vi "TILDAS Prep Line Valves Sequence - 6June22.vi"() -> ()   [LabVIEW 2020]
uses:
  <vilib>/Analysis/baseanly.llb/Mean (DBL).vi
  <vilib>/MakerHub/LINX/Public/Peripherals/Digital/Digital Write 1 Chan.vi
  <vilib>/MakerHub/LINX/Public/Peripherals/Digital/Digital Write N Chans.vi
  <vilib>/MakerHub/LINX/Private/Local IO/LinxDigitalWrite.vi
  <vilib>/MakerHub/LINX/Public/Utilities/Check Channel.vi
  <vilib>/MakerHub/LINX/Public/Utilities/Open Serial.vi
  <vilib>/MakerHub/LINX/Private/Utilties/Generate Error.vi
  <vilib>/MakerHub/LINX/LMH-LINX.lvlib
  <vilib>/Analysis/NI_AALBase.lvlib
panel:
  in  "Stop Loop Fill":bool
  out "Prep. Loop":bool
  in  "Circulation Loop":bool
  in  "Circulation Loop":u8=17
  out "Slosh acc. %":dbl
  out "P frac. slosh":dbl
  out "Rem. slosh frac.":dbl
  out "Exact slosh":dbl
  out "Slosh P (mbar)":dbl
  out "Slosh to do":dbl
  out "No. Slosh":dbl
  out "Final P Accuracy (%)":dbl
  in  "Stop Sample Pressure":bool
  out "Final P (mbar)":dbl
  out "Final Target P (mbar)":dbl
  out "Seq. Finished":bool
  out "Inject GB":bool
  in  "Test":bool
  in  "Stop Pump Over":bool
  out "umol CO2":dbl format="%0.3f"
  out "Dil. Target P (mbar)":dbl format="%0.3f"
  out "Thawing":bool
  out "Diluting":bool
  out "Cryo-pull":bool
  out "Dilution P (mbar)":dbl
  in  "Stop Dilution":bool
  out "Dil. i":i32
  in  "Valve 2":u8=2
  in  "V2":bool
  in  "Valve 3":u8=3
  in  "V3":bool
  in  "Valve 1":u8=4
  in  "V1":bool
  in  "Valve 5":u8=5
  in  "V5":bool
  in  "Valve 6":u8=6
  in  "V6":bool
  in  "Valve 4":u8=7
  in  "V4":bool
  in  "Valve 16":u8=8
  in  "V16":bool
  in  "Valve 8":u8=10
  in  "V8":bool
  in  "Dewar":u8=11
  in  "D":bool
  in  "Valve 19":u8=12
  in  "V19":bool
  in  "Valve 7":u8=13
  in  "V7":bool
  in  "Valve 18":u8=14
  in  "V18":bool
  in  "Valve 17":u8=16
  in  "V21":bool
  in  "Valve 21":u8=15
  in  "V17":bool
  in  "Valve 20":u8=17
  in  "V20":bool
  in  "stop (F)":bool caption="Gauge Signal"
  out "Wika (Avg)":dynamicdata(graph)
  out "?":dbl(knob) scale=0.001..1000.0
  out "?":dynamicdata(graph)
  out "Agilent":dbl(knob) scale=0.001..10.0
  out "Agilent (Torr)":dbl
  out "Pressure (mbar)":dbl format="%0.3f"
  out "V":dbl format="%#_4g"
  out "Thaw Yield (torr)":dbl
  out "Open Flask":bool
  out "Break Tube":bool
  in  "Temp (K)":dbl
  out "Analysis Start Time":timestamp format="%<%H:%M:%S\n%x>T"
  out "Current Time":timestamp format="%<%H:%M:%S>T"
  in  "End Program":bool caption="Press & Hold"
  in  "GO!!!!":bool
  in  "Cracker 3":bool
  in  "Cracker 2":bool
  in  "Cracker 1":bool
  in  "Standby Mode":bool
  out "Cracker":bool
  in  "Cracker Enabled":bool
  in  "Flask Enabled":bool
  in  "Carbonate Enabled":bool
  out "Atm Flask":bool
  out "Carbonate Sam":bool
  in  "Start Sequence":bool
  # "List of proper DO channel values: \nV1 - 4\nV2 - 2                     Slosh stats\nV3 - 3\nV4 - 7\nV5 - 5\nV6 - 6\nV7 - 13\nV8 - 10\nDewar - 11\nV16 - 8\nV17 - 15\nV18 - 14\nV19 - 12\nV20 - 17\nV21 - 16\nCirculation Loop - 9"
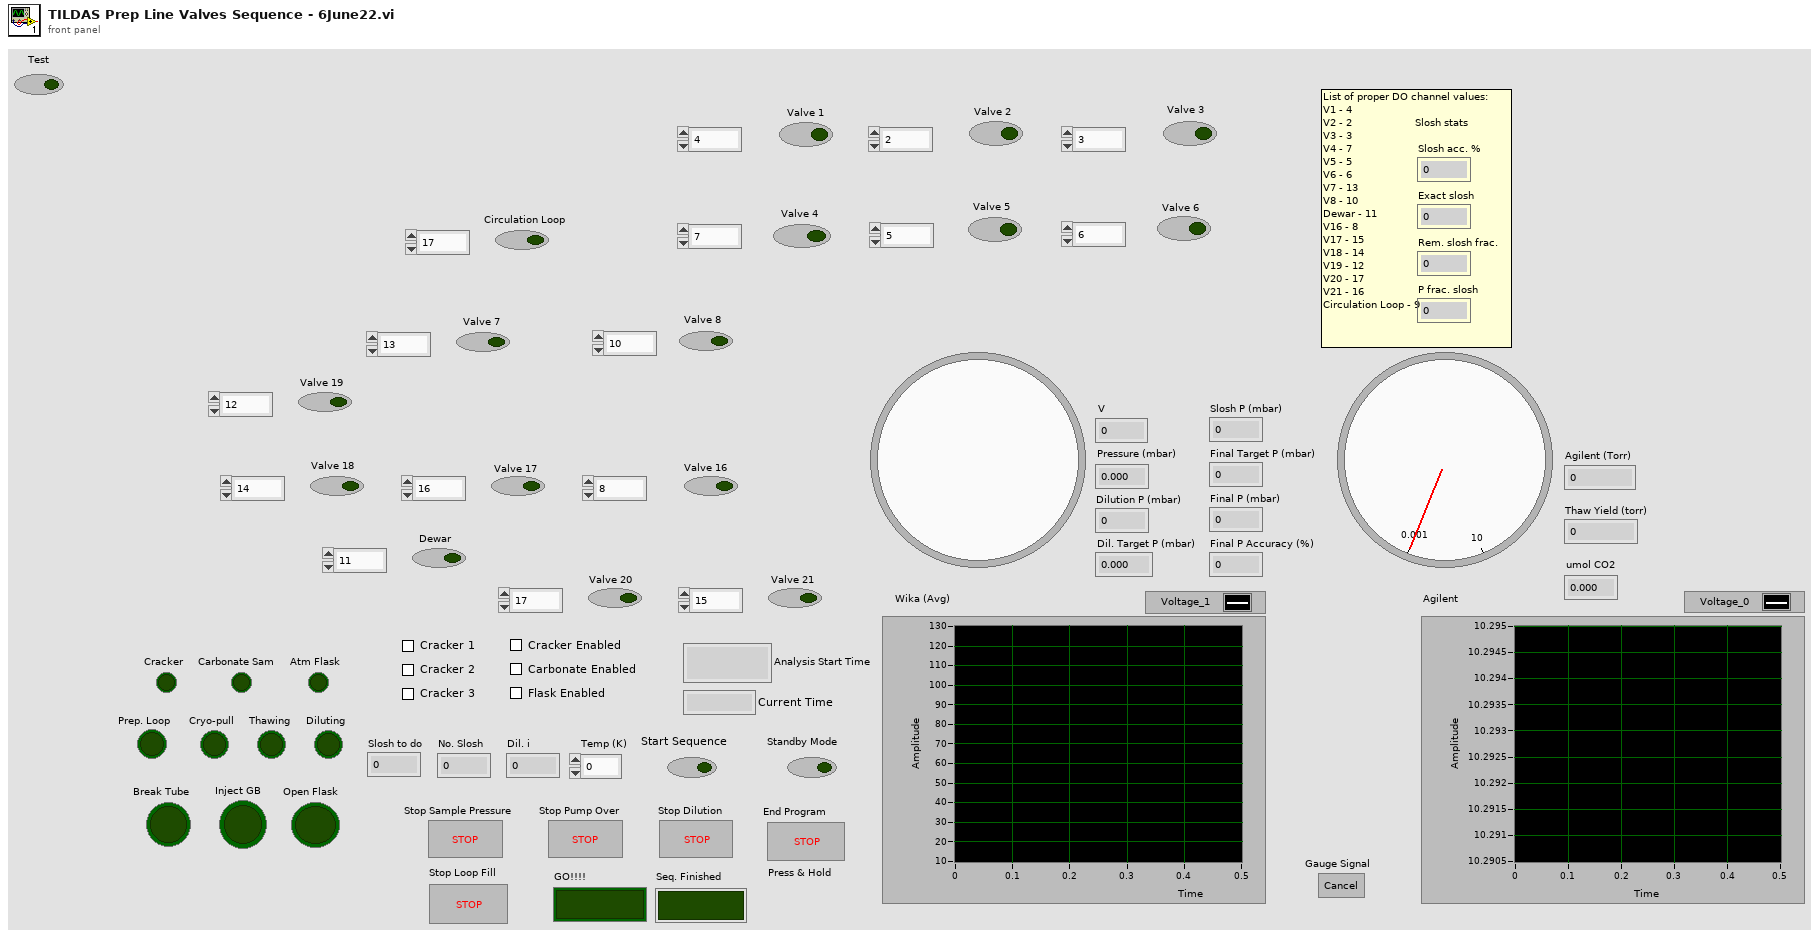
[diagram p1: front panel]
types:
  T1 = typedef "LMH-LINX.lvlib/LINX Ref.ctl" = cluster{"IO":T2, "Interface":T3, "LINX Device Config":T4}
  T2 = typedef "LMH-LINX.lvlib/Platform.ctl" = enum16{"Remote", "Local"}
  T3 = typedef "LMH-LINX.lvlib/Interface.ctl" = enum16{"Serial", "TCP"}
  T4 = typedef "LMH-LINX.lvlib/Device.lvlib/LINX Device Config.ctl" = cluster{"Interface":T3, "COM Port":refnum<visa-resource-name>, "TCP Configuration":T5, "Device Family":u8, "Device ID":u8, "Device Name":string, "TCP Ref":refnum<k5>, "Channels":T6}
  T5 = typedef "LMH-LINX.lvlib/Device.lvlib/TCP Config.ctl" = cluster{"IP Address":string, "Port":u16}
  T6 = typedef "LMH-LINX.lvlib/Channels.ctl" = cluster{"DI":u8[], "DO":u8[], "AI":u8[], "AO":u8[], "PWM":u8[], "QE":u8[], "UART":u8[], "I2C 2":u8[], "SPI":u8[], "CAN":u8[], "Servo":u8[], "AI Ref (V)":dbl, "AI Resolution (Bits)":u8, "AO Ref (V)":dbl, "AO Resolution (Bits)":u8}
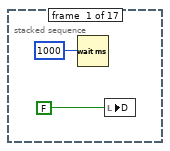
[diagram p6: hidden frame]
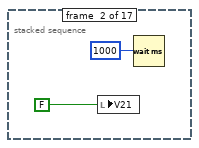
[diagram p7: hidden frame]
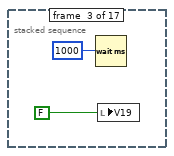
[diagram p8: hidden frame]
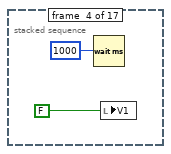
[diagram p9: hidden frame]
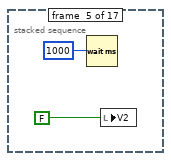
[diagram p10: hidden frame]
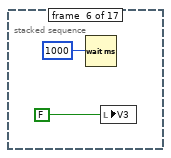
[diagram p11: hidden frame]
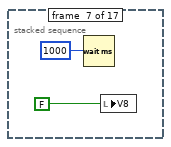
[diagram p12: hidden frame]
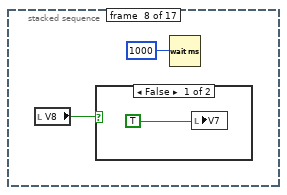
[diagram p13: hidden frame]
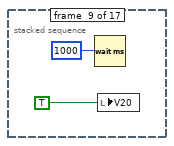
[diagram p15: hidden frame]
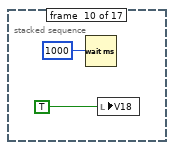
[diagram p16: hidden frame]
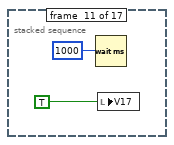
[diagram p17: hidden frame]
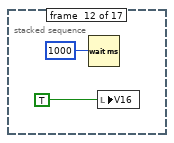
[diagram p18: hidden frame]
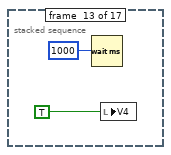
[diagram p19: hidden frame]
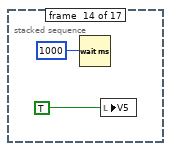
[diagram p20: hidden frame]
diagram:
  # "Standby mode: \nV21 - C\nV19 - C\nV1 - C\nV2 - C\nV3 - C\nV8 - C\nV7 - O\nV20 - O\nV18 - O\nV17 - O\nV16 - O\nV4 - O\nV5 - O\nV6 - O\nTurn off all \nindicators/controls"
  n1 = control-ref of="Standby Mode"() -> (w18:refnum<vi>)
  n2 = register-events(w18) -> (reference out=w17:refnum<event-registration>, error out=w7:errorcluster)  [unwired: 2 in]
  n3 = while {
    tunnel: w17 -> [w29]
    tunnel: [w28] -> w16
    tunnel: w7 -> [w25]
    tunnel: [w25] -> w8
    stop <- w26 stop-if-true
    n4 = event shown="[0] \"Standby Mode\": Value Change" {
      selector: w29 -> [_]
      dyn-events: [_] -> w28
      timeout: _ -> [_]
      event "Standby Mode": Value Change {
        n5 = event-data() -> ()  [unwired: 1 in, 6 out]
        n6 = stacked-sequence {
          frame #0 {
            n7 = Wait (ms)(milliseconds to wait=1000) -> ()  [unwired: 1 out]
            n8 = local write "D"(FALSE) -> ()
          }
          frame #1 {
            n9 = local write "V21"(FALSE) -> ()
            n10 = Wait (ms)(milliseconds to wait=1000) -> ()  [unwired: 1 out]
          }
          frame #2 {
            n11 = Wait (ms)(milliseconds to wait=1000) -> ()  [unwired: 1 out]
            n12 = local write "V19"(FALSE) -> ()
          }
          frame #3 {
            n13 = Wait (ms)(milliseconds to wait=1000) -> ()  [unwired: 1 out]
            n14 = local write "V1"(FALSE) -> ()
          }
          frame #4 {
            n15 = Wait (ms)(milliseconds to wait=1000) -> ()  [unwired: 1 out]
            n16 = local write "V2"(FALSE) -> ()
          }
          frame #5 {
            n17 = Wait (ms)(milliseconds to wait=1000) -> ()  [unwired: 1 out]
            n18 = local write "V3"(FALSE) -> ()
          }
          frame #6 {
            n19 = Wait (ms)(milliseconds to wait=1000) -> ()  [unwired: 1 out]
            n20 = local write "V8"(FALSE) -> ()
          }
          frame #7 {
            n21 = local read "V8"() -> (w45:bool)
            n22 = case shown="False" w45 {
              frame False {
                n23 = local write "V7"(TRUE) -> ()
              }
              frame True {
              }
            }
            n24 = Wait (ms)(milliseconds to wait=1000) -> ()  [unwired: 1 out]
          }
          frame #8 {
            n25 = Wait (ms)(milliseconds to wait=1000) -> ()  [unwired: 1 out]
            n26 = local write "V20"(TRUE) -> ()
          }
          frame #9 {
            n27 = Wait (ms)(milliseconds to wait=1000) -> ()  [unwired: 1 out]
            n28 = local write "V18"(TRUE) -> ()
          }
          frame #10 {
            n29 = Wait (ms)(milliseconds to wait=1000) -> ()  [unwired: 1 out]
            n30 = local write "V17"(TRUE) -> ()
          }
          frame #11 {
            n31 = Wait (ms)(milliseconds to wait=1000) -> ()  [unwired: 1 out]
            n32 = local write "V16"(TRUE) -> ()
          }
          frame #12 {
            n33 = Wait (ms)(milliseconds to wait=1000) -> ()  [unwired: 1 out]
            n34 = local write "V4"(TRUE) -> ()
          }
          frame #13 {
            n35 = Wait (ms)(milliseconds to wait=1000) -> ()  [unwired: 1 out]
            n36 = local write "V5"(TRUE) -> ()
          }
          frame #14 {
            n37 = Wait (ms)(milliseconds to wait=1000) -> ()  [unwired: 1 out]
            n38 = local write "V6"(TRUE) -> ()
          }
          frame #15 {
            w61 = FALSE
            n39 = local write "Break Tube"(w61) -> ()
            n40 = local write "Start Sequence"(w61) -> ()
            n41 = local write "Carbonate Enabled"(w61) -> ()
            n42 = local write "Flask Enabled"(w61) -> ()
            n43 = local write "Standby Mode"(w61) -> ()
            n44 = local write "Open Flask"(w61) -> ()
            n45 = local write "Cracker Enabled"(w61) -> ()
            n46 = local write "Carbonate Sam"(w61) -> ()
            n47 = local write "Cracker 1"(w61) -> ()
            n48 = local write "Atm Flask"(w61) -> ()
            n49 = local write "Cracker 2"(w61) -> ()
            n50 = local write "Cracker 3"(w61) -> ()
            n51 = local write "Cracker"(w61) -> ()
            n52 = local write "GO!!!!"(w61) -> ()
          }
          frame #16 {
            n53 = local write "Dil. Target P (mbar)"(0.0 ("Target P (mbar)")) -> ()
            n54 = local write "umol CO2"(0.0 ("umol CO2")) -> ()
            n55 = local write "Thaw Yield (torr)"(0.0 ("Thaw Yield (torr)")) -> ()
            n56 = local write "Dilution P (mbar)"(0.0 ("Dilution P (mbar)")) -> ()
            n57 = local write "Dil. i"(0 ("Dil. i")) -> ()
          }
        }
      }
    }
    n58 = Wait (ms)(milliseconds to wait=u32 111) -> ()  [unwired: 1 out]
    n59 = local read "End Program"() -> (w26:bool)
  }
  n60 = control-ref of="Start Sequence"() -> (w12:refnum<vi>)
  n61 = register-events(w12) -> (reference out=w13:refnum<event-registration>, error out=w9:errorcluster)  [unwired: 2 in]
  n62 = Unregister For Events(event registration refnum=w16, error in=w8) -> (error out=w15:errorcluster)
  n63 = call <vilib>:"Simple Error Handler.vi"("error in (no error)"=w15) -> ()  [unwired: 4 in, 5 out]
  n64 = call-poly <vilib>:"Open.vi"("Serial Port"=refnum<visa-resource-name> "COM3") -> ("Error Out"=w23:errorcluster, "LINX Resource"=w22:T1)  [unwired: 8 in, 1 out]
  n65 = while {
    tunnel: w13 -> [w70]
    tunnel: [w69] -> w11
    tunnel: w9 -> [w68]
    tunnel: [w67] -> w10
    stop <- w71 stop-if-true
    n66 = event shown="[0] \"Start Sequence\": Value Change" {
      selector: w70 -> [_]
      dyn-events: [_] -> w69
      timeout: _ -> [_]
      tunnel: w68 -> [w73]
      tunnel: [w73] -> w67
      event "Start Sequence": Value Change {
        # "Just lights - used to verify start of sequence"
        # "Atm flask sequence"
        # "Carbonate sequence"
        # "Crackers sequence"
        n67 = event-data() -> ()  [unwired: 1 in, 6 out]
        n68 = local read "Carbonate Enabled"() -> (w87:bool)
        n69 = local read "Flask Enabled"() -> (w86:bool)
        n70 = local read "Cracker Enabled"() -> (w84:bool)
        n71 = local read "Carbonate Enabled"() -> (w79:bool)
        n72 = local read "Cracker Enabled"() -> (w80:bool)
        n73 = local read "Start Sequence"() -> (w82:bool)
        n74 = local read "Flask Enabled"() -> (w78:bool)
        n75 = Or(x=w87, y=w86) -> (x .or. y?=w85:bool)
        n76 = Or(x=w84, y=w85) -> (x .or. y?=w83:bool)
        n77 = And(x=w82, y=w83) -> (x .and. y?=w81:bool)
        n78 = case shown="True" w80 {
          frame False {
          }
          frame True {
            n79 = local write "Carbonate Sam"(FALSE) -> ()
            n80 = local write "Atm Flask"(FALSE) -> ()
            n81 = local write "Cracker"(TRUE) -> ()
          }
        }
        n82 = case shown="True" w79 {
          frame False {
          }
          frame True {
            n83 = local write "Carbonate Sam"(TRUE) -> ()
            n84 = local write "Atm Flask"(FALSE) -> ()
            n85 = local write "Cracker"(FALSE) -> ()
          }
        }
        n86 = case shown="True" w78 {
          frame False {
          }
          frame True {
            n87 = local write "Carbonate Sam"(FALSE) -> ()
            n88 = local write "Atm Flask"(TRUE) -> ()
            n89 = local write "Cracker"(FALSE) -> ()
          }
        }
        n90 = case shown="True" w81 {
          selector: w81 -> [w1641 w1643]
          tunnel: [w1641 w1643] -> w74
          frame False {
            n91 = call "Display Message to User13"() -> ()  [unwired: 10 in, 2 out]
          }
          frame True {
            n92 = flat-sequence {
              frame #0 {
                n93 = Get Date/Time In Seconds() -> (seconds since 1Jan1904=→"Analysis Start Time":timestamp)
              }
              frame #1 {
                n94 = local write "GO!!!!"(TRUE) -> ()
              }
            }
            n95 = Wait (ms)(milliseconds to wait=u32 1000) -> ()  [unwired: 1 out]
          }
        }
        n96 = case shown="True" w74 {
          selector: w74 -> [w99 _]
          tunnel: [w99 w103] -> w76
          frame False {
          }
          frame True {
            n97 = local read "Carbonate Sam"() -> (w100:bool)
            n98 = local read "Start Sequence"() -> (w101:bool)
            n99 = And(x=w101, y=w100) -> (x .and. y?=w102:bool)
            n100 = case shown="True" w102 {
              tunnel: [w106 w107] -> w103
              frame False {
                n101 = local read "Carbonate Enabled"() -> (w104:bool)
                n102 = local read "GO!!!!"() -> (w105:bool)
                n103 = And(x=w105, y=w104) -> (x .and. y?=w106:bool)
              }
              frame True {
                n104 = local read "Carbonate Enabled"() -> (w108:bool)
                n105 = local read "GO!!!!"() -> (w109:bool)
                n106 = And(x=w109, y=w108) -> (x .and. y?=w107:bool)
              }
            }
          }
        }
        n107 = case shown="True" w74 {
          selector: w74 -> [w110 _]
          tunnel: [w110 w114] -> w75
          frame False {
          }
          frame True {
            n108 = local read "Start Sequence"() -> (w112:bool)
            n109 = local read "Cracker"() -> (w111:bool)
            n110 = And(x=w112, y=w111) -> (x .and. y?=w113:bool)
            n111 = case shown="True" w113 {
              tunnel: [w117 w118] -> w114
              frame False {
                n112 = local read "Carbonate Enabled"() -> (w115:bool)
                n113 = local read "GO!!!!"() -> (w116:bool)
                n114 = And(x=w116, y=w115) -> (x .and. y?=w117:bool)
              }
              frame True {
                n115 = local read "Cracker Enabled"() -> (w119:bool)
                n116 = local read "GO!!!!"() -> (w120:bool)
                n117 = And(x=w120, y=w119) -> (x .and. y?=w118:bool)
              }
            }
          }
        }
        n118 = case shown="True" w74 {
          selector: w74 -> [w88 _]
          tunnel: [w88 w92] -> w77
          frame False {
          }
          frame True {
            n119 = local read "Start Sequence"() -> (w90:bool)
            n120 = local read "Atm Flask"() -> (w89:bool)
            n121 = And(x=w90, y=w89) -> (x .and. y?=w91:bool)
            n122 = case shown="True" w91 {
              tunnel: [w95 w96] -> w92
              frame False {
                n123 = local read "Flask Enabled"() -> (w93:bool)
                n124 = local read "GO!!!!"() -> (w94:bool)
                n125 = And(x=w94, y=w93) -> (x .and. y?=w95:bool)
              }
              frame True {
                n126 = local read "Flask Enabled"() -> (w97:bool)
                n127 = local read "GO!!!!"() -> (w98:bool)
                n128 = And(x=w98, y=w97) -> (x .and. y?=w96:bool)
              }
            }
          }
        }
        n129 = case shown="True" w75 {
          frame False {
          }
          frame True {
            # "Pretty much if something is wrong from the start it won't pass this 2 second check and save the trouble of dealing with it"
            # "If Current Time is within a 2 second window of \nAnalysis Start Time, run this. If not, do nothing."
            n130 = local read "Analysis Start Time"() -> (w725:timestamp)
            n131 = local read "Current Time"() -> (w724:timestamp)
            n132 = To Double Precision Float(number=w725) -> (double precision float=w723:dbl)
            n133 = To Double Precision Float(number=w724) -> (double precision float=w726:dbl)
            n134 = Add(x=w723, y=2.0) -> (x+y=w728:dbl)
            n135 = Greater?(x=w726, y=w723) -> (0:w729:bool)
            n136 = Less?(x=w726, y=w728) -> (x < y?=w730:bool)
            n137 = And(x=w729, y=w730) -> (x .and. y?=w722:bool)
            n138 = case shown="True" w722 {
              frame False {
              }
              frame True {
                # "Cracker 1: V1-V4\nCracker 2: V2-V5\nCracker 3: V3-V6"
                # "Assuming stby start"
                # "Read cracker selected"
                # "Cracker 1: V1-V4\nCracker 2: V2-V5\nCracker 3: V3-V6"
                # "Assuming stby start"
                # "Read cracker selected"
                n139 = local read "Cracker 1"() -> (w731:bool)
                n140 = case shown="False" w731 {
                  frame False {
                    # "Cracker 1: V1-V4\nCracker 2: V2-V5\nCracker 3: V3-V6"
                    n141 = local read "Cracker 2"() -> (w732:bool)
                    n142 = case shown="False" w732 {
                      frame False {
                        # "Cracker 1: V1-V4\nCracker 2: V2-V5\nCracker 3: V3-V6"
                        n143 = local read "Cracker 3"() -> (w733:bool)
                        n144 = case shown="True" w733 {
                          frame False {
                            n145 = call "Display Message to User12"() -> ()  [unwired: 10 in, 2 out]
                          }
                          frame True {
                            n146 = stacked-sequence {
                              tunnel: [_ _ _ _ w759 _ _ _ _ _ _ _ _ _ _ _ _ _ _ _ _ _ _ _ _ _ _ _ _ _ _ _ _ _ _ _ _ _ _ _ _ _ _ _ _ _ _ _ _ _ _ _ _ _ _ _ _ _ _ _ _] -> _
                              tunnel: [_ _ _ _ _ _ _ _ _ _ _ _ _ _ _ _ w789 _ _ _ _ _ _ _ _ _ _ _ _ _ _ _ _ _ _ _ _ _ _ _ _ _ _ _ _ _ _ _ _ _ _ _ _ _ _ _ _ _ _ _ _] -> _
                              tunnel: [_ _ _ _ _ w760 _ _ _ _ _ _ _ _ _ _ _ _ _ _ _ _ _ _ _ _ _ _ _ _ _ _ _ _ _ _ _ _ _ _ _ _ _ _ _ _ _ _ _ _ _ _ _ _ _ _ _ _ _ _ _] -> _
                              tunnel: [_ _ _ _ _ _ _ _ _ _ _ _ _ _ _ _ _ _ _ _ _ _ _ _ _ _ _ _ _ _ _ _ _ _ _ _ _ _ _ _ _ _ _ _ _ _ _ _ _ _ _ _ _ _ _ _ w1024 _ _ _ _] -> _
                              tunnel: [_ _ _ _ _ _ _ _ _ _ _ _ _ _ _ _ _ _ _ _ _ _ _ _ _ _ _ _ _ _ _ _ _ _ _ _ _ _ _ _ _ _ _ _ _ _ _ _ _ _ _ _ _ _ _ _ _ _ w1027 _ _] -> _
                              frame #0 {
                                n147 = local write "Final Target P (mbar)"(0.0) -> ()
                                n148 = local write "Final P Accuracy (%)"(0.0) -> ()
                                n149 = local write "Thaw Yield (torr)"(0.0) -> ()
                                n150 = local write "Final P (mbar)"(0.0) -> ()
                                n151 = local write "Slosh to do"(0.0) -> ()
                                n152 = local write "umol CO2"(0.0) -> ()
                                n153 = local write "No. Slosh"(0.0) -> ()
                                n154 = local write "Dil. i"(0.0) -> ()
                                n155 = local write "Dil. Target P (mbar)"(0.0) -> ()
                                n156 = local write "Dilution P (mbar)"(0.0) -> ()
                                n157 = local write "Rem. slosh frac."(0.0) -> ()
                                n158 = local write "Slosh P (mbar)"(0.0) -> ()
                                n159 = local write "Slosh acc. %"(0.0) -> ()
                                n160 = local write "P frac. slosh"(0.0) -> ()
                                n161 = local write "Exact slosh"(0.0) -> ()
                                n162 = local write "Temp (K)"(294.0) -> ()
                              }
                              frame #1 {
                                # "V18,17,16,20 should all be open to start"
                                # "Open V7"
                                n163 = local write "V7"(TRUE) -> ()
                                n164 = local write "Seq. Finished"(FALSE) -> ()
                                n165 = Wait (ms)(milliseconds to wait=1000) -> ()  [unwired: 1 out]
                              }
                              frame #2 {
                                # "V18,17,16,20 should all be open to start"
                                # "Open V16"
                                n166 = local write "V16"(TRUE) -> ()
                                n167 = Wait (ms)(milliseconds to wait=1000) -> ()  [unwired: 1 out]
                              }
                              frame #3 {
                                # "Close off unselected crackers"
                                n168 = flat-sequence {
                                frame #0 {
                                n169 = local write "V4"(FALSE) -> ()
                                }
                                frame #1 {
                                n170 = Wait (ms)(milliseconds to wait=1000) -> ()  [unwired: 1 out]
                                }
                                frame #2 {
                                n171 = local write "V5"(FALSE) -> ()
                                }
                                }
                                n172 = Wait (ms)(milliseconds to wait=1000) -> ()  [unwired: 1 out]
                              }
                              frame #4 {
                                # "Close flask valves"
                                n173 = call "Prompt User for Input33"() -> ("OK"=w759:bool)  [unwired: 18 in, 1 out]
                              }
                              frame #5 {
                                # "Close crackers and GB manual valves"
                                n174 = call "Prompt User for Input34"() -> ("OK"=w760:bool)  [unwired: 18 in, 1 out]
                              }
                              frame #6 {
                                # "Open Loop"
                                n175 = local write "Circulation Loop"(TRUE) -> ()
                                n176 = local write "Prep. Loop"(TRUE) -> ()
                                n177 = Wait (ms)(milliseconds to wait=1000) -> ()  [unwired: 1 out]
                              }
                              frame #7 {
                                # "22/4/22 - background ~280 mtorr bg"
                                # "Pump Loop for 60sec"
                                n178 = call "Time Delay22"() -> ()  [unwired: 11 in, 1 out]
                              }
                              frame #8 {
                                # "Open V8"
                                n179 = local write "V8"(TRUE) -> ()
                                n180 = Wait (ms)(milliseconds to wait=1000) -> ()  [unwired: 1 out]
                              }
                              frame #9 {
                                # "Close V20"
                                n181 = local write "V20"(FALSE) -> ()
                                n182 = Wait (ms)(milliseconds to wait=1000) -> ()  [unwired: 1 out]
                              }
                              frame #10 {
                                # "Open V21"
                                n183 = local write "V21"(TRUE) -> ()
                                n184 = Wait (ms)(milliseconds to wait=1000) -> ()  [unwired: 1 out]
                              }
                              frame #11 {
                                # "When P > 1300 in Loop close V21"
                                n185 = while {
                                shift-right: [w771] -> _
                                shift-left: _ -> [_]
                                stop <- w772 stop-if-true
                                n186 = local read "Pressure (mbar)"() -> (w775:dbl)
                                n187 = Wait (ms)(milliseconds to wait=100) -> ()  [unwired: 1 out]
                                n188 = Greater?(x=w775, y=1300.0) -> (0:w774:bool)
                                n189 = case shown="True" w774 {
                                selector: w774 -> [w777 w780]
                                tunnel: [w777 w780] -> w771
                                frame False {
                                }
                                frame True {
                                n190 = local write "Stop Loop Fill"(TRUE) -> ()
                                n191 = local write "V21"(FALSE) -> ()
                                }
                                }
                                n192 = local read "Stop Loop Fill"() -> (w772:bool)
                                }
                                n193 = Wait (ms)(milliseconds to wait=1000) -> ()  [unwired: 1 out]
                              }
                              frame #12 {
                                n194 = call "Prompt User for Input35"() -> ()  [unwired: 18 in, 2 out]
                                n195 = local write "Stop Loop Fill"(FALSE) -> ()
                              }
                              frame #13 {
                                # "Shut Loop"
                                n196 = local write "Circulation Loop"(FALSE) -> ()
                                n197 = local write "Prep. Loop"(FALSE) -> ()
                                n198 = Wait (ms)(milliseconds to wait=1000) -> ()  [unwired: 1 out]
                              }
                              frame #14 {
                                # "Close V8"
                                n199 = local write "V8"(FALSE) -> ()
                                n200 = Wait (ms)(milliseconds to wait=1000) -> ()  [unwired: 1 out]
                              }
                              frame #15 {
                                # "Open V20"
                                n201 = local write "V20"(TRUE) -> ()
                                n202 = Wait (ms)(milliseconds to wait=1000) -> ()  [unwired: 1 out]
                              }
                              frame #16 {
                                # "Open crackers manual valve, close GB manual valve"
                                n203 = call "Prompt User for Input36"() -> ("OK"=w789:bool)  [unwired: 18 in, 1 out]
                              }
                              frame #17 {
                                # "Open V6 - pump out cracker to be used"
                                n204 = local write "V6"(TRUE) -> ()
                                n205 = Wait (ms)(milliseconds to wait=1000) -> ()  [unwired: 1 out]
                              }
                              frame #18 {
                                # "When P < 0,076 torr continue w/ sequence"
                                n206 = while {
                                shift-right: [w793] -> _
                                shift-left: _ -> [_]
                                stop <- w794 stop-if-true
                                n207 = local read "Agilent (Torr)"() -> (w797:dbl)
                                n208 = Wait (ms)(milliseconds to wait=100) -> ()  [unwired: 1 out]
                                n209 = Less?(x=w797, y=0.076) -> (x < y?=w796:bool)
                                n210 = case shown="True" w796 {
                                selector: w796 -> [w799 w801]
                                tunnel: [w799 w801] -> w793
                                frame False {
                                }
                                frame True {
                                n211 = local write "Stop Pump Over"(TRUE) -> ()
                                }
                                }
                                n212 = local read "Stop Pump Over"() -> (w794:bool)
                                }
                                n213 = Wait (ms)(milliseconds to wait=1000) -> ()  [unwired: 1 out]
                              }
                              frame #19 {
                                # "10 extra sec to pump out bottom cracker volume"
                                n214 = local write "Stop Pump Over"(FALSE) -> ()
                                n215 = Wait (ms)(milliseconds to wait=10000) -> ()  [unwired: 1 out]
                              }
                              frame #20 {
                                # "Redundant just in case"
                                # "Close V4"
                                n216 = local write "V4"(FALSE) -> ()
                                n217 = Wait (ms)(milliseconds to wait=1000) -> ()  [unwired: 1 out]
                              }
                              frame #21 {
                                # "Redundant just in case"
                                # "Close V5"
                                n218 = local write "V5"(FALSE) -> ()
                                n219 = Wait (ms)(milliseconds to wait=1000) -> ()  [unwired: 1 out]
                              }
                              frame #22 {
                                # "Dewar up"
                                n220 = local write "D"(TRUE) -> ()
                                n221 = Wait (ms)(milliseconds to wait=1000) -> ()  [unwired: 1 out]
                              }
                              frame #23 {
                                # "15 sec for trap to cool"
                                n222 = Wait (ms)(milliseconds to wait=15000) -> ()  [unwired: 1 out]
                              }
                              frame #24 {
                                # "Close V18"
                                n223 = local write "V18"(FALSE) -> ()
                                n224 = Wait (ms)(milliseconds to wait=1000) -> ()  [unwired: 1 out]
                              }
                              frame #25 {
                                # "Break tube light on"
                                n225 = local write "Break Tube"(TRUE) -> ()
                                n226 = Wait (ms)(milliseconds to wait=1000) -> ()  [unwired: 1 out]
                              }
                              frame #26 {
                                # "10 min cryo-pull"
                                n227 = local write "Cryo-pull"(TRUE) -> ()
                                n228 = call "Cryo pull t7"() -> ()  [unwired: 11 in, 1 out]
                              }
                              frame #27 {
                                # "Open V18 - pump over"
                                n229 = local write "V18"(TRUE) -> ()
                                n230 = Wait (ms)(milliseconds to wait=5000) -> ()  [unwired: 1 out]
                              }
                              frame #28 {
                                # "When P < 0.075 torr close LN2 trap"
                                n231 = while {
                                shift-right: [w820] -> _
                                shift-left: _ -> [_]
                                stop <- w822 stop-if-true
                                n232 = local read "Agilent (Torr)"() -> (w825:dbl)
                                n233 = Wait (ms)(milliseconds to wait=100) -> ()  [unwired: 1 out]
                                n234 = Less?(x=w825, y=0.075) -> (x < y?=w823:bool)
                                n235 = case shown="True" w823 {
                                selector: w823 -> [w826 w827]
                                tunnel: [w826 w827] -> w820
                                frame False {
                                }
                                frame True {
                                w829 = FALSE
                                n236 = local write "V17"(w829) -> ()
                                n237 = local write "V18"(w829) -> ()
                                n238 = local write "Stop Pump Over"(TRUE) -> ()
                                }
                                }
                                n239 = local read "Stop Pump Over"() -> (w822:bool)
                                }
                                n240 = local write "Cryo-pull"(FALSE) -> ()
                                n241 = Wait (ms)(milliseconds to wait=1000) -> ()  [unwired: 1 out]
                              }
                              frame #29 {
                                # "Close V16"
                                n242 = local write "Stop Pump Over"(FALSE) -> ()
                                n243 = local write "V16"(FALSE) -> ()
                                n244 = Wait (ms)(milliseconds to wait=1000) -> ()  [unwired: 1 out]
                              }
                              frame #30 {
                                # "Close V6"
                                n245 = local write "V6"(FALSE) -> ()
                                n246 = Wait (ms)(milliseconds to wait=1000) -> ()  [unwired: 1 out]
                              }
                              frame #31 {
                                # "Dewar down"
                                n247 = local write "D"(FALSE) -> ()
                                n248 = Wait (ms)(milliseconds to wait=1000) -> ()  [unwired: 1 out]
                              }
                              frame #32 {
                                # "6 minute thaw"
                                n249 = call "Time Delay23"() -> ()  [unwired: 11 in, 1 out]
                                n250 = local write "Thawing"(TRUE) -> ()
                                n251 = call "Display Message to User15"() -> ()  [unwired: 10 in, 2 out]
                              }
                              frame #33 {
                                n252 = call "Display Message to User16"() -> ()  [unwired: 10 in, 2 out]
                              }
                              frame #34 {
                                # "Read thaw P on Agilent - calculate umol CO2 trapped"
                                n253 = local write "Thawing"(FALSE) -> ()
                                n254 = flat-sequence {
                                frame #0 {
                                n255 = local read "Agilent (Torr)"() -> (w841:dbl)
                                n256 = local write "Thaw Yield (torr)"(w841) -> ()
                                n257 = Wait (ms)(milliseconds to wait=200) -> ()  [unwired: 1 out]
                                }
                                frame #1 {
                                # "mol CO2"
                                # "''Cast base units''"
                                # "R"
                                # "V LN2, in m3"
                                # "torr to Pa"
                                n258 = local read "Thaw Yield (torr)"() -> (w849:dbl)
                                n259 = local read "Temp (K)"() -> (w842:dbl)
                                n260 = Cast Unit Bases(0:dbl[unit] 8.3144598) -> (2:w843:dbl)  [unwired: 1 in]
                                n261 = Multiply(x=w849, y=133.3223684211) -> (x*y=w848:dbl)
                                n262 = Multiply(x=w843, y=w842) -> (x*y=w847:dbl)
                                n263 = Multiply(x=w848, y=6.1e-05) -> (x*y=w853:dbl)
                                n264 = Divide(x=w853, y=w847) -> (x/y=w846:dbl)
                                n265 = Multiply(x=1000000.0, y=w846) -> (x*y=w844:dbl)
                                n266 = local write "umol CO2"(w844) -> ()
                                }
                                }
                                n267 = Wait (ms)(milliseconds to wait=500) -> ()  [unwired: 1 out]
                              }
                              frame #35 {
                                # "P for 400ppm"
                                # "22/4/22\nOffset \nfor extra\nN2 from \nloop"
                                # "Calculate and store Target P"
                                # "''Cast base units''"
                                # "R"
                                # "''Cast base units''"
                                # "R"
                                # "PV=nrt\nP - Pa\nV - m3\nn - mol\nR - \nT - K"
                                # "Pa to mbar"
                                # "P = nRT/V"
                                # "Pa"
                                # "mol N2 to dilute"
                                # "V LN2, flask, bellow in m3"
                                # "ppm"
                                # "n mol N2 = x mol CO2/0.000400"
                                # "0.000400 = x mol CO2/n mol N2"
                                # "mol CO2"
                                # "V LN2, in m3"
                                # "torr to Pa"
                                n268 = local read "Thaw Yield (torr)"() -> (w873:dbl)
                                n269 = local read "Temp (K)"() -> (w857:dbl)
                                n270 = Subtract(x=w873, y=0.2) -> (x-y=w872:dbl)
                                n271 = Cast Unit Bases(0:dbl[unit] 8.3144598) -> (2:w864:dbl)  [unwired: 1 in]
                                n272 = Multiply(x=w872, y=133.3223684211) -> (x*y=w855:dbl)
                                n273 = Multiply(x=w864, y=w857) -> (x*y=w856:dbl)
                                n274 = Multiply(x=w855, y=6.1e-05) -> (x*y=w854:dbl)
                                n275 = Divide(x=w854, y=w856) -> (x/y=w861:dbl)
                                n276 = Divide(x=w861, y=0.0004) -> (x/y=w875:dbl)
                                n277 = Cast Unit Bases(0:dbl[unit] 8.3144598) -> (2:w863:dbl)  [unwired: 1 in]
                                n278 = local read "Temp (K)"() -> (w860:dbl)
                                n279 = Multiply(x=w863, y=w875) -> (x*y=w859:dbl)
                                n280 = Multiply(x=w860, y=w859) -> (x*y=w858:dbl)
                                n281 = Divide(x=w858, y=0.000687) -> (x/y=w862:dbl)
                                n282 = Multiply(x=0.01, y=w862) -> (x*y=w876:dbl)
                                n283 = local write "Final Target P (mbar)"(w876) -> ()
                                n284 = Wait (ms)(milliseconds to wait=200) -> ()  [unwired: 1 out]
                              }
                              frame #36 {
                                # "Calculate Dilution Target Pressure in prep for final expansion"
                                # "Dil. TP fills full MV, V17 closes\n101ml pumped away (all but flask)\n586ml @ Dil. TP expands to 687ml\n--> 687ml @ Final P (P for 400ppm)"
                                # "P1V1 = P2V2\nDTP*586ml = TFP*687ml\nDTP = (FP*687)/586"
                                n285 = local read "Final Target P (mbar)"() -> (w879:dbl)
                                n286 = Multiply(x=w879, y=687.0) -> (x*y=w880:dbl)
                                n287 = Divide(x=w880, y=586.0) -> (x/y=w882:dbl)
                                n288 = local write "Dil. Target P (mbar)"(w882) -> ()
                                n289 = Wait (ms)(milliseconds to wait=200) -> ()  [unwired: 1 out]
                              }
                              frame #37 {
                                # "22/2/22\nAvg of n=2 1500 mbar auto test sloshes:\nn = 3E-6x^2 + 0,003x + 0,0254"
                                # "21/2/22\n1400 mbar auto test sloshes:\nn = 3E-6x^2 + 0,0033x + 0,0268\nn        x (P mbar)\n0        0\n1        232\n2        430\n3        569\n4        733\n5        847"
                                # "8/2/22\n1100 mbar manual sloshes:\nn = 1E-5x^2 + 0,0003x + 0,3052\nn        x (P mbar)\n0        0\n1        205\n2        345\n3        477\n4        587\n5        678\n6        755\n7        819\n8        872\n9        916\n10      951\n11      981"
                                n290 = flat-sequence {
                                frame #0 {
                                # "Currently using avg curve for (Avg(Avg(1500x2),1400))\nn = 3E-6x^2 + 0.0031x + 0.0261"
                                # "Given Dilution Target Pressure, calculate how many sloshes it would take to get \nthe pressure in the full MV to that pressure."
                                n291 = local read "Dil. Target P (mbar)"() -> (w895:dbl)
                                n292 = local read "Dil. Target P (mbar)"() -> (w893:dbl)
                                n293 = Square(x=w895) -> (x^2=w894:dbl)
                                n294 = Multiply(x=3e-06, y=w894) -> (x*y=w891:dbl)
                                n295 = Multiply(x=w893, y=0.0031) -> (x*y=w892:dbl)
                                n296 = Add(x=w891, y=w892) -> (x+y=w890:dbl)
                                n297 = Add(x=w890, y=0.0261) -> (x+y=w886:dbl)
                                n298 = local write "Exact slosh"(w886) -> ()
                                n299 = Wait (ms)(milliseconds to wait=100) -> ()  [unwired: 1 out]
                                }
                                frame #1 {
                                # "Now take that calculated number of \nsloshes and round down to nearest integer."
                                n300 = local read "Exact slosh"() -> (w897:dbl)
                                n301 = Round Toward -Infinity(1:w897) -> (0:w898:dbl)
                                n302 = local write "Slosh to do"(w898) -> ()
                                n303 = Wait (ms)(milliseconds to wait=100) -> ()  [unwired: 1 out]
                                }
                                frame #2 {
                                n304 = local read "Exact slosh"() -> (w901:dbl)
                                n305 = local read "Slosh to do"() -> (w900:dbl)
                                n306 = Subtract(x=w901, y=w900) -> (x-y=w902:dbl)
                                n307 = local write "Rem. slosh frac."(w902) -> ()
                                n308 = Wait (ms)(milliseconds to wait=100) -> ()  [unwired: 1 out]
                                }
                                frame #3 {
                                n309 = local read "Rem. slosh frac."() -> (w906:dbl)
                                n310 = Multiply(x=1450.0, y=w906) -> (x*y=w905:dbl)
                                n311 = local write "P frac. slosh"(w905) -> ()
                                n312 = Wait (ms)(milliseconds to wait=100) -> ()  [unwired: 1 out]
                                }
                                }
                                n313 = Wait (ms)(milliseconds to wait=200) -> ()  [unwired: 1 out]
                              }
                              frame #38 {
                                # "P should be something like 250mtor (V LN2 ~1/10 of V LN2 + flask)"
                                # "Open, Close V17 - pure CO2 expansion into flask\nEqual concentration of CO2 in LN2, flask, and H of V16/V17"
                                n314 = flat-sequence {
                                frame #0 {
                                n315 = local write "V17"(TRUE) -> ()
                                }
                                frame #1 {
                                n316 = Wait (ms)(milliseconds to wait=u32 40000) -> ()  [unwired: 1 out]
                                }
                                frame #2 {
                                n317 = local write "V17"(FALSE) -> ()
                                }
                                }
                                n318 = Wait (ms)(milliseconds to wait=1000) -> ()  [unwired: 1 out]
                              }
                              frame #39 {
                                # "Close V20"
                                n319 = local write "V20"(FALSE) -> ()
                                n320 = Wait (ms)(milliseconds to wait=1000) -> ()  [unwired: 1 out]
                              }
                              frame #40 {
                                # "Open V8 - begin dilution steps"
                                n321 = local write "Diluting"(TRUE) -> ()
                                n322 = local write "V8"(TRUE) -> ()
                                n323 = Wait (ms)(milliseconds to wait=1000) -> ()  [unwired: 1 out]
                              }
                              frame #41 {
                                # "Open V21"
                                n324 = local write "V21"(TRUE) -> ()
                                n325 = Wait (ms)(milliseconds to wait=1000) -> ()  [unwired: 1 out]
                              }
                              frame #42 {
                                # "Build P in bellow before introducing to LN2 trap w/ sample"
                                n326 = call "Pressurize in LN16"() -> ()  [unwired: 11 in, 1 out]
                              }
                              frame #43 {
                                # "Open V18"
                                n327 = local write "V18"(TRUE) -> ()
                                n328 = Wait (ms)(milliseconds to wait=1000) -> ()  [unwired: 1 out]
                              }
                              frame #44 {
                                n329 = local read "Slosh to do"() -> (w920:dbl)
                                n330 = for {
                                N: w920 -> [_]
                                n331 = flat-sequence {
                                frame #0 {
                                n332 = while {
                                shift-right: [w922] -> _
                                shift-left: _ -> [_]
                                stop <- w923 stop-if-true
                                # "Greater difference in P causes more \nturbulent mixing when expanded into flask"
                                # "When P in bellow + LN2 is > 1450mbar, Open V17"
                                n333 = local read "Pressure (mbar)"() -> (w925:dbl)
                                n334 = Wait (ms)(milliseconds to wait=100) -> ()  [unwired: 1 out]
                                n335 = Greater?(x=w925, y=1450.0) -> (0:w926:bool)
                                n336 = case shown="True" w926 {
                                selector: w926 -> [w927 w929]
                                tunnel: [w927 w929] -> w922
                                frame False {
                                }
                                frame True {
                                n337 = local write "Stop Sample Pressure"(TRUE) -> ()
                                n338 = local write "V17"(TRUE) -> ()
                                }
                                }
                                n339 = local read "Stop Sample Pressure"() -> (w923:bool)
                                }
                                }
                                frame #1 {
                                n340 = local read "No. Slosh"() -> (w931:dbl)
                                n341 = local write "Stop Sample Pressure"(FALSE) -> ()
                                n342 = Increment(x=w931) -> (x+1=w932:dbl)
                                n343 = Wait (ms)(milliseconds to wait=4000) -> ()  [unwired: 1 out]
                                n344 = local write "No. Slosh"(w932) -> ()
                                }
                                frame #2 {
                                n345 = local read "Pressure (mbar)"() -> (w935:dbl)
                                n346 = local write "Slosh P (mbar)"(w935) -> ()
                                n347 = Wait (ms)(milliseconds to wait=1000) -> ()  [unwired: 1 out]
                                }
                                frame #3 {
                                n348 = local write "V17"(FALSE) -> ()
                                n349 = Wait (ms)(milliseconds to wait=1000) -> ()  [unwired: 1 out]
                                }
                                }
                                }
                              }
                              frame #45 {
                                # "Check that the final fractional slosh P \nwill be greater P than what's in the \nflask already. If yes, do fractional slosh; \nif no, skip it and go straight to diluting to DTP."
                                n350 = local read "Slosh P (mbar)"() -> (w941:dbl)
                                n351 = local read "P frac. slosh"() -> (w940:dbl)
                                n352 = Greater Or Equal?(x=w940, y=w941) -> (x >= y?=w939:bool)
                                n353 = case shown="True" w939 {
                                frame False {
                                # "Open V17"
                                n354 = local write "V17"(TRUE) -> ()
                                n355 = local read "Dil. Target P (mbar)"() -> (w943:dbl)
                                n356 = local read "Slosh P (mbar)"() -> (w942:dbl)
                                n357 = Divide(x=w942, y=w943) -> (x/y=w946:dbl)
                                n358 = Multiply(x=w946, y=100.0) -> (x*y=w944:dbl)
                                n359 = local write "Slosh acc. %"(w944) -> ()
                                n360 = Wait (ms)(milliseconds to wait=1000) -> ()  [unwired: 1 out]
                                }
                                frame True {
                                # "Last slosh into flask, keep V17 open so dilution loop can start right after"
                                n361 = flat-sequence {
                                frame #0 {
                                n362 = local read "Rem. slosh frac."() -> (w951:dbl)
                                n363 = local read "No. Slosh"() -> (w952:dbl)
                                n364 = Wait (ms)(milliseconds to wait=100) -> ()  [unwired: 1 out]
                                n365 = Add(x=w952, y=w951) -> (x+y=w950:dbl)
                                n366 = local write "Slosh to do"(w950) -> ()
                                }
                                frame #1 {
                                n367 = while {
                                shift-right: [w955] -> _
                                shift-left: _ -> [_]
                                stop <- w957 stop-if-true
                                # "When P in bellow + LN2 is > fractional slosh P, Open V17"
                                n368 = local read "Pressure (mbar)"() -> (w958:dbl)
                                n369 = local read "P frac. slosh"() -> (w953:dbl)
                                n370 = Wait (ms)(milliseconds to wait=100) -> ()  [unwired: 1 out]
                                n371 = Greater Or Equal?(x=w958, y=w953) -> (x >= y?=w956:bool)
                                n372 = case shown="True" w956 {
                                selector: w956 -> [w959 w960]
                                tunnel: [w959 w960] -> w955
                                frame False {
                                }
                                frame True {
                                n373 = local write "Stop Sample Pressure"(TRUE) -> ()
                                n374 = local write "V17"(TRUE) -> ()
                                }
                                }
                                n375 = local read "Stop Sample Pressure"() -> (w957:bool)
                                }
                                }
                                frame #2 {
                                n376 = local read "Rem. slosh frac."() -> (w963:dbl)
                                n377 = local read "No. Slosh"() -> (w964:dbl)
                                n378 = local write "Stop Sample Pressure"(FALSE) -> ()
                                n379 = Add(x=w964, y=w963) -> (x+y=w965:dbl)
                                n380 = Wait (ms)(milliseconds to wait=5000) -> ()  [unwired: 1 out]
                                n381 = local write "No. Slosh"(w965) -> ()
                                }
                                frame #3 {
                                n382 = local read "Pressure (mbar)"() -> (w968:dbl)
                                n383 = local write "Slosh P (mbar)"(w968) -> ()
                                n384 = Wait (ms)(milliseconds to wait=500) -> ()  [unwired: 1 out]
                                }
                                frame #4 {
                                n385 = local read "Slosh P (mbar)"() -> (w971:dbl)
                                n386 = local read "Dil. Target P (mbar)"() -> (w972:dbl)
                                n387 = Divide(x=w971, y=w972) -> (x/y=w975:dbl)
                                n388 = Multiply(x=w975, y=100.0) -> (x*y=w973:dbl)
                                n389 = local write "Slosh acc. %"(w973) -> ()
                                n390 = Wait (ms)(milliseconds to wait=200) -> ()  [unwired: 1 out]
                                }
                                }
                                }
                                }
                              }
                              frame #46 {
                                # "Dil. TP fills full MV, V17 closes\n101ml pumped away (all but flask)\n586ml @ Dil. TP expands to 687ml\n--> 687ml @ Final P (P for 400ppm)"
                                # "Agilent P comes through the DAQ"
                                # "When P Wika = maths for 400ppm dilution, close V8"
                                n391 = local read "Dil. Target P (mbar)"() -> (w978:dbl)
                                n392 = local read "Pressure (mbar)"() -> (w977:dbl)
                                n393 = Greater?(x=w978, y=w977) -> (0:w976:bool)
                                n394 = case shown="True" w976 {
                                frame False {
                                n395 = local write "V17"(FALSE) -> ()
                                n396 = local write "V8"(FALSE) -> ()
                                n397 = call "Display Message to User17"() -> ()  [unwired: 10 in, 2 out]
                                }
                                frame True {
                                n398 = while {
                                shift-right: [w983] -> _
                                shift-left: _ -> [_]
                                i -> [w993]
                                stop <- w994 stop-if-true
                                n399 = local read "Dil. Target P (mbar)"() -> (w991:dbl)
                                n400 = local write "Dil. i"(w993) -> ()
                                n401 = local read "Pressure (mbar)"() -> (w990:dbl)
                                n402 = local read "Pressure (mbar)"() -> (w988:dbl)
                                n403 = Add(x=w988, y=2.0) -> (x+y=w987:dbl)
                                n404 = Subtract(x=w990, y=2.0) -> (x-y=w986:dbl)
                                n405 = Wait (ms)(milliseconds to wait=u32 100) -> ()  [unwired: 1 out]
                                n406 = In Range and Coerce(upper limit=w987, x=w991, lower limit=w986) -> (coerced(x)=w982:dbl, In Range?=w989:bool)
                                n407 = local write "Dilution P (mbar)"(w982) -> ()
                                n408 = case shown="True" w989 {
                                selector: w989 -> [w995 w999]
                                tunnel: [w995 w999] -> w983
                                frame False {
                                }
                                frame True {
                                n409 = local write "V8"(FALSE) -> ()
                                n410 = local write "Stop Dilution"(TRUE) -> ()
                                n411 = local write "V17"(FALSE) -> ()
                                }
                                }
                                n412 = local read "Stop Dilution"() -> (w994:bool)
                                }
                                }
                                }
                                n413 = Wait (ms)(milliseconds to wait=1000) -> ()  [unwired: 1 out]
                              }
                              frame #47 {
                                # "Close V21 - N2 inlet - want to keep this volume under superambient pressure always"
                                # "Flask will be over concentrated in CO2 (hopefully somewhere around 480ppm - cant really check that so it's blind)\n19/1/22, 8:00 - Initial manual test of this measured 472ppm on the Licor. Sample expansion and re-dilution that\nfollowed diluted the sample to 397ppm."
                                n414 = local write "Stop Dilution"(FALSE) -> ()
                                n415 = local write "Diluting"(FALSE) -> ()
                                n416 = local write "V21"(FALSE) -> ()
                                n417 = Wait (ms)(milliseconds to wait=1000) -> ()  [unwired: 1 out]
                              }
                              frame #48 {
                                # "Open V20 - pump out bellow + LN2 trap"
                                n418 = local write "V20"(TRUE) -> ()
                                n419 = Wait (ms)(milliseconds to wait=1000) -> ()  [unwired: 1 out]
                              }
                              frame #49 {
                                # "Should already be open anyways"
                                # "Open V18 - pump out bellow + LN2 trap"
                                n420 = local write "V18"(TRUE) -> ()
                                n421 = Wait (ms)(milliseconds to wait=1000) -> ()  [unwired: 1 out]
                              }
                              frame #50 {
                                # "Pump excess N2 out from LN2, bellow for 2min"
                                n422 = call "Time Delay24"() -> ()  [unwired: 11 in, 1 out]
                              }
                              frame #51 {
                                # "Close V20"
                                n423 = local write "V20"(FALSE) -> ()
                                n424 = Wait (ms)(milliseconds to wait=1000) -> ()  [unwired: 1 out]
                              }
                              frame #52 {
                                # "Open V17 - expand flask back into LN2 and bellow volume"
                                n425 = local write "V17"(TRUE) -> ()
                                n426 = Wait (ms)(milliseconds to wait=15000) -> ()  [unwired: 1 out]
                              }
                              frame #53 {
                                n427 = local read "Pressure (mbar)"() -> (w1013:dbl)
                                n428 = call "Convert from Dynamic Data8"("Dynamic Data Type"=w1013) -> ("Array"=w1012:dbl[])  [unwired: 3 in]
                                n429 = call-poly <vilib>:"Mean.vi"("X"=w1012) -> ("mean"=w1014:dbl)  [unwired: 1 out]
                                n430 = local write "Final P (mbar)"(w1014) -> ()
                                n431 = Wait (ms)(milliseconds to wait=200) -> ()  [unwired: 1 out]
                              }
                              frame #54 {
                                n432 = local read "Final Target P (mbar)"() -> (w1017:dbl)
                                n433 = local read "Final P (mbar)"() -> (w1016:dbl)
                                n434 = Divide(x=w1016, y=w1017) -> (x/y=w1018:dbl)
                                n435 = Multiply(x=w1018, y=100.0) -> (x*y=w1019:dbl)
                                n436 = local write "Final P Accuracy (%)"(w1019) -> ()
                                n437 = Wait (ms)(milliseconds to wait=200) -> ()  [unwired: 1 out]
                              }
                              frame #55 {
                                # "Open V16"
                                n438 = local write "V16"(TRUE) -> ()
                                n439 = Wait (ms)(milliseconds to wait=1000) -> ()  [unwired: 1 out]
                              }
                              frame #56 {
                                # "Activate circulation loop"
                                n440 = local write "Circulation Loop"(TRUE) -> ()
                                n441 = call "Prompt User for Input37"() -> ("OK"=w1024:bool)  [unwired: 18 in, 1 out]
                                n442 = Wait (ms)(milliseconds to wait=1000) -> ()  [unwired: 1 out]
                              }
                              frame #57 {
                                # "currently 2,5min"
                                # "Time delay for circulation/mixing"
                                n443 = call "Time Delay25"() -> ()  [unwired: 11 in, 1 out]
                              }
                              frame #58 {
                                n444 = call "Prompt User for Input38"() -> ("OK"=w1027:bool)  [unwired: 18 in, 1 out]
                              }
                              frame #59 {
                                # "Close V16"
                                # "Stop circulation"
                                n445 = local write "Circulation Loop"(FALSE) -> ()
                                n446 = local write "V16"(FALSE) -> ()
                                n447 = Wait (ms)(milliseconds to wait=1000) -> ()  [unwired: 1 out]
                              }
                              frame #60 {
                                n448 = local write "GO!!!!"(FALSE) -> ()
                                n449 = local write "Start Sequence"(FALSE) -> ()
                                n450 = local write "Carbonate Sam"(FALSE) -> ()
                                n451 = local write "Seq. Finished"(TRUE) -> ()
                              }
                            }
                          }
                        }
                      }
                      frame True {
                        n452 = stacked-sequence {
                          tunnel: [_ _ _ _ w1060 _ _ _ _ _ _ _ _ _ _ _ _ _ _ _ _ _ _ _ _ _ _ _ _ _ _ _ _ _ _ _ _ _ _ _ _ _ _ _ _ _ _ _ _ _ _ _ _ _ _ _ _ _ _ _ _] -> _
                          tunnel: [_ _ _ _ _ _ _ _ _ _ _ _ _ _ _ _ w1090 _ _ _ _ _ _ _ _ _ _ _ _ _ _ _ _ _ _ _ _ _ _ _ _ _ _ _ _ _ _ _ _ _ _ _ _ _ _ _ _ _ _ _ _] -> _
                          tunnel: [_ _ _ _ _ w1061 _ _ _ _ _ _ _ _ _ _ _ _ _ _ _ _ _ _ _ _ _ _ _ _ _ _ _ _ _ _ _ _ _ _ _ _ _ _ _ _ _ _ _ _ _ _ _ _ _ _ _ _ _ _ _] -> _
                          tunnel: [_ _ _ _ _ _ _ _ _ _ _ _ _ _ _ _ _ _ _ _ _ _ _ _ _ _ _ _ _ _ _ _ _ _ _ _ _ _ _ _ _ _ _ _ _ _ _ _ _ _ _ _ _ _ _ _ w1325 _ _ _ _] -> _
                          tunnel: [_ _ _ _ _ _ _ _ _ _ _ _ _ _ _ _ _ _ _ _ _ _ _ _ _ _ _ _ _ _ _ _ _ _ _ _ _ _ _ _ _ _ _ _ _ _ _ _ _ _ _ _ _ _ _ _ _ _ w1328 _ _] -> _
                          frame #0 {
                            n453 = local write "Final Target P (mbar)"(0.0) -> ()
                            n454 = local write "Final P Accuracy (%)"(0.0) -> ()
                            n455 = local write "Thaw Yield (torr)"(0.0) -> ()
                            n456 = local write "Final P (mbar)"(0.0) -> ()
                            n457 = local write "Slosh to do"(0.0) -> ()
                            n458 = local write "umol CO2"(0.0) -> ()
                            n459 = local write "No. Slosh"(0.0) -> ()
                            n460 = local write "Dil. i"(0.0) -> ()
                            n461 = local write "Dil. Target P (mbar)"(0.0) -> ()
                            n462 = local write "Dilution P (mbar)"(0.0) -> ()
                            n463 = local write "Rem. slosh frac."(0.0) -> ()
                            n464 = local write "Slosh P (mbar)"(0.0) -> ()
                            n465 = local write "Slosh acc. %"(0.0) -> ()
                            n466 = local write "P frac. slosh"(0.0) -> ()
                            n467 = local write "Exact slosh"(0.0) -> ()
                            n468 = local write "Temp (K)"(294.0) -> ()
                          }
                          frame #1 {
                            # "V18,17,16,20 should all be open to start"
                            # "Open V7"
                            n469 = local write "V7"(TRUE) -> ()
                            n470 = local write "Seq. Finished"(FALSE) -> ()
                            n471 = Wait (ms)(milliseconds to wait=1000) -> ()  [unwired: 1 out]
                          }
                          frame #2 {
                            # "V18,17,16,20 should all be open to start"
                            # "Open V16"
                            n472 = local write "V16"(TRUE) -> ()
                            n473 = Wait (ms)(milliseconds to wait=1000) -> ()  [unwired: 1 out]
                          }
                          frame #3 {
                            # "Close off unselected crackers"
                            n474 = flat-sequence {
                              frame #0 {
                                n475 = local write "V4"(FALSE) -> ()
                              }
                              frame #1 {
                                n476 = Wait (ms)(milliseconds to wait=1000) -> ()  [unwired: 1 out]
                              }
                              frame #2 {
                                n477 = local write "V6"(FALSE) -> ()
                              }
                            }
                            n478 = Wait (ms)(milliseconds to wait=1000) -> ()  [unwired: 1 out]
                          }
                          frame #4 {
                            # "Close flask valves"
                            n479 = call "Prompt User for Input21"() -> ("OK"=w1060:bool)  [unwired: 18 in, 1 out]
                          }
                          frame #5 {
                            # "Close crackers and GB manual valves"
                            n480 = call "Prompt User for Input22"() -> ("OK"=w1061:bool)  [unwired: 18 in, 1 out]
                          }
                          frame #6 {
                            # "Open Loop"
                            n481 = local write "Circulation Loop"(TRUE) -> ()
                            n482 = local write "Prep. Loop"(TRUE) -> ()
                            n483 = Wait (ms)(milliseconds to wait=1000) -> ()  [unwired: 1 out]
                          }
                          frame #7 {
                            # "22/4/22 - background ~280 mtorr bg"
                            # "Pump Loop for 60sec"
                            n484 = call "Time Delay14"() -> ()  [unwired: 11 in, 1 out]
                          }
                          frame #8 {
                            # "Open V8"
                            n485 = local write "V8"(TRUE) -> ()
                            n486 = Wait (ms)(milliseconds to wait=1000) -> ()  [unwired: 1 out]
                          }
                          frame #9 {
                            # "Close V20"
                            n487 = local write "V20"(FALSE) -> ()
                            n488 = Wait (ms)(milliseconds to wait=1000) -> ()  [unwired: 1 out]
                          }
                          frame #10 {
                            # "Open V21"
                            n489 = local write "V21"(TRUE) -> ()
                            n490 = Wait (ms)(milliseconds to wait=1000) -> ()  [unwired: 1 out]
                          }
                          frame #11 {
                            # "When P > 1300 in Loop close V21"
                            n491 = while {
                              shift-right: [w1072] -> _
                              shift-left: _ -> [_]
                              stop <- w1073 stop-if-true
                              n492 = local read "Pressure (mbar)"() -> (w1076:dbl)
                              n493 = Wait (ms)(milliseconds to wait=100) -> ()  [unwired: 1 out]
                              n494 = Greater?(x=w1076, y=1300.0) -> (0:w1075:bool)
                              n495 = case shown="True" w1075 {
                                selector: w1075 -> [w1078 w1081]
                                tunnel: [w1078 w1081] -> w1072
                                frame False {
                                }
                                frame True {
                                n496 = local write "Stop Loop Fill"(TRUE) -> ()
                                n497 = local write "V21"(FALSE) -> ()
                                }
                              }
                              n498 = local read "Stop Loop Fill"() -> (w1073:bool)
                            }
                            n499 = Wait (ms)(milliseconds to wait=1000) -> ()  [unwired: 1 out]
                          }
                          frame #12 {
                            n500 = call "Prompt User for Input23"() -> ()  [unwired: 18 in, 2 out]
                            n501 = local write "Stop Loop Fill"(FALSE) -> ()
                          }
                          frame #13 {
                            # "Shut Loop"
                            n502 = local write "Circulation Loop"(FALSE) -> ()
                            n503 = local write "Prep. Loop"(FALSE) -> ()
                            n504 = Wait (ms)(milliseconds to wait=1000) -> ()  [unwired: 1 out]
                          }
                          frame #14 {
                            # "Close V8"
                            n505 = local write "V8"(FALSE) -> ()
                            n506 = Wait (ms)(milliseconds to wait=1000) -> ()  [unwired: 1 out]
                          }
                          frame #15 {
                            # "Open V20"
                            n507 = local write "V20"(TRUE) -> ()
                            n508 = Wait (ms)(milliseconds to wait=1000) -> ()  [unwired: 1 out]
                          }
                          frame #16 {
                            # "Open crackers manual valve, close GB manual valve"
                            n509 = call "Prompt User for Input24"() -> ("OK"=w1090:bool)  [unwired: 18 in, 1 out]
                          }
                          frame #17 {
                            # "Open V5 - pump out cracker to be used"
                            n510 = local write "V5"(TRUE) -> ()
                            n511 = Wait (ms)(milliseconds to wait=1000) -> ()  [unwired: 1 out]
                          }
                          frame #18 {
                            # "When P < 0,076 torr continue w/ sequence"
                            n512 = while {
                              shift-right: [w1094] -> _
                              shift-left: _ -> [_]
                              stop <- w1095 stop-if-true
                              n513 = local read "Agilent (Torr)"() -> (w1098:dbl)
                              n514 = Wait (ms)(milliseconds to wait=100) -> ()  [unwired: 1 out]
                              n515 = Less?(x=w1098, y=0.076) -> (x < y?=w1097:bool)
                              n516 = case shown="True" w1097 {
                                selector: w1097 -> [w1100 w1102]
                                tunnel: [w1100 w1102] -> w1094
                                frame False {
                                }
                                frame True {
                                n517 = local write "Stop Pump Over"(TRUE) -> ()
                                }
                              }
                              n518 = local read "Stop Pump Over"() -> (w1095:bool)
                            }
                            n519 = Wait (ms)(milliseconds to wait=1000) -> ()  [unwired: 1 out]
                          }
                          frame #19 {
                            # "10 extra sec to pump out bottom cracker volume"
                            n520 = local write "Stop Pump Over"(FALSE) -> ()
                            n521 = Wait (ms)(milliseconds to wait=10000) -> ()  [unwired: 1 out]
                          }
                          frame #20 {
                            # "Redundant just in case"
                            # "Close V4"
                            n522 = local write "V4"(FALSE) -> ()
                            n523 = Wait (ms)(milliseconds to wait=1000) -> ()  [unwired: 1 out]
                          }
                          frame #21 {
                            # "Redundant just in case"
                            # "Close V6"
                            n524 = local write "V6"(FALSE) -> ()
                            n525 = Wait (ms)(milliseconds to wait=1000) -> ()  [unwired: 1 out]
                          }
                          frame #22 {
                            # "Dewar up"
                            n526 = local write "D"(TRUE) -> ()
                            n527 = Wait (ms)(milliseconds to wait=1000) -> ()  [unwired: 1 out]
                          }
                          frame #23 {
                            # "15 sec for trap to cool"
                            n528 = Wait (ms)(milliseconds to wait=15000) -> ()  [unwired: 1 out]
                          }
                          frame #24 {
                            # "Close V18"
                            n529 = local write "V18"(FALSE) -> ()
                            n530 = Wait (ms)(milliseconds to wait=1000) -> ()  [unwired: 1 out]
                          }
                          frame #25 {
                            # "Break tube light on"
                            n531 = local write "Break Tube"(TRUE) -> ()
                            n532 = Wait (ms)(milliseconds to wait=1000) -> ()  [unwired: 1 out]
                          }
                          frame #26 {
                            # "10 min cryo-pull"
                            n533 = local write "Cryo-pull"(TRUE) -> ()
                            n534 = call "Cryo pull t6"() -> ()  [unwired: 11 in, 1 out]
                          }
                          frame #27 {
                            # "Open V18 - pump over"
                            n535 = local write "V18"(TRUE) -> ()
                            n536 = Wait (ms)(milliseconds to wait=5000) -> ()  [unwired: 1 out]
                          }
                          frame #28 {
                            # "When P < 0.075 torr close LN2 trap"
                            n537 = while {
                              shift-right: [w1121] -> _
                              shift-left: _ -> [_]
                              stop <- w1123 stop-if-true
                              n538 = local read "Agilent (Torr)"() -> (w1126:dbl)
                              n539 = Wait (ms)(milliseconds to wait=100) -> ()  [unwired: 1 out]
                              n540 = Less?(x=w1126, y=0.075) -> (x < y?=w1124:bool)
                              n541 = case shown="True" w1124 {
                                selector: w1124 -> [w1127 w1128]
                                tunnel: [w1127 w1128] -> w1121
                                frame False {
                                }
                                frame True {
                                w1130 = FALSE
                                n542 = local write "V17"(w1130) -> ()
                                n543 = local write "V18"(w1130) -> ()
                                n544 = local write "Stop Pump Over"(TRUE) -> ()
                                }
                              }
                              n545 = local read "Stop Pump Over"() -> (w1123:bool)
                            }
                            n546 = local write "Cryo-pull"(FALSE) -> ()
                            n547 = Wait (ms)(milliseconds to wait=1000) -> ()  [unwired: 1 out]
                          }
                          frame #29 {
                            # "Close V16"
                            n548 = local write "Stop Pump Over"(FALSE) -> ()
                            n549 = local write "V16"(FALSE) -> ()
                            n550 = Wait (ms)(milliseconds to wait=1000) -> ()  [unwired: 1 out]
                          }
                          frame #30 {
                            # "Close V5"
                            n551 = local write "V5"(FALSE) -> ()
                            n552 = Wait (ms)(milliseconds to wait=1000) -> ()  [unwired: 1 out]
                          }
                          frame #31 {
                            # "Dewar down"
                            n553 = local write "D"(FALSE) -> ()
                            n554 = Wait (ms)(milliseconds to wait=1000) -> ()  [unwired: 1 out]
                          }
                          frame #32 {
                            # "6 minute thaw"
                            n555 = call "Time Delay15"() -> ()  [unwired: 11 in, 1 out]
                            n556 = local write "Thawing"(TRUE) -> ()
                            n557 = call "Display Message to User9"() -> ()  [unwired: 10 in, 2 out]
                          }
                          frame #33 {
                            n558 = call "Display Message to User10"() -> ()  [unwired: 10 in, 2 out]
                          }
                          frame #34 {
                            # "Read thaw P on Agilent - calculate umol CO2 trapped"
                            n559 = local write "Thawing"(FALSE) -> ()
                            n560 = flat-sequence {
                              frame #0 {
                                n561 = local read "Agilent (Torr)"() -> (w1142:dbl)
                                n562 = local write "Thaw Yield (torr)"(w1142) -> ()
                                n563 = Wait (ms)(milliseconds to wait=200) -> ()  [unwired: 1 out]
                              }
                              frame #1 {
                                # "mol CO2"
                                # "''Cast base units''"
                                # "R"
                                # "V LN2, in m3"
                                # "torr to Pa"
                                n564 = local read "Thaw Yield (torr)"() -> (w1150:dbl)
                                n565 = local read "Temp (K)"() -> (w1143:dbl)
                                n566 = Cast Unit Bases(0:dbl[unit] 8.3144598) -> (2:w1144:dbl)  [unwired: 1 in]
                                n567 = Multiply(x=w1150, y=133.3223684211) -> (x*y=w1149:dbl)
                                n568 = Multiply(x=w1144, y=w1143) -> (x*y=w1148:dbl)
                                n569 = Multiply(x=w1149, y=6.1e-05) -> (x*y=w1154:dbl)
                                n570 = Divide(x=w1154, y=w1148) -> (x/y=w1147:dbl)
                                n571 = Multiply(x=1000000.0, y=w1147) -> (x*y=w1145:dbl)
                                n572 = local write "umol CO2"(w1145) -> ()
                              }
                            }
                            n573 = Wait (ms)(milliseconds to wait=500) -> ()  [unwired: 1 out]
                          }
                          frame #35 {
                            # "P for 400ppm"
                            # "22/4/22\nOffset \nfor extra\nN2 from \nloop"
                            # "Calculate and store Target P"
                            # "''Cast base units''"
                            # "R"
                            # "''Cast base units''"
                            # "R"
                            # "PV=nrt\nP - Pa\nV - m3\nn - mol\nR - \nT - K"
                            # "Pa to mbar"
                            # "P = nRT/V"
                            # "Pa"
                            # "mol N2 to dilute"
                            # "V LN2, flask, bellow in m3"
                            # "ppm"
                            # "n mol N2 = x mol CO2/0.000400"
                            # "0.000400 = x mol CO2/n mol N2"
                            # "mol CO2"
                            # "V LN2, in m3"
                            # "torr to Pa"
                            n574 = local read "Thaw Yield (torr)"() -> (w1174:dbl)
                            n575 = local read "Temp (K)"() -> (w1158:dbl)
                            n576 = Subtract(x=w1174, y=0.2) -> (x-y=w1173:dbl)
                            n577 = Cast Unit Bases(0:dbl[unit] 8.3144598) -> (2:w1165:dbl)  [unwired: 1 in]
                            n578 = Multiply(x=w1173, y=133.3223684211) -> (x*y=w1156:dbl)
                            n579 = Multiply(x=w1165, y=w1158) -> (x*y=w1157:dbl)
                            n580 = Multiply(x=w1156, y=6.1e-05) -> (x*y=w1155:dbl)
                            n581 = Divide(x=w1155, y=w1157) -> (x/y=w1162:dbl)
                            n582 = Divide(x=w1162, y=0.0004) -> (x/y=w1176:dbl)
                            n583 = Cast Unit Bases(0:dbl[unit] 8.3144598) -> (2:w1164:dbl)  [unwired: 1 in]
                            n584 = local read "Temp (K)"() -> (w1161:dbl)
                            n585 = Multiply(x=w1164, y=w1176) -> (x*y=w1160:dbl)
                            n586 = Multiply(x=w1161, y=w1160) -> (x*y=w1159:dbl)
                            n587 = Divide(x=w1159, y=0.000687) -> (x/y=w1163:dbl)
                            n588 = Multiply(x=0.01, y=w1163) -> (x*y=w1177:dbl)
                            n589 = local write "Final Target P (mbar)"(w1177) -> ()
                            n590 = Wait (ms)(milliseconds to wait=200) -> ()  [unwired: 1 out]
                          }
                          frame #36 {
                            # "Calculate Dilution Target Pressure in prep for final expansion"
                            # "Dil. TP fills full MV, V17 closes\n101ml pumped away (all but flask)\n586ml @ Dil. TP expands to 687ml\n--> 687ml @ Final P (P for 400ppm)"
                            # "P1V1 = P2V2\nDTP*586ml = TFP*687ml\nDTP = (FP*687)/586"
                            n591 = local read "Final Target P (mbar)"() -> (w1180:dbl)
                            n592 = Multiply(x=w1180, y=687.0) -> (x*y=w1181:dbl)
                            n593 = Divide(x=w1181, y=586.0) -> (x/y=w1183:dbl)
                            n594 = local write "Dil. Target P (mbar)"(w1183) -> ()
                            n595 = Wait (ms)(milliseconds to wait=200) -> ()  [unwired: 1 out]
                          }
                          frame #37 {
                            # "22/2/22\nAvg of n=2 1500 mbar auto test sloshes:\nn = 3E-6x^2 + 0,003x + 0,0254"
                            # "21/2/22\n1400 mbar auto test sloshes:\nn = 3E-6x^2 + 0,0033x + 0,0268\nn        x (P mbar)\n0        0\n1        232\n2        430\n3        569\n4        733\n5        847"
                            # "8/2/22\n1100 mbar manual sloshes:\nn = 1E-5x^2 + 0,0003x + 0,3052\nn        x (P mbar)\n0        0\n1        205\n2        345\n3        477\n4        587\n5        678\n6        755\n7        819\n8        872\n9        916\n10      951\n11      981"
                            n596 = flat-sequence {
                              frame #0 {
                                # "Currently using avg curve for (Avg(Avg(1500x2),1400))\nn = 3E-6x^2 + 0.0031x + 0.0261"
                                # "Given Dilution Target Pressure, calculate how many sloshes it would take to get \nthe pressure in the full MV to that pressure."
                                n597 = local read "Dil. Target P (mbar)"() -> (w1196:dbl)
                                n598 = local read "Dil. Target P (mbar)"() -> (w1194:dbl)
                                n599 = Square(x=w1196) -> (x^2=w1195:dbl)
                                n600 = Multiply(x=3e-06, y=w1195) -> (x*y=w1192:dbl)
                                n601 = Multiply(x=w1194, y=0.0031) -> (x*y=w1193:dbl)
                                n602 = Add(x=w1192, y=w1193) -> (x+y=w1191:dbl)
                                n603 = Add(x=w1191, y=0.0261) -> (x+y=w1187:dbl)
                                n604 = local write "Exact slosh"(w1187) -> ()
                                n605 = Wait (ms)(milliseconds to wait=100) -> ()  [unwired: 1 out]
                              }
                              frame #1 {
                                # "Now take that calculated number of \nsloshes and round down to nearest integer."
                                n606 = local read "Exact slosh"() -> (w1198:dbl)
                                n607 = Round Toward -Infinity(1:w1198) -> (0:w1199:dbl)
                                n608 = local write "Slosh to do"(w1199) -> ()
                                n609 = Wait (ms)(milliseconds to wait=100) -> ()  [unwired: 1 out]
                              }
                              frame #2 {
                                n610 = local read "Exact slosh"() -> (w1202:dbl)
                                n611 = local read "Slosh to do"() -> (w1201:dbl)
                                n612 = Subtract(x=w1202, y=w1201) -> (x-y=w1203:dbl)
                                n613 = local write "Rem. slosh frac."(w1203) -> ()
                                n614 = Wait (ms)(milliseconds to wait=100) -> ()  [unwired: 1 out]
                              }
                              frame #3 {
                                n615 = local read "Rem. slosh frac."() -> (w1207:dbl)
                                n616 = Multiply(x=1450.0, y=w1207) -> (x*y=w1206:dbl)
                                n617 = local write "P frac. slosh"(w1206) -> ()
                                n618 = Wait (ms)(milliseconds to wait=100) -> ()  [unwired: 1 out]
                              }
                            }
                            n619 = Wait (ms)(milliseconds to wait=200) -> ()  [unwired: 1 out]
                          }
                          frame #38 {
                            # "P should be something like 250mtor (V LN2 ~1/10 of V LN2 + flask)"
                            # "Open, Close V17 - pure CO2 expansion into flask\nEqual concentration of CO2 in LN2, flask, and H of V16/V17"
                            n620 = flat-sequence {
                              frame #0 {
                                n621 = local write "V17"(TRUE) -> ()
                              }
                              frame #1 {
                                n622 = Wait (ms)(milliseconds to wait=u32 40000) -> ()  [unwired: 1 out]
                              }
                              frame #2 {
                                n623 = local write "V17"(FALSE) -> ()
                              }
                            }
                            n624 = Wait (ms)(milliseconds to wait=1000) -> ()  [unwired: 1 out]
                          }
                          frame #39 {
                            # "Close V20"
                            n625 = local write "V20"(FALSE) -> ()
                            n626 = Wait (ms)(milliseconds to wait=1000) -> ()  [unwired: 1 out]
                          }
                          frame #40 {
                            # "Open V8 - begin dilution steps"
                            n627 = local write "Diluting"(TRUE) -> ()
                            n628 = local write "V8"(TRUE) -> ()
                            n629 = Wait (ms)(milliseconds to wait=1000) -> ()  [unwired: 1 out]
                          }
                          frame #41 {
                            # "Open V21"
                            n630 = local write "V21"(TRUE) -> ()
                            n631 = Wait (ms)(milliseconds to wait=1000) -> ()  [unwired: 1 out]
                          }
                          frame #42 {
                            # "Build P in bellow before introducing to LN2 trap w/ sample"
                            n632 = call "Pressurize in LN15"() -> ()  [unwired: 11 in, 1 out]
                          }
                          frame #43 {
                            # "Open V18"
                            n633 = local write "V18"(TRUE) -> ()
                            n634 = Wait (ms)(milliseconds to wait=1000) -> ()  [unwired: 1 out]
                          }
                          frame #44 {
                            n635 = local read "Slosh to do"() -> (w1221:dbl)
                            n636 = for {
                              N: w1221 -> [_]
                              n637 = flat-sequence {
                                frame #0 {
                                n638 = while {
                                shift-right: [w1223] -> _
                                shift-left: _ -> [_]
                                stop <- w1224 stop-if-true
                                # "Greater difference in P causes more \nturbulent mixing when expanded into flask"
                                # "When P in bellow + LN2 is > 1450mbar, Open V17"
                                n639 = local read "Pressure (mbar)"() -> (w1226:dbl)
                                n640 = Wait (ms)(milliseconds to wait=100) -> ()  [unwired: 1 out]
                                n641 = Greater?(x=w1226, y=1450.0) -> (0:w1227:bool)
                                n642 = case shown="True" w1227 {
                                selector: w1227 -> [w1228 w1230]
                                tunnel: [w1228 w1230] -> w1223
                                frame False {
                                }
                                frame True {
                                n643 = local write "Stop Sample Pressure"(TRUE) -> ()
                                n644 = local write "V17"(TRUE) -> ()
                                }
                                }
                                n645 = local read "Stop Sample Pressure"() -> (w1224:bool)
                                }
                                }
                                frame #1 {
                                n646 = local read "No. Slosh"() -> (w1232:dbl)
                                n647 = local write "Stop Sample Pressure"(FALSE) -> ()
                                n648 = Increment(x=w1232) -> (x+1=w1233:dbl)
                                n649 = Wait (ms)(milliseconds to wait=4000) -> ()  [unwired: 1 out]
                                n650 = local write "No. Slosh"(w1233) -> ()
                                }
                                frame #2 {
                                n651 = local read "Pressure (mbar)"() -> (w1236:dbl)
                                n652 = local write "Slosh P (mbar)"(w1236) -> ()
                                n653 = Wait (ms)(milliseconds to wait=1000) -> ()  [unwired: 1 out]
                                }
                                frame #3 {
                                n654 = local write "V17"(FALSE) -> ()
                                n655 = Wait (ms)(milliseconds to wait=1000) -> ()  [unwired: 1 out]
                                }
                              }
                            }
                          }
                          frame #45 {
                            # "Check that the final fractional slosh P \nwill be greater P than what's in the \nflask already. If yes, do fractional slosh; \nif no, skip it and go straight to diluting to DTP."
                            n656 = local read "Slosh P (mbar)"() -> (w1242:dbl)
                            n657 = local read "P frac. slosh"() -> (w1241:dbl)
                            n658 = Greater Or Equal?(x=w1241, y=w1242) -> (x >= y?=w1240:bool)
                            n659 = case shown="True" w1240 {
                              frame False {
                                # "Open V17"
                                n660 = local write "V17"(TRUE) -> ()
                                n661 = local read "Dil. Target P (mbar)"() -> (w1244:dbl)
                                n662 = local read "Slosh P (mbar)"() -> (w1243:dbl)
                                n663 = Divide(x=w1243, y=w1244) -> (x/y=w1247:dbl)
                                n664 = Multiply(x=w1247, y=100.0) -> (x*y=w1245:dbl)
                                n665 = local write "Slosh acc. %"(w1245) -> ()
                                n666 = Wait (ms)(milliseconds to wait=1000) -> ()  [unwired: 1 out]
                              }
                              frame True {
                                # "Last slosh into flask, keep V17 open so dilution loop can start right after"
                                n667 = flat-sequence {
                                frame #0 {
                                n668 = local read "Rem. slosh frac."() -> (w1252:dbl)
                                n669 = local read "No. Slosh"() -> (w1253:dbl)
                                n670 = Wait (ms)(milliseconds to wait=100) -> ()  [unwired: 1 out]
                                n671 = Add(x=w1253, y=w1252) -> (x+y=w1251:dbl)
                                n672 = local write "Slosh to do"(w1251) -> ()
                                }
                                frame #1 {
                                n673 = while {
                                shift-right: [w1256] -> _
                                shift-left: _ -> [_]
                                stop <- w1258 stop-if-true
                                # "When P in bellow + LN2 is > fractional slosh P, Open V17"
                                n674 = local read "Pressure (mbar)"() -> (w1259:dbl)
                                n675 = local read "P frac. slosh"() -> (w1254:dbl)
                                n676 = Wait (ms)(milliseconds to wait=100) -> ()  [unwired: 1 out]
                                n677 = Greater Or Equal?(x=w1259, y=w1254) -> (x >= y?=w1257:bool)
                                n678 = case shown="True" w1257 {
                                selector: w1257 -> [w1260 w1261]
                                tunnel: [w1260 w1261] -> w1256
                                frame False {
                                }
                                frame True {
                                n679 = local write "Stop Sample Pressure"(TRUE) -> ()
                                n680 = local write "V17"(TRUE) -> ()
                                }
                                }
                                n681 = local read "Stop Sample Pressure"() -> (w1258:bool)
                                }
                                }
                                frame #2 {
                                n682 = local read "Rem. slosh frac."() -> (w1264:dbl)
                                n683 = local read "No. Slosh"() -> (w1265:dbl)
                                n684 = local write "Stop Sample Pressure"(FALSE) -> ()
                                n685 = Add(x=w1265, y=w1264) -> (x+y=w1266:dbl)
                                n686 = Wait (ms)(milliseconds to wait=5000) -> ()  [unwired: 1 out]
                                n687 = local write "No. Slosh"(w1266) -> ()
                                }
                                frame #3 {
                                n688 = local read "Pressure (mbar)"() -> (w1269:dbl)
                                n689 = local write "Slosh P (mbar)"(w1269) -> ()
                                n690 = Wait (ms)(milliseconds to wait=500) -> ()  [unwired: 1 out]
                                }
                                frame #4 {
                                n691 = local read "Slosh P (mbar)"() -> (w1272:dbl)
                                n692 = local read "Dil. Target P (mbar)"() -> (w1273:dbl)
                                n693 = Divide(x=w1272, y=w1273) -> (x/y=w1276:dbl)
                                n694 = Multiply(x=w1276, y=100.0) -> (x*y=w1274:dbl)
                                n695 = local write "Slosh acc. %"(w1274) -> ()
                                n696 = Wait (ms)(milliseconds to wait=200) -> ()  [unwired: 1 out]
                                }
                                }
                              }
                            }
                          }
                          frame #46 {
                            # "Dil. TP fills full MV, V17 closes\n101ml pumped away (all but flask)\n586ml @ Dil. TP expands to 687ml\n--> 687ml @ Final P (P for 400ppm)"
                            # "Agilent P comes through the DAQ"
                            # "When P Wika = maths for 400ppm dilution, close V8"
                            n697 = local read "Dil. Target P (mbar)"() -> (w1279:dbl)
                            n698 = local read "Pressure (mbar)"() -> (w1278:dbl)
                            n699 = Greater?(x=w1279, y=w1278) -> (0:w1277:bool)
                            n700 = case shown="True" w1277 {
                              frame False {
                                n701 = local write "V17"(FALSE) -> ()
                                n702 = local write "V8"(FALSE) -> ()
                                n703 = call "Display Message to User11"() -> ()  [unwired: 10 in, 2 out]
                              }
                              frame True {
                                n704 = while {
                                shift-right: [w1284] -> _
                                shift-left: _ -> [_]
                                i -> [w1294]
                                stop <- w1295 stop-if-true
                                n705 = local read "Dil. Target P (mbar)"() -> (w1292:dbl)
                                n706 = local write "Dil. i"(w1294) -> ()
                                n707 = local read "Pressure (mbar)"() -> (w1291:dbl)
                                n708 = local read "Pressure (mbar)"() -> (w1289:dbl)
                                n709 = Add(x=w1289, y=2.0) -> (x+y=w1288:dbl)
                                n710 = Subtract(x=w1291, y=2.0) -> (x-y=w1287:dbl)
                                n711 = Wait (ms)(milliseconds to wait=u32 100) -> ()  [unwired: 1 out]
                                n712 = In Range and Coerce(upper limit=w1288, x=w1292, lower limit=w1287) -> (coerced(x)=w1283:dbl, In Range?=w1290:bool)
                                n713 = local write "Dilution P (mbar)"(w1283) -> ()
                                n714 = case shown="True" w1290 {
                                selector: w1290 -> [w1296 w1300]
                                tunnel: [w1296 w1300] -> w1284
                                frame False {
                                }
                                frame True {
                                n715 = local write "V8"(FALSE) -> ()
                                n716 = local write "Stop Dilution"(TRUE) -> ()
                                n717 = local write "V17"(FALSE) -> ()
                                }
                                }
                                n718 = local read "Stop Dilution"() -> (w1295:bool)
                                }
                              }
                            }
                            n719 = Wait (ms)(milliseconds to wait=1000) -> ()  [unwired: 1 out]
                          }
                          frame #47 {
                            # "Close V21 - N2 inlet - want to keep this volume under superambient pressure always"
                            # "Flask will be over concentrated in CO2 (hopefully somewhere around 480ppm - cant really check that so it's blind)\n19/1/22, 8:00 - Initial manual test of this measured 472ppm on the Licor. Sample expansion and re-dilution that\nfollowed diluted the sample to 397ppm."
                            n720 = local write "Stop Dilution"(FALSE) -> ()
                            n721 = local write "Diluting"(FALSE) -> ()
                            n722 = local write "V21"(FALSE) -> ()
                            n723 = Wait (ms)(milliseconds to wait=1000) -> ()  [unwired: 1 out]
                          }
                          frame #48 {
                            # "Open V20 - pump out bellow + LN2 trap"
                            n724 = local write "V20"(TRUE) -> ()
                            n725 = Wait (ms)(milliseconds to wait=1000) -> ()  [unwired: 1 out]
                          }
                          frame #49 {
                            # "Should already be open anyways"
                            # "Open V18 - pump out bellow + LN2 trap"
                            n726 = local write "V18"(TRUE) -> ()
                            n727 = Wait (ms)(milliseconds to wait=1000) -> ()  [unwired: 1 out]
                          }
                          frame #50 {
                            # "Pump excess N2 out from LN2, bellow for 2min"
                            n728 = call "Time Delay16"() -> ()  [unwired: 11 in, 1 out]
                          }
                          frame #51 {
                            # "Close V20"
                            n729 = local write "V20"(FALSE) -> ()
                            n730 = Wait (ms)(milliseconds to wait=1000) -> ()  [unwired: 1 out]
                          }
                          frame #52 {
                            # "Open V17 - expand flask back into LN2 and bellow volume"
                            n731 = local write "V17"(TRUE) -> ()
                            n732 = Wait (ms)(milliseconds to wait=15000) -> ()  [unwired: 1 out]
                          }
                          frame #53 {
                            n733 = local read "Pressure (mbar)"() -> (w1314:dbl)
                            n734 = call "Convert from Dynamic Data6"("Dynamic Data Type"=w1314) -> ("Array"=w1313:dbl[])  [unwired: 3 in]
                            n735 = call-poly <vilib>:"Mean.vi"("X"=w1313) -> ("mean"=w1315:dbl)  [unwired: 1 out]
                            n736 = local write "Final P (mbar)"(w1315) -> ()
                            n737 = Wait (ms)(milliseconds to wait=200) -> ()  [unwired: 1 out]
                          }
                          frame #54 {
                            n738 = local read "Final Target P (mbar)"() -> (w1318:dbl)
                            n739 = local read "Final P (mbar)"() -> (w1317:dbl)
                            n740 = Divide(x=w1317, y=w1318) -> (x/y=w1319:dbl)
                            n741 = Multiply(x=w1319, y=100.0) -> (x*y=w1320:dbl)
                            n742 = local write "Final P Accuracy (%)"(w1320) -> ()
                            n743 = Wait (ms)(milliseconds to wait=200) -> ()  [unwired: 1 out]
                          }
                          frame #55 {
                            # "Open V16"
                            n744 = local write "V16"(TRUE) -> ()
                            n745 = Wait (ms)(milliseconds to wait=1000) -> ()  [unwired: 1 out]
                          }
                          frame #56 {
                            # "Activate circulation loop"
                            n746 = local write "Circulation Loop"(TRUE) -> ()
                            n747 = call "Prompt User for Input25"() -> ("OK"=w1325:bool)  [unwired: 18 in, 1 out]
                            n748 = Wait (ms)(milliseconds to wait=1000) -> ()  [unwired: 1 out]
                          }
                          frame #57 {
                            # "currently 2,5min"
                            # "Time delay for circulation/mixing"
                            n749 = call "Time Delay17"() -> ()  [unwired: 11 in, 1 out]
                          }
                          frame #58 {
                            n750 = call "Prompt User for Input26"() -> ("OK"=w1328:bool)  [unwired: 18 in, 1 out]
                          }
                          frame #59 {
                            # "Close V16"
                            # "Stop circulation"
                            n751 = local write "Circulation Loop"(FALSE) -> ()
                            n752 = local write "V16"(FALSE) -> ()
                            n753 = Wait (ms)(milliseconds to wait=1000) -> ()  [unwired: 1 out]
                          }
                          frame #60 {
                            n754 = local write "GO!!!!"(FALSE) -> ()
                            n755 = local write "Start Sequence"(FALSE) -> ()
                            n756 = local write "Carbonate Sam"(FALSE) -> ()
                            n757 = local write "Seq. Finished"(TRUE) -> ()
                          }
                        }
                      }
                    }
                  }
                  frame True {
                    n758 = stacked-sequence {
                      frame #0 {
                        n759 = local write "Final Target P (mbar)"(0.0) -> ()
                        n760 = local write "Final P Accuracy (%)"(0.0) -> ()
                        n761 = local write "Thaw Yield (torr)"(0.0) -> ()
                        n762 = local write "Final P (mbar)"(0.0) -> ()
                        n763 = local write "Slosh to do"(0.0) -> ()
                        n764 = local write "umol CO2"(0.0) -> ()
                        n765 = local write "No. Slosh"(0.0) -> ()
                        n766 = local write "Dil. i"(0.0) -> ()
                        n767 = local write "Dil. Target P (mbar)"(0.0) -> ()
                        n768 = local write "Dilution P (mbar)"(0.0) -> ()
                        n769 = local write "Rem. slosh frac."(0.0) -> ()
                        n770 = local write "Slosh P (mbar)"(0.0) -> ()
                        n771 = local write "Slosh acc. %"(0.0) -> ()
                        n772 = local write "P frac. slosh"(0.0) -> ()
                        n773 = local write "Exact slosh"(0.0) -> ()
                        n774 = local write "Temp (K)"(294.0) -> ()
                      }
                      frame #1 {
                        # "V18,17,16,20 should all be open to start"
                        # "Open V7"
                        n775 = local write "V7"(TRUE) -> ()
                        n776 = local write "Seq. Finished"(FALSE) -> ()
                        n777 = Wait (ms)(milliseconds to wait=1000) -> ()  [unwired: 1 out]
                      }
                      frame #2 {
                        # "V18,17,16,20 should all be open to start"
                        # "Open V16"
                        n778 = local write "V16"(TRUE) -> ()
                        n779 = Wait (ms)(milliseconds to wait=1000) -> ()  [unwired: 1 out]
                      }
                      frame #3 {
                        # "Close off unselected crackers"
                        n780 = flat-sequence {
                          frame #0 {
                            n781 = local write "V5"(FALSE) -> ()
                          }
                          frame #1 {
                            n782 = Wait (ms)(milliseconds to wait=1000) -> ()  [unwired: 1 out]
                          }
                          frame #2 {
                            n783 = local write "V6"(FALSE) -> ()
                          }
                        }
                        n784 = Wait (ms)(milliseconds to wait=1000) -> ()  [unwired: 1 out]
                      }
                      frame #4 {
                        # "Close flask valves"
                        n785 = call "Prompt User for Input15"() -> ()  [unwired: 18 in, 2 out]
                      }
                      frame #5 {
                        # "Close crackers and GB manual valves"
                        n786 = call "Prompt User for Input18"() -> ()  [unwired: 18 in, 2 out]
                      }
                      frame #6 {
                        # "Open Loop"
                        n787 = local write "Circulation Loop"(TRUE) -> ()
                        n788 = local write "Prep. Loop"(TRUE) -> ()
                        n789 = Wait (ms)(milliseconds to wait=1000) -> ()  [unwired: 1 out]
                      }
                      frame #7 {
                        # "22/4/22 - background ~280 mtorr bg"
                        # "Pump Loop for 60sec"
                        n790 = call "Time Delay10"() -> ()  [unwired: 11 in, 1 out]
                      }
                      frame #8 {
                        # "Open V8"
                        n791 = local write "V8"(TRUE) -> ()
                        n792 = Wait (ms)(milliseconds to wait=1000) -> ()  [unwired: 1 out]
                      }
                      frame #9 {
                        # "Close V20"
                        n793 = local write "V20"(FALSE) -> ()
                        n794 = Wait (ms)(milliseconds to wait=1000) -> ()  [unwired: 1 out]
                      }
                      frame #10 {
                        # "Open V21"
                        n795 = local write "V21"(TRUE) -> ()
                        n796 = Wait (ms)(milliseconds to wait=1000) -> ()  [unwired: 1 out]
                      }
                      frame #11 {
                        # "When P > 1300 in Loop close V21"
                        n797 = while {
                          shift-right: [w1371] -> _
                          shift-left: _ -> [_]
                          stop <- w1372 stop-if-true
                          n798 = local read "Pressure (mbar)"() -> (w1375:dbl)
                          n799 = Wait (ms)(milliseconds to wait=100) -> ()  [unwired: 1 out]
                          n800 = Greater?(x=w1375, y=1300.0) -> (0:w1374:bool)
                          n801 = case shown="True" w1374 {
                            selector: w1374 -> [w1377 w1380]
                            tunnel: [w1377 w1380] -> w1371
                            frame False {
                            }
                            frame True {
                              n802 = local write "Stop Loop Fill"(TRUE) -> ()
                              n803 = local write "V21"(FALSE) -> ()
                            }
                          }
                          n804 = local read "Stop Loop Fill"() -> (w1372:bool)
                        }
                        n805 = Wait (ms)(milliseconds to wait=1000) -> ()  [unwired: 1 out]
                      }
                      frame #12 {
                        n806 = call "Prompt User for Input16"() -> ()  [unwired: 18 in, 2 out]
                        n807 = local write "Stop Loop Fill"(FALSE) -> ()
                      }
                      frame #13 {
                        # "Shut Loop"
                        n808 = local write "Circulation Loop"(FALSE) -> ()
                        n809 = local write "Prep. Loop"(FALSE) -> ()
                        n810 = Wait (ms)(milliseconds to wait=1000) -> ()  [unwired: 1 out]
                      }
                      frame #14 {
                        # "Close V8"
                        n811 = local write "V8"(FALSE) -> ()
                        n812 = Wait (ms)(milliseconds to wait=1000) -> ()  [unwired: 1 out]
                      }
                      frame #15 {
                        # "Open V20"
                        n813 = local write "V20"(TRUE) -> ()
                        n814 = Wait (ms)(milliseconds to wait=1000) -> ()  [unwired: 1 out]
                      }
                      frame #16 {
                        # "Open crackers manual valve, close GB manual valve"
                        n815 = call "Prompt User for Input17"() -> ()  [unwired: 18 in, 2 out]
                      }
                      frame #17 {
                        # "Open V4 - pump out cracker to be used"
                        n816 = local write "V4"(TRUE) -> ()
                        n817 = Wait (ms)(milliseconds to wait=1000) -> ()  [unwired: 1 out]
                      }
                      frame #18 {
                        # "When P < 0,076 torr continue w/ sequence"
                        n818 = while {
                          shift-right: [w1392] -> _
                          shift-left: _ -> [_]
                          stop <- w1393 stop-if-true
                          n819 = local read "Agilent (Torr)"() -> (w1396:dbl)
                          n820 = Wait (ms)(milliseconds to wait=100) -> ()  [unwired: 1 out]
                          n821 = Less?(x=w1396, y=0.076) -> (x < y?=w1395:bool)
                          n822 = case shown="True" w1395 {
                            selector: w1395 -> [w1398 w1400]
                            tunnel: [w1398 w1400] -> w1392
                            frame False {
                            }
                            frame True {
                              n823 = local write "Stop Pump Over"(TRUE) -> ()
                            }
                          }
                          n824 = local read "Stop Pump Over"() -> (w1393:bool)
                        }
                        n825 = Wait (ms)(milliseconds to wait=1000) -> ()  [unwired: 1 out]
                      }
                      frame #19 {
                        # "10 extra sec to pump out bottom cracker volume"
                        n826 = local write "Stop Pump Over"(FALSE) -> ()
                        n827 = Wait (ms)(milliseconds to wait=10000) -> ()  [unwired: 1 out]
                      }
                      frame #20 {
                        # "Redundant just in case"
                        # "Close V5"
                        n828 = local write "V5"(FALSE) -> ()
                        n829 = Wait (ms)(milliseconds to wait=1000) -> ()  [unwired: 1 out]
                      }
                      frame #21 {
                        # "Redundant just in case"
                        # "Close V6"
                        n830 = local write "V6"(FALSE) -> ()
                        n831 = Wait (ms)(milliseconds to wait=1000) -> ()  [unwired: 1 out]
                      }
                      frame #22 {
                        # "Dewar up"
                        n832 = local write "D"(TRUE) -> ()
                        n833 = Wait (ms)(milliseconds to wait=1000) -> ()  [unwired: 1 out]
                      }
                      frame #23 {
                        # "15 sec for trap to cool"
                        n834 = Wait (ms)(milliseconds to wait=15000) -> ()  [unwired: 1 out]
                      }
                      frame #24 {
                        # "Close V18"
                        n835 = local write "V18"(FALSE) -> ()
                        n836 = Wait (ms)(milliseconds to wait=1000) -> ()  [unwired: 1 out]
                      }
                      frame #25 {
                        # "Break tube light on"
                        n837 = local write "Break Tube"(TRUE) -> ()
                        n838 = Wait (ms)(milliseconds to wait=1000) -> ()  [unwired: 1 out]
                      }
                      frame #26 {
                        # "10 min cryo-pull"
                        n839 = local write "Cryo-pull"(TRUE) -> ()
                        n840 = call "Cryo pull t"() -> ()  [unwired: 11 in, 1 out]
                      }
                      frame #27 {
                        # "Open V18 - pump over"
                        n841 = local write "V18"(TRUE) -> ()
                        n842 = Wait (ms)(milliseconds to wait=5000) -> ()  [unwired: 1 out]
                      }
                      frame #28 {
                        # "When P < 0.075 torr close LN2 trap"
                        n843 = while {
                          shift-right: [w1419] -> _
                          shift-left: _ -> [_]
                          stop <- w1421 stop-if-true
                          n844 = local read "Agilent (Torr)"() -> (w1424:dbl)
                          n845 = Wait (ms)(milliseconds to wait=100) -> ()  [unwired: 1 out]
                          n846 = Less?(x=w1424, y=0.075) -> (x < y?=w1422:bool)
                          n847 = case shown="True" w1422 {
                            selector: w1422 -> [w1425 w1426]
                            tunnel: [w1425 w1426] -> w1419
                            frame False {
                            }
                            frame True {
                              w1428 = FALSE
                              n848 = local write "V17"(w1428) -> ()
                              n849 = local write "V18"(w1428) -> ()
                              n850 = local write "Stop Pump Over"(TRUE) -> ()
                            }
                          }
                          n851 = local read "Stop Pump Over"() -> (w1421:bool)
                        }
                        n852 = local write "Cryo-pull"(FALSE) -> ()
                        n853 = Wait (ms)(milliseconds to wait=1000) -> ()  [unwired: 1 out]
                      }
                      frame #29 {
                        # "Close V16"
                        n854 = local write "Stop Pump Over"(FALSE) -> ()
                        n855 = local write "V16"(FALSE) -> ()
                        n856 = Wait (ms)(milliseconds to wait=1000) -> ()  [unwired: 1 out]
                      }
                      frame #30 {
                        # "Close V4"
                        n857 = local write "V4"(FALSE) -> ()
                        n858 = Wait (ms)(milliseconds to wait=1000) -> ()  [unwired: 1 out]
                      }
                      frame #31 {
                        # "Dewar down"
                        n859 = local write "D"(FALSE) -> ()
                        n860 = Wait (ms)(milliseconds to wait=1000) -> ()  [unwired: 1 out]
                      }
                      frame #32 {
                        # "6 minute thaw"
                        n861 = call "Time Delay11"() -> ()  [unwired: 11 in, 1 out]
                        n862 = local write "Thawing"(TRUE) -> ()
                        n863 = call "Display Message to User4"() -> ()  [unwired: 10 in, 2 out]
                      }
                      frame #33 {
                        n864 = call "Display Message to User7"() -> ()  [unwired: 10 in, 2 out]
                      }
                      frame #34 {
                        # "Read thaw P on Agilent - calculate umol CO2 trapped"
                        n865 = local write "Thawing"(FALSE) -> ()
                        n866 = flat-sequence {
                          frame #0 {
                            n867 = local read "Agilent (Torr)"() -> (w1440:dbl)
                            n868 = local write "Thaw Yield (torr)"(w1440) -> ()
                            n869 = Wait (ms)(milliseconds to wait=200) -> ()  [unwired: 1 out]
                          }
                          frame #1 {
                            # "mol CO2"
                            # "''Cast base units''"
                            # "R"
                            # "V LN2, in m3"
                            # "torr to Pa"
                            n870 = local read "Thaw Yield (torr)"() -> (w1448:dbl)
                            n871 = local read "Temp (K)"() -> (w1441:dbl)
                            n872 = Cast Unit Bases(0:dbl[unit] 8.3144598) -> (2:w1442:dbl)  [unwired: 1 in]
                            n873 = Multiply(x=w1448, y=133.3223684211) -> (x*y=w1447:dbl)
                            n874 = Multiply(x=w1442, y=w1441) -> (x*y=w1446:dbl)
                            n875 = Multiply(x=w1447, y=6.1e-05) -> (x*y=w1452:dbl)
                            n876 = Divide(x=w1452, y=w1446) -> (x/y=w1445:dbl)
                            n877 = Multiply(x=1000000.0, y=w1445) -> (x*y=w1443:dbl)
                            n878 = local write "umol CO2"(w1443) -> ()
                          }
                        }
                        n879 = Wait (ms)(milliseconds to wait=500) -> ()  [unwired: 1 out]
                      }
                      frame #35 {
                        # "P for 400ppm"
                        # "22/4/22\nOffset \nfor extra\nN2 from \nloop"
                        # "Calculate and store Target P"
                        # "''Cast base units''"
                        # "R"
                        # "''Cast base units''"
                        # "R"
                        # "PV=nrt\nP - Pa\nV - m3\nn - mol\nR - \nT - K"
                        # "Pa to mbar"
                        # "P = nRT/V"
                        # "Pa"
                        # "mol N2 to dilute"
                        # "V LN2, flask, bellow in m3"
                        # "ppm"
                        # "n mol N2 = x mol CO2/0.000400"
                        # "0.000400 = x mol CO2/n mol N2"
                        # "mol CO2"
                        # "V LN2, in m3"
                        # "torr to Pa"
                        n880 = local read "Thaw Yield (torr)"() -> (w1472:dbl)
                        n881 = local read "Temp (K)"() -> (w1456:dbl)
                        n882 = Subtract(x=w1472, y=0.2) -> (x-y=w1471:dbl)
                        n883 = Cast Unit Bases(0:dbl[unit] 8.3144598) -> (2:w1463:dbl)  [unwired: 1 in]
                        n884 = Multiply(x=w1471, y=133.3223684211) -> (x*y=w1454:dbl)
                        n885 = Multiply(x=w1463, y=w1456) -> (x*y=w1455:dbl)
                        n886 = Multiply(x=w1454, y=6.1e-05) -> (x*y=w1453:dbl)
                        n887 = Divide(x=w1453, y=w1455) -> (x/y=w1460:dbl)
                        n888 = Divide(x=w1460, y=0.0004) -> (x/y=w1474:dbl)
                        n889 = Cast Unit Bases(0:dbl[unit] 8.3144598) -> (2:w1462:dbl)  [unwired: 1 in]
                        n890 = local read "Temp (K)"() -> (w1459:dbl)
                        n891 = Multiply(x=w1462, y=w1474) -> (x*y=w1458:dbl)
                        n892 = Multiply(x=w1459, y=w1458) -> (x*y=w1457:dbl)
                        n893 = Divide(x=w1457, y=0.000687) -> (x/y=w1461:dbl)
                        n894 = Multiply(x=0.01, y=w1461) -> (x*y=w1475:dbl)
                        n895 = local write "Final Target P (mbar)"(w1475) -> ()
                        n896 = Wait (ms)(milliseconds to wait=200) -> ()  [unwired: 1 out]
                      }
                      frame #36 {
                        # "Calculate Dilution Target Pressure in prep for final expansion"
                        # "Dil. TP fills full MV, V17 closes\n101ml pumped away (all but flask)\n586ml @ Dil. TP expands to 687ml\n--> 687ml @ Final P (P for 400ppm)"
                        # "P1V1 = P2V2\nDTP*586ml = TFP*687ml\nDTP = (FP*687)/586"
                        n897 = local read "Final Target P (mbar)"() -> (w1478:dbl)
                        n898 = Multiply(x=w1478, y=687.0) -> (x*y=w1479:dbl)
                        n899 = Divide(x=w1479, y=586.0) -> (x/y=w1481:dbl)
                        n900 = local write "Dil. Target P (mbar)"(w1481) -> ()
                        n901 = Wait (ms)(milliseconds to wait=200) -> ()  [unwired: 1 out]
                      }
                      frame #37 {
                        # "22/2/22\nAvg of n=2 1500 mbar auto test sloshes:\nn = 3E-6x^2 + 0,003x + 0,0254"
                        # "21/2/22\n1400 mbar auto test sloshes:\nn = 3E-6x^2 + 0,0033x + 0,0268\nn        x (P mbar)\n0        0\n1        232\n2        430\n3        569\n4        733\n5        847"
                        # "8/2/22\n1100 mbar manual sloshes:\nn = 1E-5x^2 + 0,0003x + 0,3052\nn        x (P mbar)\n0        0\n1        205\n2        345\n3        477\n4        587\n5        678\n6        755\n7        819\n8        872\n9        916\n10      951\n11      981"
                        n902 = flat-sequence {
                          frame #0 {
                            # "Currently using avg curve for (Avg(Avg(1500x2),1400))\nn = 3E-6x^2 + 0.0031x + 0.0261"
                            # "Given Dilution Target Pressure, calculate how many sloshes it would take to get \nthe pressure in the full MV to that pressure."
                            n903 = local read "Dil. Target P (mbar)"() -> (w1494:dbl)
                            n904 = local read "Dil. Target P (mbar)"() -> (w1492:dbl)
                            n905 = Square(x=w1494) -> (x^2=w1493:dbl)
                            n906 = Multiply(x=3e-06, y=w1493) -> (x*y=w1490:dbl)
                            n907 = Multiply(x=w1492, y=0.0031) -> (x*y=w1491:dbl)
                            n908 = Add(x=w1490, y=w1491) -> (x+y=w1489:dbl)
                            n909 = Add(x=w1489, y=0.0261) -> (x+y=w1485:dbl)
                            n910 = local write "Exact slosh"(w1485) -> ()
                            n911 = Wait (ms)(milliseconds to wait=100) -> ()  [unwired: 1 out]
                          }
                          frame #1 {
                            # "Now take that calculated number of \nsloshes and round down to nearest integer."
                            n912 = local read "Exact slosh"() -> (w1496:dbl)
                            n913 = Round Toward -Infinity(1:w1496) -> (0:w1497:dbl)
                            n914 = local write "Slosh to do"(w1497) -> ()
                            n915 = Wait (ms)(milliseconds to wait=100) -> ()  [unwired: 1 out]
                          }
                          frame #2 {
                            n916 = local read "Exact slosh"() -> (w1500:dbl)
                            n917 = local read "Slosh to do"() -> (w1499:dbl)
                            n918 = Subtract(x=w1500, y=w1499) -> (x-y=w1501:dbl)
                            n919 = local write "Rem. slosh frac."(w1501) -> ()
                            n920 = Wait (ms)(milliseconds to wait=100) -> ()  [unwired: 1 out]
                          }
                          frame #3 {
                            n921 = local read "Rem. slosh frac."() -> (w1505:dbl)
                            n922 = Multiply(x=1450.0, y=w1505) -> (x*y=w1504:dbl)
                            n923 = local write "P frac. slosh"(w1504) -> ()
                            n924 = Wait (ms)(milliseconds to wait=100) -> ()  [unwired: 1 out]
                          }
                        }
                        n925 = Wait (ms)(milliseconds to wait=200) -> ()  [unwired: 1 out]
                      }
                      frame #38 {
                        # "P should be something like 250mtor (V LN2 ~1/10 of V LN2 + flask)"
                        # "Open, Close V17 - pure CO2 expansion into flask\nEqual concentration of CO2 in LN2, flask, and H of V16/V17"
                        n926 = flat-sequence {
                          frame #0 {
                            n927 = local write "V17"(TRUE) -> ()
                          }
                          frame #1 {
                            n928 = Wait (ms)(milliseconds to wait=u32 40000) -> ()  [unwired: 1 out]
                          }
                          frame #2 {
                            n929 = local write "V17"(FALSE) -> ()
                          }
                        }
                        n930 = Wait (ms)(milliseconds to wait=1000) -> ()  [unwired: 1 out]
                      }
                      frame #39 {
                        # "Close V20"
                        n931 = local write "V20"(FALSE) -> ()
                        n932 = Wait (ms)(milliseconds to wait=1000) -> ()  [unwired: 1 out]
                      }
                      frame #40 {
                        # "Open V8 - begin dilution steps"
                        n933 = local write "Diluting"(TRUE) -> ()
                        n934 = local write "V8"(TRUE) -> ()
                        n935 = Wait (ms)(milliseconds to wait=1000) -> ()  [unwired: 1 out]
                      }
                      frame #41 {
                        # "Open V21"
                        n936 = local write "V21"(TRUE) -> ()
                        n937 = Wait (ms)(milliseconds to wait=1000) -> ()  [unwired: 1 out]
                      }
                      frame #42 {
                        # "Build P in bellow before introducing to LN2 trap w/ sample"
                        n938 = call "Pressurize in LN"() -> ()  [unwired: 11 in, 1 out]
                      }
                      frame #43 {
                        # "Open V18"
                        n939 = local write "V18"(TRUE) -> ()
                        n940 = Wait (ms)(milliseconds to wait=1000) -> ()  [unwired: 1 out]
                      }
                      frame #44 {
                        n941 = local read "Slosh to do"() -> (w1519:dbl)
                        n942 = for {
                          N: w1519 -> [_]
                          n943 = flat-sequence {
                            frame #0 {
                              n944 = while {
                                shift-right: [w1521] -> _
                                shift-left: _ -> [_]
                                stop <- w1522 stop-if-true
                                # "Greater difference in P causes more \nturbulent mixing when expanded into flask"
                                # "When P in bellow + LN2 is > 1450mbar, Open V17"
                                n945 = local read "Pressure (mbar)"() -> (w1524:dbl)
                                n946 = Wait (ms)(milliseconds to wait=100) -> ()  [unwired: 1 out]
                                n947 = Greater?(x=w1524, y=1450.0) -> (0:w1525:bool)
                                n948 = case shown="True" w1525 {
                                selector: w1525 -> [w1526 w1528]
                                tunnel: [w1526 w1528] -> w1521
                                frame False {
                                }
                                frame True {
                                n949 = local write "Stop Sample Pressure"(TRUE) -> ()
                                n950 = local write "V17"(TRUE) -> ()
                                }
                                }
                                n951 = local read "Stop Sample Pressure"() -> (w1522:bool)
                              }
                            }
                            frame #1 {
                              n952 = local read "No. Slosh"() -> (w1530:dbl)
                              n953 = local write "Stop Sample Pressure"(FALSE) -> ()
                              n954 = Increment(x=w1530) -> (x+1=w1531:dbl)
                              n955 = Wait (ms)(milliseconds to wait=4000) -> ()  [unwired: 1 out]
                              n956 = local write "No. Slosh"(w1531) -> ()
                            }
                            frame #2 {
                              n957 = local read "Pressure (mbar)"() -> (w1534:dbl)
                              n958 = local write "Slosh P (mbar)"(w1534) -> ()
                              n959 = Wait (ms)(milliseconds to wait=1000) -> ()  [unwired: 1 out]
                            }
                            frame #3 {
                              n960 = local write "V17"(FALSE) -> ()
                              n961 = Wait (ms)(milliseconds to wait=1000) -> ()  [unwired: 1 out]
                            }
                          }
                        }
                      }
                      frame #45 {
                        # "Check that the final fractional slosh P \nwill be greater P than what's in the \nflask already. If yes, do fractional slosh; \nif no, skip it and go straight to diluting to DTP."
                        n962 = local read "Slosh P (mbar)"() -> (w1540:dbl)
                        n963 = local read "P frac. slosh"() -> (w1539:dbl)
                        n964 = Greater Or Equal?(x=w1539, y=w1540) -> (x >= y?=w1538:bool)
                        n965 = case shown="True" w1538 {
                          frame False {
                            # "Open V17"
                            n966 = local write "V17"(TRUE) -> ()
                            n967 = local read "Dil. Target P (mbar)"() -> (w1542:dbl)
                            n968 = local read "Slosh P (mbar)"() -> (w1541:dbl)
                            n969 = Divide(x=w1541, y=w1542) -> (x/y=w1545:dbl)
                            n970 = Multiply(x=w1545, y=100.0) -> (x*y=w1543:dbl)
                            n971 = local write "Slosh acc. %"(w1543) -> ()
                            n972 = Wait (ms)(milliseconds to wait=1000) -> ()  [unwired: 1 out]
                          }
                          frame True {
                            # "Last slosh into flask, keep V17 open so dilution loop can start right after"
                            n973 = flat-sequence {
                              frame #0 {
                                n974 = local read "Rem. slosh frac."() -> (w1550:dbl)
                                n975 = local read "No. Slosh"() -> (w1551:dbl)
                                n976 = Wait (ms)(milliseconds to wait=100) -> ()  [unwired: 1 out]
                                n977 = Add(x=w1551, y=w1550) -> (x+y=w1549:dbl)
                                n978 = local write "Slosh to do"(w1549) -> ()
                              }
                              frame #1 {
                                n979 = while {
                                shift-right: [w1554] -> _
                                shift-left: _ -> [_]
                                stop <- w1556 stop-if-true
                                # "When P in bellow + LN2 is > fractional slosh P, Open V17"
                                n980 = local read "Pressure (mbar)"() -> (w1557:dbl)
                                n981 = local read "P frac. slosh"() -> (w1552:dbl)
                                n982 = Wait (ms)(milliseconds to wait=100) -> ()  [unwired: 1 out]
                                n983 = Greater Or Equal?(x=w1557, y=w1552) -> (x >= y?=w1555:bool)
                                n984 = case shown="True" w1555 {
                                selector: w1555 -> [w1558 w1559]
                                tunnel: [w1558 w1559] -> w1554
                                frame False {
                                }
                                frame True {
                                n985 = local write "Stop Sample Pressure"(TRUE) -> ()
                                n986 = local write "V17"(TRUE) -> ()
                                }
                                }
                                n987 = local read "Stop Sample Pressure"() -> (w1556:bool)
                                }
                              }
                              frame #2 {
                                n988 = local read "Rem. slosh frac."() -> (w1562:dbl)
                                n989 = local read "No. Slosh"() -> (w1563:dbl)
                                n990 = local write "Stop Sample Pressure"(FALSE) -> ()
                                n991 = Add(x=w1563, y=w1562) -> (x+y=w1564:dbl)
                                n992 = Wait (ms)(milliseconds to wait=5000) -> ()  [unwired: 1 out]
                                n993 = local write "No. Slosh"(w1564) -> ()
                              }
                              frame #3 {
                                n994 = local read "Pressure (mbar)"() -> (w1567:dbl)
                                n995 = local write "Slosh P (mbar)"(w1567) -> ()
                                n996 = Wait (ms)(milliseconds to wait=500) -> ()  [unwired: 1 out]
                              }
                              frame #4 {
                                n997 = local read "Slosh P (mbar)"() -> (w1570:dbl)
                                n998 = local read "Dil. Target P (mbar)"() -> (w1571:dbl)
                                n999 = Divide(x=w1570, y=w1571) -> (x/y=w1574:dbl)
                                n1000 = Multiply(x=w1574, y=100.0) -> (x*y=w1572:dbl)
                                n1001 = local write "Slosh acc. %"(w1572) -> ()
                                n1002 = Wait (ms)(milliseconds to wait=200) -> ()  [unwired: 1 out]
                              }
                            }
                          }
                        }
                      }
                      frame #46 {
                        # "Dil. TP fills full MV, V17 closes\n101ml pumped away (all but flask)\n586ml @ Dil. TP expands to 687ml\n--> 687ml @ Final P (P for 400ppm)"
                        # "Agilent P comes through the DAQ"
                        # "When P Wika = maths for 400ppm dilution, close V8"
                        n1003 = local read "Dil. Target P (mbar)"() -> (w1577:dbl)
                        n1004 = local read "Pressure (mbar)"() -> (w1576:dbl)
                        n1005 = Greater?(x=w1577, y=w1576) -> (0:w1575:bool)
                        n1006 = case shown="True" w1575 {
                          frame False {
                            n1007 = local write "V17"(FALSE) -> ()
                            n1008 = local write "V8"(FALSE) -> ()
                            n1009 = call "Display Message to User8"() -> ()  [unwired: 10 in, 2 out]
                          }
                          frame True {
                            n1010 = while {
                              shift-right: [w1582] -> _
                              shift-left: _ -> [_]
                              i -> [w1592]
                              stop <- w1593 stop-if-true
                              n1011 = local read "Dil. Target P (mbar)"() -> (w1590:dbl)
                              n1012 = local write "Dil. i"(w1592) -> ()
                              n1013 = local read "Pressure (mbar)"() -> (w1589:dbl)
                              n1014 = local read "Pressure (mbar)"() -> (w1587:dbl)
                              n1015 = Add(x=w1587, y=2.0) -> (x+y=w1586:dbl)
                              n1016 = Subtract(x=w1589, y=2.0) -> (x-y=w1585:dbl)
                              n1017 = Wait (ms)(milliseconds to wait=u32 100) -> ()  [unwired: 1 out]
                              n1018 = In Range and Coerce(upper limit=w1586, x=w1590, lower limit=w1585) -> (coerced(x)=w1581:dbl, In Range?=w1588:bool)
                              n1019 = local write "Dilution P (mbar)"(w1581) -> ()
                              n1020 = case shown="True" w1588 {
                                selector: w1588 -> [w1594 w1598]
                                tunnel: [w1594 w1598] -> w1582
                                frame False {
                                }
                                frame True {
                                n1021 = local write "V8"(FALSE) -> ()
                                n1022 = local write "Stop Dilution"(TRUE) -> ()
                                n1023 = local write "V17"(FALSE) -> ()
                                }
                              }
                              n1024 = local read "Stop Dilution"() -> (w1593:bool)
                            }
                          }
                        }
                        n1025 = Wait (ms)(milliseconds to wait=1000) -> ()  [unwired: 1 out]
                      }
                      frame #47 {
                        # "Close V21 - N2 inlet"
                        # "Flask will be over concentrated in CO2 (hopefully somewhere around 480ppm - cant really check that so it's blind)\n19/1/22, 8:00 - Initial manual test of this measured 472ppm on the Licor. Sample expansion and re-dilution that\nfollowed diluted the sample to 397ppm."
                        n1026 = local write "Stop Dilution"(FALSE) -> ()
                        n1027 = local write "Diluting"(FALSE) -> ()
                        n1028 = local write "V21"(FALSE) -> ()
                        n1029 = Wait (ms)(milliseconds to wait=1000) -> ()  [unwired: 1 out]
                      }
                      frame #48 {
                        # "Open V20 - pump out bellow + LN2 trap"
                        n1030 = local write "V20"(TRUE) -> ()
                        n1031 = Wait (ms)(milliseconds to wait=1000) -> ()  [unwired: 1 out]
                      }
                      frame #49 {
                        # "Should already be open anyways"
                        # "Open V18 - pump out bellow + LN2 trap"
                        n1032 = local write "V18"(TRUE) -> ()
                        n1033 = Wait (ms)(milliseconds to wait=1000) -> ()  [unwired: 1 out]
                      }
                      frame #50 {
                        # "Pump excess N2 out from LN2, bellow for 2min"
                        n1034 = call "Time Delay12"() -> ()  [unwired: 11 in, 1 out]
                      }
                      frame #51 {
                        # "Close V20"
                        n1035 = local write "V20"(FALSE) -> ()
                        n1036 = Wait (ms)(milliseconds to wait=1000) -> ()  [unwired: 1 out]
                      }
                      frame #52 {
                        # "Open V17 - expand flask back into LN2 and bellow volume"
                        n1037 = local write "V17"(TRUE) -> ()
                        n1038 = Wait (ms)(milliseconds to wait=15000) -> ()  [unwired: 1 out]
                      }
                      frame #53 {
                        n1039 = local read "Pressure (mbar)"() -> (w1612:dbl)
                        n1040 = call "Convert from Dynamic Data5"("Dynamic Data Type"=w1612) -> ("Array"=w1611:dbl[])  [unwired: 3 in]
                        n1041 = call-poly <vilib>:"Mean.vi"("X"=w1611) -> ("mean"=w1613:dbl)  [unwired: 1 out]
                        n1042 = local write "Final P (mbar)"(w1613) -> ()
                        n1043 = Wait (ms)(milliseconds to wait=200) -> ()  [unwired: 1 out]
                      }
                      frame #54 {
                        n1044 = local read "Final Target P (mbar)"() -> (w1616:dbl)
                        n1045 = local read "Final P (mbar)"() -> (w1615:dbl)
                        n1046 = Divide(x=w1615, y=w1616) -> (x/y=w1617:dbl)
                        n1047 = Multiply(x=w1617, y=100.0) -> (x*y=w1618:dbl)
                        n1048 = local write "Final P Accuracy (%)"(w1618) -> ()
                        n1049 = Wait (ms)(milliseconds to wait=200) -> ()  [unwired: 1 out]
                      }
                      frame #55 {
                        # "Open V16"
                        n1050 = local write "V16"(TRUE) -> ()
                        n1051 = Wait (ms)(milliseconds to wait=1000) -> ()  [unwired: 1 out]
                      }
                      frame #56 {
                        # "Activate circulation loop"
                        n1052 = local write "Circulation Loop"(TRUE) -> ()
                        n1053 = call "Prompt User for Input19"() -> ()  [unwired: 18 in, 2 out]
                        n1054 = Wait (ms)(milliseconds to wait=1000) -> ()  [unwired: 1 out]
                      }
                      frame #57 {
                        # "currently 2,5min"
                        # "Time delay for circulation/mixing"
                        n1055 = call "Time Delay13"() -> ()  [unwired: 11 in, 1 out]
                      }
                      frame #58 {
                        n1056 = call "Prompt User for Input20"() -> ()  [unwired: 18 in, 2 out]
                      }
                      frame #59 {
                        # "Close V16"
                        # "Stop circulation"
                        n1057 = local write "Circulation Loop"(FALSE) -> ()
                        n1058 = local write "V16"(FALSE) -> ()
                        n1059 = Wait (ms)(milliseconds to wait=1000) -> ()  [unwired: 1 out]
                      }
                      frame #60 {
                        n1060 = local write "GO!!!!"(FALSE) -> ()
                        n1061 = local write "Start Sequence"(FALSE) -> ()
                        n1062 = local write "Carbonate Sam"(FALSE) -> ()
                        n1063 = local write "Seq. Finished"(TRUE) -> ()
                      }
                    }
                  }
                }
              }
            }
          }
        }
        n1064 = case shown="True" w77 {
          frame False {
          }
          frame True {
            # "Pretty much if something is wrong from the start it won't pass this 2 second check and save the trouble of dealing with it"
            # "If Current Time is within a 2 second window of \nAnalysis Start Time, run this. If not, do nothing."
            n1065 = local read "Analysis Start Time"() -> (w123:timestamp)
            n1066 = local read "Current Time"() -> (w122:timestamp)
            n1067 = To Double Precision Float(number=w123) -> (double precision float=w124:dbl)
            n1068 = To Double Precision Float(number=w122) -> (double precision float=w125:dbl)
            n1069 = Add(x=w124, y=2.0) -> (x+y=w127:dbl)
            n1070 = Greater?(x=w125, y=w124) -> (0:w128:bool)
            n1071 = Less?(x=w125, y=w127) -> (x < y?=w129:bool)
            n1072 = And(x=w128, y=w129) -> (x .and. y?=w121:bool)
            n1073 = case shown="True" w121 {
              frame False {
              }
              frame True {
                # "Prep atm flask"
                # "Assuming stby start"
                n1074 = stacked-sequence {
                  tunnel: [_ _ _ _ _ _ _ _ _ _ _ _ _ _ _ _ _ _ _ _ _ _ w199 _ _ _ _ _ _ _ _ _ _ _ _ _ _ _ _ _ _ _ _ _ _ _ _ _ _ _ _ _ _ _ _] -> _
                  tunnel: [_ _ _ _ _ _ _ _ _ _ _ _ _ _ _ _ _ _ w194 _ _ _ _ _ _ _ _ _ _ _ _ _ _ _ _ _ _ _ _ _ _ _ _ _ _ _ _ _ _ _ _ _ _ _ _] -> _
                  tunnel: [_ _ _ _ _ _ _ _ _ _ _ _ _ _ _ _ _ _ _ _ _ _ _ _ _ _ _ w220 _ _ _ _ _ _ _ _ _ _ _ _ _ _ _ _ _ _ _ _ _ _ _ _ _ _ _] -> _
                  tunnel: [_ _ _ _ _ _ _ _ _ _ _ _ _ _ _ _ _ _ _ _ _ _ _ _ _ _ _ _ _ _ _ _ _ _ _ _ _ _ _ _ _ _ _ _ _ _ _ _ _ _ w407 _ _ _ _] -> _
                  tunnel: [_ _ _ _ _ _ _ _ _ _ _ _ _ _ _ _ _ _ _ _ _ _ _ _ _ _ _ _ _ _ _ _ _ _ _ _ _ _ _ _ _ _ _ _ _ _ _ _ _ _ _ _ w410 _ _] -> _
                  frame #0 {
                    n1075 = local write "Final Target P (mbar)"(0.0) -> ()
                    n1076 = local write "Final P (mbar)"(0.0) -> ()
                    n1077 = local write "Final P Accuracy (%)"(0.0) -> ()
                    n1078 = local write "Thaw Yield (torr)"(0.0) -> ()
                    n1079 = local write "umol CO2"(0.0) -> ()
                    n1080 = local write "Slosh to do"(0.0) -> ()
                    n1081 = local write "No. Slosh"(0.0) -> ()
                    n1082 = local write "Dil. i"(0.0) -> ()
                    n1083 = local write "Dilution P (mbar)"(0.0) -> ()
                    n1084 = local write "Dil. Target P (mbar)"(0.0) -> ()
                    n1085 = local write "Slosh P (mbar)"(0.0) -> ()
                    n1086 = local write "Slosh acc. %"(0.0) -> ()
                    n1087 = local write "Exact slosh"(0.0) -> ()
                    n1088 = local write "Rem. slosh frac."(0.0) -> ()
                    n1089 = local write "P frac. slosh"(0.0) -> ()
                    n1090 = local write "Temp (K)"(294.0) -> ()
                  }
                  frame #1 {
                    # "V18,17,16,20 should all be open to start"
                    # "Open V7"
                    n1091 = local write "Seq. Finished"(FALSE) -> ()
                    n1092 = local write "V7"(TRUE) -> ()
                    n1093 = Wait (ms)(milliseconds to wait=1000) -> ()  [unwired: 1 out]
                  }
                  frame #2 {
                    # "V18,17,16,20 should all be open to start"
                    # "Open V16"
                    n1094 = local write "V16"(TRUE) -> ()
                    n1095 = Wait (ms)(milliseconds to wait=1000) -> ()  [unwired: 1 out]
                  }
                  frame #3 {
                    # "Close manual valves"
                    n1096 = call "Prompt User for Input10"() -> ()  [unwired: 18 in, 2 out]
                  }
                  frame #4 {
                    # "Open Loop"
                    n1097 = local write "Circulation Loop"(TRUE) -> ()
                    n1098 = local write "Prep. Loop"(TRUE) -> ()
                    n1099 = Wait (ms)(milliseconds to wait=1000) -> ()  [unwired: 1 out]
                  }
                  frame #5 {
                    # "22/4/22 - background ~280 mtorr bg"
                    # "Pump Loop for 60sec"
                    n1100 = call "Time Delay8"() -> ()  [unwired: 11 in, 1 out]
                  }
                  frame #6 {
                    # "Open V8"
                    n1101 = local write "V8"(TRUE) -> ()
                    n1102 = Wait (ms)(milliseconds to wait=1000) -> ()  [unwired: 1 out]
                  }
                  frame #7 {
                    # "Close V20"
                    n1103 = local write "V20"(FALSE) -> ()
                    n1104 = Wait (ms)(milliseconds to wait=1000) -> ()  [unwired: 1 out]
                  }
                  frame #8 {
                    # "Open V21"
                    n1105 = local write "V21"(TRUE) -> ()
                    n1106 = Wait (ms)(milliseconds to wait=1000) -> ()  [unwired: 1 out]
                  }
                  frame #9 {
                    # "When P > 1300 in Loop close V21"
                    n1107 = while {
                      shift-right: [w161] -> _
                      shift-left: _ -> [_]
                      stop <- w162 stop-if-true
                      n1108 = local read "Pressure (mbar)"() -> (w165:dbl)
                      n1109 = Wait (ms)(milliseconds to wait=100) -> ()  [unwired: 1 out]
                      n1110 = Greater?(x=w165, y=1300.0) -> (0:w164:bool)
                      n1111 = case shown="True" w164 {
                        selector: w164 -> [w167 w170]
                        tunnel: [w167 w170] -> w161
                        frame False {
                        }
                        frame True {
                          n1112 = local write "Stop Loop Fill"(TRUE) -> ()
                          n1113 = local write "V21"(FALSE) -> ()
                        }
                      }
                      n1114 = local read "Stop Loop Fill"() -> (w162:bool)
                    }
                    n1115 = Wait (ms)(milliseconds to wait=1000) -> ()  [unwired: 1 out]
                  }
                  frame #10 {
                    n1116 = call "Prompt User for Input11"() -> ()  [unwired: 18 in, 2 out]
                    n1117 = local write "Stop Loop Fill"(FALSE) -> ()
                  }
                  frame #11 {
                    # "Shut Loop"
                    n1118 = local write "Circulation Loop"(FALSE) -> ()
                    n1119 = local write "Prep. Loop"(FALSE) -> ()
                    n1120 = Wait (ms)(milliseconds to wait=1000) -> ()  [unwired: 1 out]
                  }
                  frame #12 {
                    # "Close V8"
                    n1121 = local write "V8"(FALSE) -> ()
                    n1122 = Wait (ms)(milliseconds to wait=1000) -> ()  [unwired: 1 out]
                  }
                  frame #13 {
                    # "Open V20"
                    n1123 = local write "V20"(TRUE) -> ()
                    n1124 = Wait (ms)(milliseconds to wait=1000) -> ()  [unwired: 1 out]
                  }
                  frame #14 {
                    # "When P < 0,076 torr continue w/ sequence"
                    n1125 = while {
                      shift-right: [w180] -> _
                      shift-left: _ -> [_]
                      stop <- w181 stop-if-true
                      n1126 = local read "Agilent (Torr)"() -> (w184:dbl)
                      n1127 = Wait (ms)(milliseconds to wait=100) -> ()  [unwired: 1 out]
                      n1128 = Less?(x=w184, y=0.076) -> (x < y?=w183:bool)
                      n1129 = case shown="True" w183 {
                        selector: w183 -> [w186 w188]
                        tunnel: [w186 w188] -> w180
                        frame False {
                        }
                        frame True {
                          n1130 = local write "Stop Pump Over"(TRUE) -> ()
                        }
                      }
                      n1131 = local read "Stop Pump Over"() -> (w181:bool)
                    }
                    n1132 = Wait (ms)(milliseconds to wait=1000) -> ()  [unwired: 1 out]
                  }
                  frame #15 {
                    n1133 = local write "Stop Pump Over"(FALSE) -> ()
                  }
                  frame #16 {
                    # "Close V16"
                    n1134 = local write "V16"(FALSE) -> ()
                    n1135 = Wait (ms)(milliseconds to wait=1000) -> ()  [unwired: 1 out]
                  }
                  frame #17 {
                    # "Close V17"
                    n1136 = local write "V17"(FALSE) -> ()
                    n1137 = Wait (ms)(milliseconds to wait=1000) -> ()  [unwired: 1 out]
                  }
                  frame #18 {
                    n1138 = call "Prompt User for Input"() -> ("OK"=w194:bool)  [unwired: 18 in, 1 out]
                  }
                  frame #19 {
                    n1139 = Wait (ms)(milliseconds to wait=15000) -> ()  [unwired: 1 out]
                  }
                  frame #20 {
                    # "Dewar up"
                    n1140 = local write "D"(TRUE) -> ()
                    n1141 = Wait (ms)(milliseconds to wait=1000) -> ()  [unwired: 1 out]
                  }
                  frame #21 {
                    # "Give trap 15sec to cool down"
                    n1142 = Wait (ms)(milliseconds to wait=15000) -> ()  [unwired: 1 out]
                  }
                  frame #22 {
                    n1143 = call "Prompt User for Input2"() -> ("OK"=w199:bool)  [unwired: 18 in, 1 out]
                  }
                  frame #23 {
                    # "Open V17"
                    n1144 = local write "V17"(TRUE) -> ()
                    n1145 = Wait (ms)(milliseconds to wait=1000) -> ()  [unwired: 1 out]
                  }
                  frame #24 {
                    # "When P < 0,09 torr close off LN2 trap"
                    n1146 = while {
                      shift-right: [w209] -> _
                      shift-left: _ -> [_]
                      stop <- w208 stop-if-true
                      n1147 = local read "Agilent (Torr)"() -> (w206:dbl)
                      n1148 = Wait (ms)(milliseconds to wait=100) -> ()  [unwired: 1 out]
                      n1149 = Less?(x=w206, y=0.09) -> (x < y?=w205:bool)
                      n1150 = case shown="True" w205 {
                        selector: w205 -> [w210 w214]
                        tunnel: [w210 w214] -> w209
                        frame False {
                        }
                        frame True {
                          n1151 = local write "V18"(FALSE) -> ()
                          n1152 = local write "V17"(FALSE) -> ()
                          n1153 = local write "Stop Pump Over"(TRUE) -> ()
                        }
                      }
                      n1154 = local read "Stop Pump Over"() -> (w208:bool)
                    }
                    n1155 = local write "Cryo-pull"(TRUE) -> ()
                    n1156 = Wait (ms)(milliseconds to wait=1000) -> ()  [unwired: 1 out]
                  }
                  frame #25 {
                    # "Dewar down"
                    n1157 = local write "Cryo-pull"(FALSE) -> ()
                    n1158 = local write "Stop Pump Over"(FALSE) -> ()
                    n1159 = local write "D"(FALSE) -> ()
                    n1160 = Wait (ms)(milliseconds to wait=1000) -> ()  [unwired: 1 out]
                  }
                  frame #26 {
                    # "6 minute thaw"
                    n1161 = call "Time Delay4"() -> ()  [unwired: 11 in, 1 out]
                    n1162 = local write "Thawing"(TRUE) -> ()
                  }
                  frame #27 {
                    n1163 = call "Prompt User for Input12"() -> ("OK"=w220:bool)  [unwired: 18 in, 1 out]
                  }
                  frame #28 {
                    # "Read thaw P on Agilent - calculate umol CO2 trapped"
                    n1164 = local write "Thawing"(FALSE) -> ()
                    n1165 = flat-sequence {
                      frame #0 {
                        n1166 = local read "Agilent (Torr)"() -> (w224:dbl)
                        n1167 = local write "Thaw Yield (torr)"(w224) -> ()
                        n1168 = Wait (ms)(milliseconds to wait=200) -> ()  [unwired: 1 out]
                      }
                      frame #1 {
                        # "mol CO2"
                        # "''Cast base units''"
                        # "R"
                        # "V LN2, in m3"
                        # "torr to Pa"
                        n1169 = local read "Thaw Yield (torr)"() -> (w232:dbl)
                        n1170 = local read "Temp (K)"() -> (w225:dbl)
                        n1171 = Cast Unit Bases(0:dbl[unit] 8.3144598) -> (2:w226:dbl)  [unwired: 1 in]
                        n1172 = Multiply(x=w232, y=133.3223684211) -> (x*y=w231:dbl)
                        n1173 = Multiply(x=w226, y=w225) -> (x*y=w230:dbl)
                        n1174 = Multiply(x=w231, y=6.1e-05) -> (x*y=w236:dbl)
                        n1175 = Divide(x=w236, y=w230) -> (x/y=w229:dbl)
                        n1176 = Multiply(x=1000000.0, y=w229) -> (x*y=w227:dbl)
                        n1177 = local write "umol CO2"(w227) -> ()
                      }
                    }
                    n1178 = Wait (ms)(milliseconds to wait=500) -> ()  [unwired: 1 out]
                  }
                  frame #29 {
                    # "P for 400ppm"
                    # "22/4/22\nOffset \nfor extra\nN2 from \nloop"
                    # "Calculate and store Target P"
                    # "''Cast base units''"
                    # "R"
                    # "''Cast base units''"
                    # "R"
                    # "PV=nrt\nP - Pa\nV - m3\nn - mol\nR - \nT - K"
                    # "Pa to mbar"
                    # "P = nRT/V"
                    # "Pa"
                    # "mol N2 to dilute"
                    # "V LN2, flask, bellow in m3"
                    # "ppm"
                    # "n mol N2 = x mol CO2/0.000400"
                    # "0.000400 = x mol CO2/n mol N2"
                    # "mol CO2"
                    # "V LN2, in m3"
                    # "torr to Pa"
                    n1179 = local read "Thaw Yield (torr)"() -> (w256:dbl)
                    n1180 = local read "Temp (K)"() -> (w240:dbl)
                    n1181 = Subtract(x=w256, y=0.2) -> (x-y=w255:dbl)
                    n1182 = Cast Unit Bases(0:dbl[unit] 8.3144598) -> (2:w247:dbl)  [unwired: 1 in]
                    n1183 = Multiply(x=w255, y=133.3223684211) -> (x*y=w238:dbl)
                    n1184 = Multiply(x=w247, y=w240) -> (x*y=w239:dbl)
                    n1185 = Multiply(x=w238, y=6.1e-05) -> (x*y=w237:dbl)
                    n1186 = Divide(x=w237, y=w239) -> (x/y=w244:dbl)
                    n1187 = Divide(x=w244, y=0.0004) -> (x/y=w258:dbl)
                    n1188 = Cast Unit Bases(0:dbl[unit] 8.3144598) -> (2:w246:dbl)  [unwired: 1 in]
                    n1189 = local read "Temp (K)"() -> (w243:dbl)
                    n1190 = Multiply(x=w246, y=w258) -> (x*y=w242:dbl)
                    n1191 = Multiply(x=w243, y=w242) -> (x*y=w241:dbl)
                    n1192 = Divide(x=w241, y=0.000687) -> (x/y=w245:dbl)
                    n1193 = Multiply(x=0.01, y=w245) -> (x*y=w259:dbl)
                    n1194 = local write "Final Target P (mbar)"(w259) -> ()
                    n1195 = Wait (ms)(milliseconds to wait=200) -> ()  [unwired: 1 out]
                  }
                  frame #30 {
                    # "Calculate Dilution Target Pressure in prep for final expansion"
                    # "Dil. TP fills full MV, V17 closes\n101ml pumped away (all but flask)\n586ml @ Dil. TP expands to 687ml\n--> 687ml @ Final P (P for 400ppm)"
                    # "P1V1 = P2V2\nDTP*586ml = TFP*687ml\nDTP = (FP*687)/586"
                    n1196 = local read "Final Target P (mbar)"() -> (w262:dbl)
                    n1197 = Multiply(x=w262, y=687.0) -> (x*y=w263:dbl)
                    n1198 = Divide(x=w263, y=586.0) -> (x/y=w265:dbl)
                    n1199 = local write "Dil. Target P (mbar)"(w265) -> ()
                    n1200 = Wait (ms)(milliseconds to wait=200) -> ()  [unwired: 1 out]
                  }
                  frame #31 {
                    # "22/2/22\nAvg of n=2 1500 mbar auto test sloshes:\nn = 3E-6x^2 + 0,003x + 0,0254"
                    # "21/2/22\n1400 mbar auto test sloshes:\nn = 3E-6x^2 + 0,0033x + 0,0268\nn        x (P mbar)\n0        0\n1        232\n2        430\n3        569\n4        733\n5        847"
                    # "8/2/22\n1100 mbar manual sloshes:\nn = 1E-5x^2 + 0,0003x + 0,3052\nn        x (P mbar)\n0        0\n1        205\n2        345\n3        477\n4        587\n5        678\n6        755\n7        819\n8        872\n9        916\n10      951\n11      981"
                    n1201 = flat-sequence {
                      frame #0 {
                        # "Currently using avg curve for (Avg(Avg(1500x2),1400))\nn = 3E-6x^2 + 0.0031x + 0.0261"
                        # "Given Dilution Target Pressure, calculate how many sloshes it would take to get \nthe pressure in the full MV to that pressure."
                        n1202 = local read "Dil. Target P (mbar)"() -> (w278:dbl)
                        n1203 = local read "Dil. Target P (mbar)"() -> (w276:dbl)
                        n1204 = Square(x=w278) -> (x^2=w277:dbl)
                        n1205 = Multiply(x=3e-06, y=w277) -> (x*y=w274:dbl)
                        n1206 = Multiply(x=w276, y=0.0031) -> (x*y=w275:dbl)
                        n1207 = Add(x=w274, y=w275) -> (x+y=w273:dbl)
                        n1208 = Add(x=w273, y=0.0261) -> (x+y=w269:dbl)
                        n1209 = local write "Exact slosh"(w269) -> ()
                        n1210 = Wait (ms)(milliseconds to wait=100) -> ()  [unwired: 1 out]
                      }
                      frame #1 {
                        # "Now take that calculated number of \nsloshes and round down to nearest integer."
                        n1211 = local read "Exact slosh"() -> (w280:dbl)
                        n1212 = Round Toward -Infinity(1:w280) -> (0:w281:dbl)
                        n1213 = local write "Slosh to do"(w281) -> ()
                        n1214 = Wait (ms)(milliseconds to wait=100) -> ()  [unwired: 1 out]
                      }
                      frame #2 {
                        n1215 = local read "Exact slosh"() -> (w284:dbl)
                        n1216 = local read "Slosh to do"() -> (w283:dbl)
                        n1217 = Subtract(x=w284, y=w283) -> (x-y=w285:dbl)
                        n1218 = local write "Rem. slosh frac."(w285) -> ()
                        n1219 = Wait (ms)(milliseconds to wait=100) -> ()  [unwired: 1 out]
                      }
                      frame #3 {
                        n1220 = local read "Rem. slosh frac."() -> (w289:dbl)
                        n1221 = Multiply(x=1450.0, y=w289) -> (x*y=w288:dbl)
                        n1222 = local write "P frac. slosh"(w288) -> ()
                        n1223 = Wait (ms)(milliseconds to wait=100) -> ()  [unwired: 1 out]
                      }
                    }
                    n1224 = Wait (ms)(milliseconds to wait=200) -> ()  [unwired: 1 out]
                  }
                  frame #32 {
                    # "Open, Close V17 - pure CO2 expansion into flask\nEqual concentration of CO2 in LN2, flask, and H of V16/V17"
                    n1225 = flat-sequence {
                      frame #0 {
                        n1226 = local write "V17"(TRUE) -> ()
                      }
                      frame #1 {
                        n1227 = Wait (ms)(milliseconds to wait=u32 40000) -> ()  [unwired: 1 out]
                      }
                      frame #2 {
                        n1228 = local write "V17"(FALSE) -> ()
                      }
                    }
                    n1229 = Wait (ms)(milliseconds to wait=1000) -> ()  [unwired: 1 out]
                  }
                  frame #33 {
                    # "Close V20"
                    n1230 = local write "V20"(FALSE) -> ()
                    n1231 = Wait (ms)(milliseconds to wait=1000) -> ()  [unwired: 1 out]
                  }
                  frame #34 {
                    # "Open V8 - begin dilution steps"
                    n1232 = local write "Diluting"(TRUE) -> ()
                    n1233 = local write "V8"(TRUE) -> ()
                    n1234 = Wait (ms)(milliseconds to wait=1000) -> ()  [unwired: 1 out]
                  }
                  frame #35 {
                    # "Open V21"
                    n1235 = local write "V21"(TRUE) -> ()
                    n1236 = Wait (ms)(milliseconds to wait=1000) -> ()  [unwired: 1 out]
                  }
                  frame #36 {
                    # "Build P in bellow before introducing to LN2 trap w/ sample"
                    n1237 = call "Pressurize in LN5"() -> ()  [unwired: 11 in, 1 out]
                  }
                  frame #37 {
                    # "Open V18"
                    n1238 = local write "V18"(TRUE) -> ()
                    n1239 = Wait (ms)(milliseconds to wait=1000) -> ()  [unwired: 1 out]
                  }
                  frame #38 {
                    n1240 = local read "Slosh to do"() -> (w303:dbl)
                    n1241 = for {
                      N: w303 -> [_]
                      n1242 = flat-sequence {
                        frame #0 {
                          n1243 = while {
                            shift-right: [w305] -> _
                            shift-left: _ -> [_]
                            stop <- w306 stop-if-true
                            # "Greater difference in P causes more \nturbulent mixing when expanded into flask"
                            # "When P in bellow + LN2 is > 1450mbar, Open V17"
                            n1244 = local read "Pressure (mbar)"() -> (w308:dbl)
                            n1245 = Wait (ms)(milliseconds to wait=100) -> ()  [unwired: 1 out]
                            n1246 = Greater?(x=w308, y=1450.0) -> (0:w309:bool)
                            n1247 = case shown="True" w309 {
                              selector: w309 -> [w310 w312]
                              tunnel: [w310 w312] -> w305
                              frame False {
                              }
                              frame True {
                                n1248 = local write "Stop Sample Pressure"(TRUE) -> ()
                                n1249 = local write "V17"(TRUE) -> ()
                              }
                            }
                            n1250 = local read "Stop Sample Pressure"() -> (w306:bool)
                          }
                        }
                        frame #1 {
                          n1251 = local read "No. Slosh"() -> (w314:dbl)
                          n1252 = local write "Stop Sample Pressure"(FALSE) -> ()
                          n1253 = Increment(x=w314) -> (x+1=w315:dbl)
                          n1254 = Wait (ms)(milliseconds to wait=4000) -> ()  [unwired: 1 out]
                          n1255 = local write "No. Slosh"(w315) -> ()
                        }
                        frame #2 {
                          n1256 = local read "Pressure (mbar)"() -> (w318:dbl)
                          n1257 = local write "Slosh P (mbar)"(w318) -> ()
                          n1258 = Wait (ms)(milliseconds to wait=1000) -> ()  [unwired: 1 out]
                        }
                        frame #3 {
                          n1259 = local write "V17"(FALSE) -> ()
                          n1260 = Wait (ms)(milliseconds to wait=1000) -> ()  [unwired: 1 out]
                        }
                      }
                    }
                  }
                  frame #39 {
                    # "Check that the final fractional slosh P \nwill be greater P than what's in the \nflask already. If yes, do fractional slosh; \nif no, skip it and go straight to diluting to DTP."
                    n1261 = local read "Slosh P (mbar)"() -> (w324:dbl)
                    n1262 = local read "P frac. slosh"() -> (w323:dbl)
                    n1263 = Greater Or Equal?(x=w323, y=w324) -> (x >= y?=w322:bool)
                    n1264 = case shown="True" w322 {
                      frame False {
                        # "Open V17"
                        n1265 = local write "V17"(TRUE) -> ()
                        n1266 = local read "Dil. Target P (mbar)"() -> (w326:dbl)
                        n1267 = local read "Slosh P (mbar)"() -> (w325:dbl)
                        n1268 = Divide(x=w325, y=w326) -> (x/y=w329:dbl)
                        n1269 = Multiply(x=w329, y=100.0) -> (x*y=w327:dbl)
                        n1270 = local write "Slosh acc. %"(w327) -> ()
                        n1271 = Wait (ms)(milliseconds to wait=1000) -> ()  [unwired: 1 out]
                      }
                      frame True {
                        # "Last slosh into flask, keep V17 open so dilution loop can start right after"
                        n1272 = flat-sequence {
                          frame #0 {
                            n1273 = local read "Rem. slosh frac."() -> (w334:dbl)
                            n1274 = local read "No. Slosh"() -> (w335:dbl)
                            n1275 = Wait (ms)(milliseconds to wait=100) -> ()  [unwired: 1 out]
                            n1276 = Add(x=w335, y=w334) -> (x+y=w333:dbl)
                            n1277 = local write "Slosh to do"(w333) -> ()
                          }
                          frame #1 {
                            n1278 = while {
                              shift-right: [w338] -> _
                              shift-left: _ -> [_]
                              stop <- w340 stop-if-true
                              # "When P in bellow + LN2 is > fractional slosh P, Open V17"
                              n1279 = local read "Pressure (mbar)"() -> (w341:dbl)
                              n1280 = local read "P frac. slosh"() -> (w336:dbl)
                              n1281 = Wait (ms)(milliseconds to wait=100) -> ()  [unwired: 1 out]
                              n1282 = Greater Or Equal?(x=w341, y=w336) -> (x >= y?=w339:bool)
                              n1283 = case shown="True" w339 {
                                selector: w339 -> [w342 w343]
                                tunnel: [w342 w343] -> w338
                                frame False {
                                }
                                frame True {
                                n1284 = local write "Stop Sample Pressure"(TRUE) -> ()
                                n1285 = local write "V17"(TRUE) -> ()
                                }
                              }
                              n1286 = local read "Stop Sample Pressure"() -> (w340:bool)
                            }
                          }
                          frame #2 {
                            n1287 = local read "Rem. slosh frac."() -> (w346:dbl)
                            n1288 = local read "No. Slosh"() -> (w347:dbl)
                            n1289 = local write "Stop Sample Pressure"(FALSE) -> ()
                            n1290 = Add(x=w347, y=w346) -> (x+y=w348:dbl)
                            n1291 = Wait (ms)(milliseconds to wait=5000) -> ()  [unwired: 1 out]
                            n1292 = local write "No. Slosh"(w348) -> ()
                          }
                          frame #3 {
                            n1293 = local read "Pressure (mbar)"() -> (w351:dbl)
                            n1294 = local write "Slosh P (mbar)"(w351) -> ()
                            n1295 = Wait (ms)(milliseconds to wait=500) -> ()  [unwired: 1 out]
                          }
                          frame #4 {
                            n1296 = local read "Slosh P (mbar)"() -> (w354:dbl)
                            n1297 = local read "Dil. Target P (mbar)"() -> (w355:dbl)
                            n1298 = Divide(x=w354, y=w355) -> (x/y=w358:dbl)
                            n1299 = Multiply(x=w358, y=100.0) -> (x*y=w356:dbl)
                            n1300 = local write "Slosh acc. %"(w356) -> ()
                            n1301 = Wait (ms)(milliseconds to wait=200) -> ()  [unwired: 1 out]
                          }
                        }
                      }
                    }
                  }
                  frame #40 {
                    # "Dil. TP fills full MV, V17 closes\n101ml pumped away (all but flask)\n586ml @ Dil. TP expands to 687ml\n--> 687ml @ Final P (P for 400ppm)"
                    # "Agilent P comes through the DAQ"
                    # "When P Wika = maths for 400ppm dilution, close V8"
                    n1302 = local read "Dil. Target P (mbar)"() -> (w361:dbl)
                    n1303 = local read "Pressure (mbar)"() -> (w360:dbl)
                    n1304 = Greater?(x=w361, y=w360) -> (0:w359:bool)
                    n1305 = case shown="True" w359 {
                      frame False {
                        n1306 = local write "V17"(FALSE) -> ()
                        n1307 = local write "V8"(FALSE) -> ()
                        n1308 = call "Display Message to User3"() -> ()  [unwired: 10 in, 2 out]
                      }
                      frame True {
                        n1309 = while {
                          shift-right: [w366] -> _
                          shift-left: _ -> [_]
                          i -> [w376]
                          stop <- w377 stop-if-true
                          n1310 = local read "Dil. Target P (mbar)"() -> (w374:dbl)
                          n1311 = local write "Dil. i"(w376) -> ()
                          n1312 = local read "Pressure (mbar)"() -> (w373:dbl)
                          n1313 = local read "Pressure (mbar)"() -> (w371:dbl)
                          n1314 = Add(x=w371, y=2.0) -> (x+y=w370:dbl)
                          n1315 = Subtract(x=w373, y=2.0) -> (x-y=w369:dbl)
                          n1316 = Wait (ms)(milliseconds to wait=u32 100) -> ()  [unwired: 1 out]
                          n1317 = In Range and Coerce(upper limit=w370, x=w374, lower limit=w369) -> (coerced(x)=w365:dbl, In Range?=w372:bool)
                          n1318 = local write "Dilution P (mbar)"(w365) -> ()
                          n1319 = case shown="True" w372 {
                            selector: w372 -> [w378 w382]
                            tunnel: [w378 w382] -> w366
                            frame False {
                            }
                            frame True {
                              n1320 = local write "V8"(FALSE) -> ()
                              n1321 = local write "Stop Dilution"(TRUE) -> ()
                              n1322 = local write "V17"(FALSE) -> ()
                            }
                          }
                          n1323 = local read "Stop Dilution"() -> (w377:bool)
                        }
                      }
                    }
                    n1324 = Wait (ms)(milliseconds to wait=1000) -> ()  [unwired: 1 out]
                  }
                  frame #41 {
                    # "Close V21 - N2 inlet - want to keep this volume under superambient pressure always"
                    # "Flask will be over concentrated in CO2 (hopefully somewhere around 480ppm - cant really check that so it's blind)\n19/1/22, 8:00 - Initial manual test of this measured 472ppm on the Licor. Sample expansion and re-dilution that\nfollowed diluted the sample to 397ppm."
                    n1325 = local write "Stop Dilution"(FALSE) -> ()
                    n1326 = local write "Diluting"(FALSE) -> ()
                    n1327 = local write "V21"(FALSE) -> ()
                    n1328 = Wait (ms)(milliseconds to wait=1000) -> ()  [unwired: 1 out]
                  }
                  frame #42 {
                    # "Open V20 - pump out bellow + LN2 trap"
                    n1329 = local write "V20"(TRUE) -> ()
                    n1330 = Wait (ms)(milliseconds to wait=1000) -> ()  [unwired: 1 out]
                  }
                  frame #43 {
                    # "Should already be open anyways"
                    # "Open V18 - pump out bellow + LN2 trap"
                    n1331 = local write "V18"(TRUE) -> ()
                    n1332 = Wait (ms)(milliseconds to wait=1000) -> ()  [unwired: 1 out]
                  }
                  frame #44 {
                    # "Pump excess N2 out from LN2, bellow for 2min"
                    n1333 = call "Time Delay5"() -> ()  [unwired: 11 in, 1 out]
                  }
                  frame #45 {
                    # "Close V20"
                    n1334 = local write "V20"(FALSE) -> ()
                    n1335 = Wait (ms)(milliseconds to wait=1000) -> ()  [unwired: 1 out]
                  }
                  frame #46 {
                    # "Open V17 - expand flask back into LN2 and bellow volume"
                    n1336 = local write "V17"(TRUE) -> ()
                    n1337 = Wait (ms)(milliseconds to wait=15000) -> ()  [unwired: 1 out]
                  }
                  frame #47 {
                    n1338 = local read "Pressure (mbar)"() -> (w396:dbl)
                    n1339 = call "Convert from Dynamic Data4"("Dynamic Data Type"=w396) -> ("Array"=w395:dbl[])  [unwired: 3 in]
                    n1340 = call-poly <vilib>:"Mean.vi"("X"=w395) -> ("mean"=w397:dbl)  [unwired: 1 out]
                    n1341 = local write "Final P (mbar)"(w397) -> ()
                    n1342 = Wait (ms)(milliseconds to wait=200) -> ()  [unwired: 1 out]
                  }
                  frame #48 {
                    n1343 = local read "Final Target P (mbar)"() -> (w400:dbl)
                    n1344 = local read "Final P (mbar)"() -> (w399:dbl)
                    n1345 = Divide(x=w399, y=w400) -> (x/y=w401:dbl)
                    n1346 = Multiply(x=w401, y=100.0) -> (x*y=w402:dbl)
                    n1347 = local write "Final P Accuracy (%)"(w402) -> ()
                    n1348 = Wait (ms)(milliseconds to wait=200) -> ()  [unwired: 1 out]
                  }
                  frame #49 {
                    # "Open V16"
                    n1349 = local write "V16"(TRUE) -> ()
                    n1350 = Wait (ms)(milliseconds to wait=1000) -> ()  [unwired: 1 out]
                  }
                  frame #50 {
                    # "Activate circulation loop"
                    n1351 = local write "Circulation Loop"(TRUE) -> ()
                    n1352 = call "Prompt User for Input13"() -> ("OK"=w407:bool)  [unwired: 18 in, 1 out]
                    n1353 = Wait (ms)(milliseconds to wait=1000) -> ()  [unwired: 1 out]
                  }
                  frame #51 {
                    # "currently 2,5min"
                    # "Time delay for circulation/mixing"
                    n1354 = call "Time Delay9"() -> ()  [unwired: 11 in, 1 out]
                  }
                  frame #52 {
                    n1355 = call "Prompt User for Input14"() -> ("OK"=w410:bool)  [unwired: 18 in, 1 out]
                  }
                  frame #53 {
                    # "Close V16"
                    # "Stop circulation"
                    n1356 = local write "Circulation Loop"(FALSE) -> ()
                    n1357 = local write "V16"(FALSE) -> ()
                    n1358 = Wait (ms)(milliseconds to wait=1000) -> ()  [unwired: 1 out]
                  }
                  frame #54 {
                    n1359 = local write "GO!!!!"(FALSE) -> ()
                    n1360 = local write "Start Sequence"(FALSE) -> ()
                    n1361 = local write "Seq. Finished"(TRUE) -> ()
                    n1362 = local write "Atm Flask"(FALSE) -> ()
                  }
                }
              }
            }
          }
        }
        n1363 = case shown="True" w76 {
          frame False {
          }
          frame True {
            # "Pretty much if something is wrong from the start it won't pass this 2 second check and save the trouble of dealing with it"
            # "I suppose for super super small samples could do a \nslosh seq that doesn't use flask, just b/w LN2 + bellow\n6 aliquots = 1030mbar, 0.18mg CaCO3\nWould have to re-plumb LN2 trap to push sam to bellow"
            # "For 13 aliquots into TILDAS, need 575mbar of mixed sam.\n575mbar = 6.62umol CO2 = 0.663mg CaCO3 = 1.99 torr\nyield during thaw. \n11 aliquots = 544mbar, 12 aliquots = 559mbar needed.\n5 aliquots = 460mbar, 7 aliquots = 487mbar"
            # "If Current Time is within a 2 second window of \nAnalysis Start Time, run this. If not, do nothing."
            n1364 = local read "Analysis Start Time"() -> (w421:timestamp)
            n1365 = local read "Current Time"() -> (w420:timestamp)
            n1366 = To Double Precision Float(number=w421) -> (double precision float=w419:dbl)
            n1367 = To Double Precision Float(number=w420) -> (double precision float=w422:dbl)
            n1368 = Add(x=w419, y=2.0) -> (x+y=w424:dbl)
            n1369 = Greater?(x=w422, y=w419) -> (0:w425:bool)
            n1370 = Less?(x=w422, y=w424) -> (x < y?=w426:bool)
            n1371 = And(x=w425, y=w426) -> (x .and. y?=w418:bool)
            n1372 = case shown="True" w418 {
              frame False {
              }
              frame True {
                # "Prep carbonate samples"
                # "Assuming stby start"
                n1373 = stacked-sequence {
                  tunnel: [_ _ _ _ _ _ _ _ _ _ _ _ _ _ _ w489 _ _ _ _ _ _ _ _ _ _ _ _ _ _ _ _ _ _ _ _ _ _ _ _ _ _ _ _ _ _ _ _ _ _ _ _ _ _ _ _] -> _
                  tunnel: [_ _ _ _ _ _ _ _ _ _ _ _ _ _ _ _ _ _ _ w494 _ _ _ _ _ _ _ _ _ _ _ _ _ _ _ _ _ _ _ _ _ _ _ _ _ _ _ _ _ _ _ _ _ _ _ _] -> _
                  tunnel: [_ _ _ _ _ _ _ _ _ _ _ _ _ _ _ _ _ _ _ _ _ _ _ _ w503 _ _ _ _ _ _ _ _ _ _ _ _ _ _ _ _ _ _ _ _ _ _ _ _ _ _ _ _ _ _ _] -> _
                  tunnel: [_ _ _ w448 _ _ _ _ _ _ _ _ _ _ _ _ _ _ _ _ _ _ _ _ _ _ _ _ _ _ _ _ _ _ _ _ _ _ _ _ _ _ _ _ _ _ _ _ _ _ _ _ _ _ _ _] -> _
                  tunnel: [_ _ _ _ _ _ _ _ _ _ _ _ _ _ _ _ _ _ _ _ _ _ _ _ _ _ _ _ _ _ _ _ _ _ _ _ _ _ _ _ _ _ _ _ _ _ _ _ _ _ _ w712 _ _ _ _] -> _
                  tunnel: [_ _ _ _ _ _ _ _ _ _ _ _ _ _ _ _ _ _ _ _ _ _ _ _ _ _ _ _ _ _ _ _ _ _ _ _ _ _ _ _ _ _ _ _ _ _ _ _ _ _ _ _ _ w714 _ _] -> _
                  tunnel: [_ _ _ _ _ _ _ _ _ _ w470 _ _ _ _ _ _ _ _ _ _ _ _ _ _ _ _ _ _ _ _ _ _ _ _ _ _ _ _ _ _ _ _ _ _ _ _ _ _ _ _ _ _ _ _ _] -> _
                  frame #0 {
                    n1374 = local write "Final Target P (mbar)"(0.0) -> ()
                    n1375 = local write "Final P Accuracy (%)"(0.0) -> ()
                    n1376 = local write "Thaw Yield (torr)"(0.0) -> ()
                    n1377 = local write "Final P (mbar)"(0.0) -> ()
                    n1378 = local write "Slosh to do"(0.0) -> ()
                    n1379 = local write "umol CO2"(0.0) -> ()
                    n1380 = local write "No. Slosh"(0.0) -> ()
                    n1381 = local write "Dil. i"(0.0) -> ()
                    n1382 = local write "Dil. Target P (mbar)"(0.0) -> ()
                    n1383 = local write "Dilution P (mbar)"(0.0) -> ()
                    n1384 = local write "Rem. slosh frac."(0.0) -> ()
                    n1385 = local write "Slosh P (mbar)"(0.0) -> ()
                    n1386 = local write "Slosh acc. %"(0.0) -> ()
                    n1387 = local write "P frac. slosh"(0.0) -> ()
                    n1388 = local write "Exact slosh"(0.0) -> ()
                    n1389 = local write "Temp (K)"(294.0) -> ()
                  }
                  frame #1 {
                    # "V18,17,16,20 should all be open to start"
                    # "Open V7"
                    n1390 = local write "V7"(TRUE) -> ()
                    n1391 = local write "Seq. Finished"(FALSE) -> ()
                    n1392 = Wait (ms)(milliseconds to wait=1000) -> ()  [unwired: 1 out]
                  }
                  frame #2 {
                    # "V18,17,16,20 should all be open to start"
                    # "Open V16"
                    n1393 = local write "V16"(TRUE) -> ()
                    n1394 = Wait (ms)(milliseconds to wait=1000) -> ()  [unwired: 1 out]
                  }
                  frame #3 {
                    # "Close flask valves"
                    n1395 = call "Prompt User for Input5"() -> ("OK"=w448:bool)  [unwired: 18 in, 1 out]
                  }
                  frame #4 {
                    # "Open Loop"
                    n1396 = local write "Circulation Loop"(TRUE) -> ()
                    n1397 = local write "Prep. Loop"(TRUE) -> ()
                    n1398 = Wait (ms)(milliseconds to wait=1000) -> ()  [unwired: 1 out]
                  }
                  frame #5 {
                    # "22/4/22 - background ~280 mtorr bg"
                    # "Pump Loop for 60sec"
                    n1399 = call "Time Delay7"() -> ()  [unwired: 11 in, 1 out]
                  }
                  frame #6 {
                    # "Open V8"
                    n1400 = local write "V8"(TRUE) -> ()
                    n1401 = Wait (ms)(milliseconds to wait=1000) -> ()  [unwired: 1 out]
                  }
                  frame #7 {
                    # "Close V20"
                    n1402 = local write "V20"(FALSE) -> ()
                    n1403 = Wait (ms)(milliseconds to wait=1000) -> ()  [unwired: 1 out]
                  }
                  frame #8 {
                    # "Open V21"
                    n1404 = local write "V21"(TRUE) -> ()
                    n1405 = Wait (ms)(milliseconds to wait=1000) -> ()  [unwired: 1 out]
                  }
                  frame #9 {
                    # "When P > 1300 in Loop close V21"
                    n1406 = while {
                      shift-right: [w459] -> _
                      shift-left: _ -> [_]
                      stop <- w460 stop-if-true
                      n1407 = local read "Pressure (mbar)"() -> (w463:dbl)
                      n1408 = Wait (ms)(milliseconds to wait=100) -> ()  [unwired: 1 out]
                      n1409 = Greater?(x=w463, y=1300.0) -> (0:w462:bool)
                      n1410 = case shown="True" w462 {
                        selector: w462 -> [w465 w468]
                        tunnel: [w465 w468] -> w459
                        frame False {
                        }
                        frame True {
                          n1411 = local write "Stop Loop Fill"(TRUE) -> ()
                          n1412 = local write "V21"(FALSE) -> ()
                        }
                      }
                      n1413 = local read "Stop Loop Fill"() -> (w460:bool)
                    }
                    n1414 = Wait (ms)(milliseconds to wait=1000) -> ()  [unwired: 1 out]
                  }
                  frame #10 {
                    n1415 = call "Prompt User for Input9"() -> ("OK"=w470:bool)  [unwired: 18 in, 1 out]
                    n1416 = local write "Stop Loop Fill"(FALSE) -> ()
                  }
                  frame #11 {
                    # "Shut Loop"
                    n1417 = local write "Circulation Loop"(FALSE) -> ()
                    n1418 = local write "Prep. Loop"(FALSE) -> ()
                    n1419 = Wait (ms)(milliseconds to wait=1000) -> ()  [unwired: 1 out]
                  }
                  frame #12 {
                    # "Close V8"
                    n1420 = local write "V8"(FALSE) -> ()
                    n1421 = Wait (ms)(milliseconds to wait=1000) -> ()  [unwired: 1 out]
                  }
                  frame #13 {
                    # "Open V20"
                    n1422 = local write "V20"(TRUE) -> ()
                    n1423 = Wait (ms)(milliseconds to wait=1000) -> ()  [unwired: 1 out]
                  }
                  frame #14 {
                    # "When P < 0,076 torr continue w/ sequence"
                    n1424 = while {
                      shift-right: [w479] -> _
                      shift-left: _ -> [_]
                      stop <- w480 stop-if-true
                      n1425 = local read "Agilent (Torr)"() -> (w483:dbl)
                      n1426 = Wait (ms)(milliseconds to wait=100) -> ()  [unwired: 1 out]
                      n1427 = Less?(x=w483, y=0.076) -> (x < y?=w482:bool)
                      n1428 = case shown="True" w482 {
                        selector: w482 -> [w485 w487]
                        tunnel: [w485 w487] -> w479
                        frame False {
                        }
                        frame True {
                          n1429 = local write "Stop Pump Over"(TRUE) -> ()
                        }
                      }
                      n1430 = local read "Stop Pump Over"() -> (w480:bool)
                    }
                    n1431 = Wait (ms)(milliseconds to wait=1000) -> ()  [unwired: 1 out]
                  }
                  frame #15 {
                    n1432 = call "Prompt User for Input3"() -> ("OK"=w489:bool)  [unwired: 18 in, 1 out]
                    n1433 = local write "Stop Pump Over"(FALSE) -> ()
                  }
                  frame #16 {
                    # "30 sec to pump out capillary from cart to GB"
                    n1434 = Wait (ms)(milliseconds to wait=30000) -> ()  [unwired: 1 out]
                  }
                  frame #17 {
                    # "Dewar up"
                    n1435 = local write "D"(TRUE) -> ()
                    n1436 = Wait (ms)(milliseconds to wait=1000) -> ()  [unwired: 1 out]
                  }
                  frame #18 {
                    # "Give trap 15sec to cool down"
                    n1437 = Wait (ms)(milliseconds to wait=15000) -> ()  [unwired: 1 out]
                  }
                  frame #19 {
                    n1438 = call "Prompt User for Input4"() -> ("OK"=w494:bool)  [unwired: 18 in, 1 out]
                  }
                  frame #20 {
                    # "Should already be open"
                    # "Open V16 when GB ready to introduce"
                    n1439 = local write "V16"(TRUE) -> ()
                    n1440 = Wait (ms)(milliseconds to wait=1000) -> ()  [unwired: 1 out]
                  }
                  frame #21 {
                    # "Start GB sample introduction"
                    n1441 = local write "Inject GB"(TRUE) -> ()
                    n1442 = Wait (ms)(milliseconds to wait=5000) -> ()  [unwired: 1 out]
                  }
                  frame #22 {
                    # "Delay to allow you to make the needle transfer into the sample vial \nand to build He pressure back in GC in case dec. of pressure while \nneedle is out of vial causes atm to leak back in through Valco port 3"
                    n1443 = Wait (ms)(milliseconds to wait=60000) -> ()  [unwired: 1 out]
                  }
                  frame #23 {
                    # "40 min now"
                    # "Time delay for He carrier gas to flow through LN2 trap."
                    n1444 = call "Time Delay"() -> ()  [unwired: 11 in, 1 out]
                    n1445 = local write "Cryo-pull"(TRUE) -> ()
                    n1446 = Wait (ms)(milliseconds to wait=1000) -> ()  [unwired: 1 out]
                  }
                  frame #24 {
                    n1447 = local write "Inject GB"(FALSE) -> ()
                    n1448 = call "Prompt User for Input6"() -> ("OK"=w503:bool)  [unwired: 18 in, 1 out]
                    n1449 = Wait (ms)(milliseconds to wait=1000) -> ()  [unwired: 1 out]
                  }
                  frame #25 {
                    # "When P < 0,075 torr close off LN2 trap"
                    n1450 = call "Display Message to User5"() -> ()  [unwired: 10 in, 2 out]
                    n1451 = while {
                      shift-right: [w507] -> _
                      shift-left: _ -> [_]
                      stop <- w508 stop-if-true
                      n1452 = local read "Agilent (Torr)"() -> (w511:dbl)
                      n1453 = Wait (ms)(milliseconds to wait=100) -> ()  [unwired: 1 out]
                      n1454 = Less?(x=w511, y=0.075) -> (x < y?=w510:bool)
                      n1455 = case shown="True" w510 {
                        selector: w510 -> [w513 w515]
                        tunnel: [w513 w515] -> w507
                        frame False {
                        }
                        frame True {
                          n1456 = flat-sequence {
                            frame #0 {
                              n1457 = local write "V16"(FALSE) -> ()
                              n1458 = Wait (ms)(milliseconds to wait=100) -> ()  [unwired: 1 out]
                            }
                            frame #1 {
                              n1459 = local write "V17"(FALSE) -> ()
                              n1460 = Wait (ms)(milliseconds to wait=100) -> ()  [unwired: 1 out]
                            }
                            frame #2 {
                              n1461 = local write "V18"(FALSE) -> ()
                            }
                          }
                          n1462 = local write "Stop Pump Over"(TRUE) -> ()
                        }
                      }
                      n1463 = local read "Stop Pump Over"() -> (w508:bool)
                    }
                    n1464 = local write "Cryo-pull"(FALSE) -> ()
                    n1465 = Wait (ms)(milliseconds to wait=1000) -> ()  [unwired: 1 out]
                  }
                  frame #26 {
                    # "Dewar down"
                    n1466 = local write "D"(FALSE) -> ()
                    n1467 = local write "Stop Pump Over"(FALSE) -> ()
                    n1468 = Wait (ms)(milliseconds to wait=1000) -> ()  [unwired: 1 out]
                  }
                  frame #27 {
                    # "6 minute thaw"
                    n1469 = call "Time Delay2"() -> ()  [unwired: 11 in, 1 out]
                    n1470 = local write "Thawing"(TRUE) -> ()
                    n1471 = call "Display Message to User6"() -> ()  [unwired: 10 in, 2 out]
                  }
                  frame #28 {
                    n1472 = call "Display Message to User"() -> ()  [unwired: 10 in, 2 out]
                  }
                  frame #29 {
                    # "Read thaw P on Agilent - calculate umol CO2 trapped"
                    n1473 = local write "Thawing"(FALSE) -> ()
                    n1474 = flat-sequence {
                      frame #0 {
                        n1475 = local read "Agilent (Torr)"() -> (w528:dbl)
                        n1476 = local write "Thaw Yield (torr)"(w528) -> ()
                        n1477 = Wait (ms)(milliseconds to wait=200) -> ()  [unwired: 1 out]
                      }
                      frame #1 {
                        # "mol CO2"
                        # "''Cast base units''"
                        # "R"
                        # "V LN2, in m3"
                        # "torr to Pa"
                        n1478 = local read "Thaw Yield (torr)"() -> (w536:dbl)
                        n1479 = local read "Temp (K)"() -> (w529:dbl)
                        n1480 = Cast Unit Bases(0:dbl[unit] 8.3144598) -> (2:w530:dbl)  [unwired: 1 in]
                        n1481 = Multiply(x=w536, y=133.3223684211) -> (x*y=w535:dbl)
                        n1482 = Multiply(x=w530, y=w529) -> (x*y=w534:dbl)
                        n1483 = Multiply(x=w535, y=6.1e-05) -> (x*y=w540:dbl)
                        n1484 = Divide(x=w540, y=w534) -> (x/y=w533:dbl)
                        n1485 = Multiply(x=1000000.0, y=w533) -> (x*y=w531:dbl)
                        n1486 = local write "umol CO2"(w531) -> ()
                      }
                    }
                    n1487 = Wait (ms)(milliseconds to wait=500) -> ()  [unwired: 1 out]
                  }
                  frame #30 {
                    # "P for 400ppm"
                    # "22/4/22\nOffset \nfor extra\nN2 from \nloop"
                    # "Calculate and store Target P"
                    # "''Cast base units''"
                    # "R"
                    # "''Cast base units''"
                    # "R"
                    # "PV=nrt\nP - Pa\nV - m3\nn - mol\nR - \nT - K"
                    # "Pa to mbar"
                    # "P = nRT/V"
                    # "Pa"
                    # "mol N2 to dilute"
                    # "V LN2, flask, bellow in m3"
                    # "ppm"
                    # "n mol N2 = x mol CO2/0.000400"
                    # "0.000400 = x mol CO2/n mol N2"
                    # "mol CO2"
                    # "V LN2, in m3"
                    # "torr to Pa"
                    n1488 = local read "Thaw Yield (torr)"() -> (w545:dbl)
                    n1489 = local read "Temp (K)"() -> (w561:dbl)
                    n1490 = Subtract(x=w545, y=0.2) -> (x-y=w546:dbl)
                    n1491 = Cast Unit Bases(0:dbl[unit] 8.3144598) -> (2:w554:dbl)  [unwired: 1 in]
                    n1492 = Multiply(x=w546, y=133.3223684211) -> (x*y=w563:dbl)
                    n1493 = Multiply(x=w554, y=w561) -> (x*y=w562:dbl)
                    n1494 = Multiply(x=w563, y=6.1e-05) -> (x*y=w564:dbl)
                    n1495 = Divide(x=w564, y=w562) -> (x/y=w557:dbl)
                    n1496 = Divide(x=w557, y=0.0004) -> (x/y=w543:dbl)
                    n1497 = Cast Unit Bases(0:dbl[unit] 8.3144598) -> (2:w555:dbl)  [unwired: 1 in]
                    n1498 = local read "Temp (K)"() -> (w558:dbl)
                    n1499 = Multiply(x=w555, y=w543) -> (x*y=w559:dbl)
                    n1500 = Multiply(x=w558, y=w559) -> (x*y=w560:dbl)
                    n1501 = Divide(x=w560, y=0.000687) -> (x/y=w556:dbl)
                    n1502 = Multiply(x=0.01, y=w556) -> (x*y=w542:dbl)
                    n1503 = local write "Final Target P (mbar)"(w542) -> ()
                    n1504 = Wait (ms)(milliseconds to wait=200) -> ()  [unwired: 1 out]
                  }
                  frame #31 {
                    # "Calculate Dilution Target Pressure in prep for final expansion"
                    # "Dil. TP fills full MV, V17 closes\n101ml pumped away (all but flask)\n586ml @ Dil. TP expands to 687ml\n--> 687ml @ Final P (P for 400ppm)"
                    # "P1V1 = P2V2\nDTP*586ml = TFP*687ml\nDTP = (FP*687)/586"
                    n1505 = local read "Final Target P (mbar)"() -> (w569:dbl)
                    n1506 = Multiply(x=w569, y=687.0) -> (x*y=w568:dbl)
                    n1507 = Divide(x=w568, y=586.0) -> (x/y=w566:dbl)
                    n1508 = local write "Dil. Target P (mbar)"(w566) -> ()
                    n1509 = Wait (ms)(milliseconds to wait=200) -> ()  [unwired: 1 out]
                  }
                  frame #32 {
                    # "22/2/22\nAvg of n=2 1500 mbar auto test sloshes:\nn = 3E-6x^2 + 0,003x + 0,0254"
                    # "21/2/22\n1400 mbar auto test sloshes:\nn = 3E-6x^2 + 0,0033x + 0,0268\nn        x (P mbar)\n0        0\n1        232\n2        430\n3        569\n4        733\n5        847"
                    # "8/2/22\n1100 mbar manual sloshes:\nn = 1E-5x^2 + 0,0003x + 0,3052\nn        x (P mbar)\n0        0\n1        205\n2        345\n3        477\n4        587\n5        678\n6        755\n7        819\n8        872\n9        916\n10      951\n11      981"
                    n1510 = flat-sequence {
                      frame #0 {
                        # "Currently using avg curve for (Avg(Avg(1500x2),1400))\nn = 3E-6x^2 + 0.0031x + 0.0261"
                        # "Given Dilution Target Pressure, calculate how many sloshes it would take to get \nthe pressure in the full MV to that pressure."
                        n1511 = local read "Dil. Target P (mbar)"() -> (w582:dbl)
                        n1512 = local read "Dil. Target P (mbar)"() -> (w580:dbl)
                        n1513 = Square(x=w582) -> (x^2=w581:dbl)
                        n1514 = Multiply(x=3e-06, y=w581) -> (x*y=w578:dbl)
                        n1515 = Multiply(x=w580, y=0.0031) -> (x*y=w579:dbl)
                        n1516 = Add(x=w578, y=w579) -> (x+y=w577:dbl)
                        n1517 = Add(x=w577, y=0.0261) -> (x+y=w573:dbl)
                        n1518 = local write "Exact slosh"(w573) -> ()
                        n1519 = Wait (ms)(milliseconds to wait=100) -> ()  [unwired: 1 out]
                      }
                      frame #1 {
                        # "Now take that calculated number of \nsloshes and round down to nearest integer."
                        n1520 = local read "Exact slosh"() -> (w584:dbl)
                        n1521 = Round Toward -Infinity(1:w584) -> (0:w585:dbl)
                        n1522 = local write "Slosh to do"(w585) -> ()
                        n1523 = Wait (ms)(milliseconds to wait=100) -> ()  [unwired: 1 out]
                      }
                      frame #2 {
                        n1524 = local read "Exact slosh"() -> (w588:dbl)
                        n1525 = local read "Slosh to do"() -> (w587:dbl)
                        n1526 = Subtract(x=w588, y=w587) -> (x-y=w589:dbl)
                        n1527 = local write "Rem. slosh frac."(w589) -> ()
                        n1528 = Wait (ms)(milliseconds to wait=100) -> ()  [unwired: 1 out]
                      }
                      frame #3 {
                        n1529 = local read "Rem. slosh frac."() -> (w593:dbl)
                        n1530 = Multiply(x=1450.0, y=w593) -> (x*y=w592:dbl)
                        n1531 = local write "P frac. slosh"(w592) -> ()
                        n1532 = Wait (ms)(milliseconds to wait=100) -> ()  [unwired: 1 out]
                      }
                    }
                    n1533 = Wait (ms)(milliseconds to wait=200) -> ()  [unwired: 1 out]
                  }
                  frame #33 {
                    # "P should be something like 250mtor (V LN2 ~1/10 of V LN2 + flask)"
                    # "Open, Close V17 - pure CO2 expansion into flask\nEqual concentration of CO2 in LN2, flask, and H of V16/V17"
                    n1534 = flat-sequence {
                      frame #0 {
                        n1535 = local write "V17"(TRUE) -> ()
                      }
                      frame #1 {
                        n1536 = Wait (ms)(milliseconds to wait=u32 40000) -> ()  [unwired: 1 out]
                      }
                      frame #2 {
                        n1537 = local write "V17"(FALSE) -> ()
                      }
                    }
                    n1538 = Wait (ms)(milliseconds to wait=1000) -> ()  [unwired: 1 out]
                  }
                  frame #34 {
                    # "Close V20"
                    n1539 = local write "V20"(FALSE) -> ()
                    n1540 = Wait (ms)(milliseconds to wait=1000) -> ()  [unwired: 1 out]
                  }
                  frame #35 {
                    # "Open V8 - begin dilution steps"
                    n1541 = local write "Diluting"(TRUE) -> ()
                    n1542 = local write "V8"(TRUE) -> ()
                    n1543 = Wait (ms)(milliseconds to wait=1000) -> ()  [unwired: 1 out]
                  }
                  frame #36 {
                    # "Open V21"
                    n1544 = local write "V21"(TRUE) -> ()
                    n1545 = Wait (ms)(milliseconds to wait=1000) -> ()  [unwired: 1 out]
                  }
                  frame #37 {
                    # "Build P in bellow before introducing to LN2 trap w/ sample"
                    n1546 = call "Pressurize in LN28"() -> ()  [unwired: 11 in, 1 out]
                  }
                  frame #38 {
                    # "Open V18"
                    n1547 = local write "V18"(TRUE) -> ()
                    n1548 = Wait (ms)(milliseconds to wait=1000) -> ()  [unwired: 1 out]
                  }
                  frame #39 {
                    n1549 = local read "Slosh to do"() -> (w607:dbl)
                    n1550 = for {
                      N: w607 -> [_]
                      n1551 = flat-sequence {
                        frame #0 {
                          n1552 = while {
                            shift-right: [w609] -> _
                            shift-left: _ -> [_]
                            stop <- w610 stop-if-true
                            # "Greater difference in P causes more \nturbulent mixing when expanded into flask"
                            # "When P in bellow + LN2 is > 1450mbar, Open V17"
                            n1553 = local read "Pressure (mbar)"() -> (w612:dbl)
                            n1554 = Wait (ms)(milliseconds to wait=100) -> ()  [unwired: 1 out]
                            n1555 = Greater?(x=w612, y=1450.0) -> (0:w613:bool)
                            n1556 = case shown="True" w613 {
                              selector: w613 -> [w614 w616]
                              tunnel: [w614 w616] -> w609
                              frame False {
                              }
                              frame True {
                                n1557 = local write "Stop Sample Pressure"(TRUE) -> ()
                                n1558 = local write "V17"(TRUE) -> ()
                              }
                            }
                            n1559 = local read "Stop Sample Pressure"() -> (w610:bool)
                          }
                        }
                        frame #1 {
                          n1560 = local read "No. Slosh"() -> (w618:dbl)
                          n1561 = local write "Stop Sample Pressure"(FALSE) -> ()
                          n1562 = Increment(x=w618) -> (x+1=w619:dbl)
                          n1563 = Wait (ms)(milliseconds to wait=4000) -> ()  [unwired: 1 out]
                          n1564 = local write "No. Slosh"(w619) -> ()
                        }
                        frame #2 {
                          n1565 = local read "Pressure (mbar)"() -> (w622:dbl)
                          n1566 = local write "Slosh P (mbar)"(w622) -> ()
                          n1567 = Wait (ms)(milliseconds to wait=1000) -> ()  [unwired: 1 out]
                        }
                        frame #3 {
                          n1568 = local write "V17"(FALSE) -> ()
                          n1569 = Wait (ms)(milliseconds to wait=1000) -> ()  [unwired: 1 out]
                        }
                      }
                    }
                  }
                  frame #40 {
                    # "Check that the final fractional slosh P \nwill be greater P than what's in the \nflask already. If yes, do fractional slosh; \nif no, skip it and go straight to diluting to DTP."
                    n1570 = local read "Slosh P (mbar)"() -> (w626:dbl)
                    n1571 = local read "P frac. slosh"() -> (w627:dbl)
                    n1572 = Greater Or Equal?(x=w627, y=w626) -> (x >= y?=w628:bool)
                    n1573 = case shown="True" w628 {
                      frame False {
                        # "Open V17"
                        n1574 = local write "V17"(TRUE) -> ()
                        n1575 = local read "Dil. Target P (mbar)"() -> (w630:dbl)
                        n1576 = local read "Slosh P (mbar)"() -> (w629:dbl)
                        n1577 = Divide(x=w629, y=w630) -> (x/y=w633:dbl)
                        n1578 = Multiply(x=w633, y=100.0) -> (x*y=w631:dbl)
                        n1579 = local write "Slosh acc. %"(w631) -> ()
                        n1580 = Wait (ms)(milliseconds to wait=1000) -> ()  [unwired: 1 out]
                      }
                      frame True {
                        # "Last slosh into flask, keep V17 open so dilution loop can start right after"
                        n1581 = flat-sequence {
                          frame #0 {
                            n1582 = local read "Rem. slosh frac."() -> (w638:dbl)
                            n1583 = local read "No. Slosh"() -> (w639:dbl)
                            n1584 = Wait (ms)(milliseconds to wait=100) -> ()  [unwired: 1 out]
                            n1585 = Add(x=w639, y=w638) -> (x+y=w637:dbl)
                            n1586 = local write "Slosh to do"(w637) -> ()
                          }
                          frame #1 {
                            n1587 = while {
                              shift-right: [w642] -> _
                              shift-left: _ -> [_]
                              stop <- w644 stop-if-true
                              # "When P in bellow + LN2 is > fractional slosh P, Open V17"
                              n1588 = local read "Pressure (mbar)"() -> (w645:dbl)
                              n1589 = local read "P frac. slosh"() -> (w640:dbl)
                              n1590 = Wait (ms)(milliseconds to wait=100) -> ()  [unwired: 1 out]
                              n1591 = Greater Or Equal?(x=w645, y=w640) -> (x >= y?=w643:bool)
                              n1592 = case shown="True" w643 {
                                selector: w643 -> [w646 w647]
                                tunnel: [w646 w647] -> w642
                                frame False {
                                }
                                frame True {
                                n1593 = local write "Stop Sample Pressure"(TRUE) -> ()
                                n1594 = local write "V17"(TRUE) -> ()
                                }
                              }
                              n1595 = local read "Stop Sample Pressure"() -> (w644:bool)
                            }
                          }
                          frame #2 {
                            n1596 = local read "Rem. slosh frac."() -> (w650:dbl)
                            n1597 = local read "No. Slosh"() -> (w651:dbl)
                            n1598 = local write "Stop Sample Pressure"(FALSE) -> ()
                            n1599 = Add(x=w651, y=w650) -> (x+y=w652:dbl)
                            n1600 = Wait (ms)(milliseconds to wait=5000) -> ()  [unwired: 1 out]
                            n1601 = local write "No. Slosh"(w652) -> ()
                          }
                          frame #3 {
                            n1602 = local read "Pressure (mbar)"() -> (w655:dbl)
                            n1603 = local write "Slosh P (mbar)"(w655) -> ()
                            n1604 = Wait (ms)(milliseconds to wait=500) -> ()  [unwired: 1 out]
                          }
                          frame #4 {
                            n1605 = local read "Slosh P (mbar)"() -> (w658:dbl)
                            n1606 = local read "Dil. Target P (mbar)"() -> (w659:dbl)
                            n1607 = Divide(x=w658, y=w659) -> (x/y=w662:dbl)
                            n1608 = Multiply(x=w662, y=100.0) -> (x*y=w660:dbl)
                            n1609 = local write "Slosh acc. %"(w660) -> ()
                            n1610 = Wait (ms)(milliseconds to wait=200) -> ()  [unwired: 1 out]
                          }
                        }
                      }
                    }
                  }
                  frame #41 {
                    # "Dil. TP fills full MV, V17 closes\n101ml pumped away (all but flask)\n586ml @ Dil. TP expands to 687ml\n--> 687ml @ Final P (P for 400ppm)"
                    # "Agilent P comes through the DAQ"
                    # "When P Wika = maths for 400ppm dilution, close V8"
                    n1611 = local read "Dil. Target P (mbar)"() -> (w664:dbl)
                    n1612 = local read "Pressure (mbar)"() -> (w665:dbl)
                    n1613 = Greater?(x=w664, y=w665) -> (0:w666:bool)
                    n1614 = case shown="True" w666 {
                      frame False {
                        n1615 = local write "V17"(FALSE) -> ()
                        n1616 = local write "V8"(FALSE) -> ()
                        n1617 = call "Display Message to User2"() -> ()  [unwired: 10 in, 2 out]
                      }
                      frame True {
                        n1618 = while {
                          shift-right: [w670] -> _
                          shift-left: _ -> [_]
                          i -> [w680]
                          stop <- w681 stop-if-true
                          n1619 = local read "Dil. Target P (mbar)"() -> (w678:dbl)
                          n1620 = local write "Dil. i"(w680) -> ()
                          n1621 = local read "Pressure (mbar)"() -> (w677:dbl)
                          n1622 = local read "Pressure (mbar)"() -> (w675:dbl)
                          n1623 = Add(x=w675, y=2.0) -> (x+y=w674:dbl)
                          n1624 = Subtract(x=w677, y=2.0) -> (x-y=w673:dbl)
                          n1625 = Wait (ms)(milliseconds to wait=u32 100) -> ()  [unwired: 1 out]
                          n1626 = In Range and Coerce(upper limit=w674, x=w678, lower limit=w673) -> (coerced(x)=w669:dbl, In Range?=w676:bool)
                          n1627 = local write "Dilution P (mbar)"(w669) -> ()
                          n1628 = case shown="True" w676 {
                            selector: w676 -> [w682 w686]
                            tunnel: [w682 w686] -> w670
                            frame False {
                            }
                            frame True {
                              n1629 = local write "V8"(FALSE) -> ()
                              n1630 = local write "Stop Dilution"(TRUE) -> ()
                              n1631 = local write "V17"(FALSE) -> ()
                            }
                          }
                          n1632 = local read "Stop Dilution"() -> (w681:bool)
                        }
                      }
                    }
                    n1633 = Wait (ms)(milliseconds to wait=1000) -> ()  [unwired: 1 out]
                  }
                  frame #42 {
                    # "Close V21 - N2 inlet - want to keep this volume under superambient pressure always"
                    # "Flask will be over concentrated in CO2 (hopefully somewhere around 480ppm - cant really check that so it's blind)\n19/1/22, 8:00 - Initial manual test of this measured 472ppm on the Licor. Sample expansion and re-dilution that\nfollowed diluted the sample to 397ppm."
                    n1634 = local write "Stop Dilution"(FALSE) -> ()
                    n1635 = local write "Diluting"(FALSE) -> ()
                    n1636 = local write "V21"(FALSE) -> ()
                    n1637 = Wait (ms)(milliseconds to wait=1000) -> ()  [unwired: 1 out]
                  }
                  frame #43 {
                    # "Open V20 - pump out bellow + LN2 trap"
                    n1638 = local write "V20"(TRUE) -> ()
                    n1639 = Wait (ms)(milliseconds to wait=1000) -> ()  [unwired: 1 out]
                  }
                  frame #44 {
                    # "Should already be open anyways"
                    # "Open V18 - pump out bellow + LN2 trap"
                    n1640 = local write "V18"(TRUE) -> ()
                    n1641 = Wait (ms)(milliseconds to wait=1000) -> ()  [unwired: 1 out]
                  }
                  frame #45 {
                    # "Pump excess N2 out from LN2, bellow for 2min"
                    n1642 = call "Time Delay3"() -> ()  [unwired: 11 in, 1 out]
                  }
                  frame #46 {
                    # "Close V20"
                    n1643 = local write "V20"(FALSE) -> ()
                    n1644 = Wait (ms)(milliseconds to wait=1000) -> ()  [unwired: 1 out]
                  }
                  frame #47 {
                    # "Open V17 - expand flask back into LN2 and bellow volume"
                    n1645 = local write "V17"(TRUE) -> ()
                    n1646 = Wait (ms)(milliseconds to wait=15000) -> ()  [unwired: 1 out]
                  }
                  frame #48 {
                    n1647 = local read "Pressure (mbar)"() -> (w701:dbl)
                    n1648 = call "Convert from Dynamic Data3"("Dynamic Data Type"=w701) -> ("Array"=w702:dbl[])  [unwired: 3 in]
                    n1649 = call-poly <vilib>:"Mean.vi"("X"=w702) -> ("mean"=w700:dbl)  [unwired: 1 out]
                    n1650 = local write "Final P (mbar)"(w700) -> ()
                    n1651 = Wait (ms)(milliseconds to wait=200) -> ()  [unwired: 1 out]
                  }
                  frame #49 {
                    n1652 = local read "Final Target P (mbar)"() -> (w707:dbl)
                    n1653 = local read "Final P (mbar)"() -> (w708:dbl)
                    n1654 = Divide(x=w708, y=w707) -> (x/y=w706:dbl)
                    n1655 = Multiply(x=w706, y=100.0) -> (x*y=w705:dbl)
                    n1656 = local write "Final P Accuracy (%)"(w705) -> ()
                    n1657 = Wait (ms)(milliseconds to wait=200) -> ()  [unwired: 1 out]
                  }
                  frame #50 {
                    # "Open V16"
                    n1658 = local write "V16"(TRUE) -> ()
                    n1659 = Wait (ms)(milliseconds to wait=1000) -> ()  [unwired: 1 out]
                  }
                  frame #51 {
                    # "Activate circulation loop"
                    n1660 = local write "Circulation Loop"(TRUE) -> ()
                    n1661 = call "Prompt User for Input7"() -> ("OK"=w712:bool)  [unwired: 18 in, 1 out]
                    n1662 = Wait (ms)(milliseconds to wait=1000) -> ()  [unwired: 1 out]
                  }
                  frame #52 {
                    # "currently 2,5min"
                    # "Time delay for circulation/mixing"
                    n1663 = call "Time Delay6"() -> ()  [unwired: 11 in, 1 out]
                  }
                  frame #53 {
                    n1664 = call "Prompt User for Input8"() -> ("OK"=w714:bool)  [unwired: 18 in, 1 out]
                  }
                  frame #54 {
                    # "Close V16"
                    # "Stop circulation"
                    n1665 = local write "Circulation Loop"(FALSE) -> ()
                    n1666 = local write "V16"(FALSE) -> ()
                    n1667 = Wait (ms)(milliseconds to wait=1000) -> ()  [unwired: 1 out]
                  }
                  frame #55 {
                    n1668 = local write "GO!!!!"(FALSE) -> ()
                    n1669 = local write "Start Sequence"(FALSE) -> ()
                    n1670 = local write "Carbonate Sam"(FALSE) -> ()
                    n1671 = local write "Seq. Finished"(TRUE) -> ()
                  }
                }
              }
            }
          }
        }
      }
    }
    n1672 = Wait (ms)(milliseconds to wait=u32 49) -> ()  [unwired: 1 out]
    n1673 = local read "End Program"() -> (w71:bool)
  }
  n1674 = while {
    shift-right: [w1647] -> w19
    shift-left: w23 -> [w1744]
    shift-right: [w1649] -> w20
    shift-left: w22 -> [w1743]
    stop <- "End Program" stop-if-true
    # "Add 50mV for \nhorizontal mount"
    # "14/01/22 - Calibrating Wika V to Licor P (kPa)\ny = 400,17x - 7,5512   ->  mbar = 400,17(V) - 7,5512\nV              kPa          mbar\n1,522       60            600\n1.767       70            700\n1.893       75            750\n2.019       80            800\n2.143       85            850\n2.267       90            900\n2.391       95            950\n2.516       100          100"
    # "List of proper DO channel values: \nV1 - 4\nV2 - 2\nV3 - 3\nV4 - 7\nV5 - 5\nV6 - 6\nV7 - 13\nV8 - 10\nDewar - 11\nV16 - 8\nV17 - 15\nV18 - 14\nV19 - 12\nV20 - 17\nV21 - 16\nCirculation Loop - 9"
    # "Okay so sometimes, for some unknown reason, the ID values for the valve DO channels change. Specifically, V17 & V21 buttons switch values. Also, \nthe Shunt+Pump button takes on the value 17, which is used by V20. The correct values are V17 - 15, V21 - 16, Shunt+Pump -9 but sometimes they flip-flop. \nIt seems that the values switch usually after powering down the computer. Have to pay more attention to if they change even just when closing LV and \nre-opening it, or if it changes after being closed for some period of time."
    n1675 = Get Date/Time In Seconds() -> (seconds since 1Jan1904=→"Current Time":timestamp)
    n1676 = Wait (ms)(milliseconds to wait=u32 10) -> ()  [unwired: 1 out]
    n1677 = Not(x="V2") -> (.not. x?=w1673:bool)
    n1678 = call-poly <vilib>:"Digital Write.vi"("Error In"=w1744, "Output Value"=w1673, "DO Channel"="Valve 2", "LINX Resource"=w1743) -> ("Error Out"=w1726:errorcluster, "LINX Resource"=w1725:T1)  [unwired: 6 in]
    n1679 = Not(x="V3") -> (.not. x?=w1676:bool)
    n1680 = call "DAQ Assistant"("stop (F)"="stop (F)") -> ("data"=w1668:dynamicdata)  [unwired: 15 in, 3 out]
    n1681 = call-poly <vilib>:"Digital Write.vi"("Error In"=w1726, "Output Value"=w1676, "DO Channel"="Valve 3", "LINX Resource"=w1725) -> ("Error Out"=w1727:errorcluster, "LINX Resource"=w1724:T1)  [unwired: 6 in]
    n1682 = Split Signals(w1668) -> (w1660:dynamicdata, w1656:dynamicdata)  [unwired: 2 in]
    n1683 = Not(x="V1") -> (.not. x?=w1678:bool)
    n1684 = call "Convert from Dynamic Data2"("Dynamic Data Type"=w1656) -> ("Array"=w1662:dbl[])  [unwired: 3 in]
    n1685 = call-poly <vilib>:"Digital Write.vi"("Error In"=w1727, "Output Value"=w1678, "DO Channel"="Valve 1", "LINX Resource"=w1724) -> ("Error Out"=w1728:errorcluster, "LINX Resource"=w1723:T1)  [unwired: 6 in]
    n1686 = call-poly <vilib>:"Mean.vi"("X"=w1662) -> ("mean"=→"V":dbl)  [unwired: 1 out]
    n1687 = Multiply(x=w1656, y=400.17) -> (x*y=w1664:dynamicdata)
    n1688 = Add(x=w1660, y=0.05) -> (x+y=→"?" →"Agilent" →"Agilent (Torr)":dynamicdata)
    n1689 = Not(x="V5") -> (.not. x?=w1681:bool)
    n1690 = Subtract(x=w1664, y=7.5512) -> (x-y=w1663:dynamicdata)
    "Wika (Avg)" <- w1663
    n1691 = call-poly <vilib>:"Digital Write.vi"("Error In"=w1728, "Output Value"=w1681, "DO Channel"="Valve 5", "LINX Resource"=w1723) -> ("Error Out"=w1729:errorcluster, "LINX Resource"=w1722:T1)  [unwired: 6 in]
    n1692 = call "Convert from Dynamic Data"("Dynamic Data Type"=w1663) -> ("Array"=w1666:dbl[])  [unwired: 3 in]
    n1693 = Not(x="V6") -> (.not. x?=w1684:bool)
    n1694 = call-poly <vilib>:"Mean.vi"("X"=w1666) -> ("mean"=→"?" →"Pressure (mbar)":dbl)  [unwired: 1 out]
    n1695 = call-poly <vilib>:"Digital Write.vi"("Error In"=w1729, "Output Value"=w1684, "DO Channel"="Valve 6", "LINX Resource"=w1722) -> ("Error Out"=w1730:errorcluster, "LINX Resource"=w1721:T1)  [unwired: 6 in]
    n1696 = Not(x="V4") -> (.not. x?=w1687:bool)
    n1697 = call-poly <vilib>:"Digital Write.vi"("Error In"=w1730, "Output Value"=w1687, "DO Channel"="Valve 4", "LINX Resource"=w1721) -> ("Error Out"=w1731:errorcluster, "LINX Resource"=w1720:T1)  [unwired: 6 in]
    n1698 = Not(x="V16") -> (.not. x?=w1690:bool)
    n1699 = call-poly <vilib>:"Digital Write.vi"("Error In"=w1731, "Output Value"=w1690, "DO Channel"="Valve 16", "LINX Resource"=w1720) -> ("Error Out"=w1742:errorcluster, "LINX Resource"=w1741:T1)  [unwired: 6 in]
    n1700 = Not(x="V8") -> (.not. x?=w1693:bool)
    n1701 = call-poly <vilib>:"Digital Write.vi"("Error In"=w1742, "Output Value"=w1693, "DO Channel"="Valve 8", "LINX Resource"=w1741) -> ("Error Out"=w1732:errorcluster, "LINX Resource"=w1719:T1)  [unwired: 6 in]
    n1702 = Not(x="D") -> (.not. x?=w1696:bool)
    n1703 = call-poly <vilib>:"Digital Write.vi"("Error In"=w1732, "Output Value"=w1696, "DO Channel"="Dewar", "LINX Resource"=w1719) -> ("Error Out"=w1733:errorcluster, "LINX Resource"=w1718:T1)  [unwired: 6 in]
    n1704 = Not(x="V19") -> (.not. x?=w1698:bool)
    n1705 = call-poly <vilib>:"Digital Write.vi"("Error In"=w1733, "Output Value"=w1698, "DO Channel"="Valve 19", "LINX Resource"=w1718) -> ("Error Out"=w1734:errorcluster, "LINX Resource"=w1717:T1)  [unwired: 6 in]
    n1706 = Not(x="V7") -> (.not. x?=w1701:bool)
    n1707 = call-poly <vilib>:"Digital Write.vi"("Error In"=w1734, "Output Value"=w1701, "DO Channel"="Valve 7", "LINX Resource"=w1717) -> ("Error Out"=w1735:errorcluster, "LINX Resource"=w1716:T1)  [unwired: 6 in]
    n1708 = Not(x="V18") -> (.not. x?=w1704:bool)
    n1709 = call-poly <vilib>:"Digital Write.vi"("Error In"=w1735, "Output Value"=w1704, "DO Channel"="Valve 18", "LINX Resource"=w1716) -> ("Error Out"=w1736:errorcluster, "LINX Resource"=w1715:T1)  [unwired: 6 in]
    n1710 = Not(x="V17") -> (.not. x?=w1655:bool)
    n1711 = call-poly <vilib>:"Digital Write.vi"("Error In"=w1736, "Output Value"=w1655, "DO Channel"="Valve 17", "LINX Resource"=w1715) -> ("Error Out"=w1737:errorcluster, "LINX Resource"=w1714:T1)  [unwired: 6 in]
    n1712 = Not(x="V21") -> (.not. x?=w1654:bool)
    n1713 = call-poly <vilib>:"Digital Write.vi"("Error In"=w1737, "Output Value"=w1654, "DO Channel"="Valve 21", "LINX Resource"=w1714) -> ("Error Out"=w1713:errorcluster, "LINX Resource"=w1712:T1)  [unwired: 6 in]
    n1714 = Not(x="V20") -> (.not. x?=w1711:bool)
    n1715 = call-poly <vilib>:"Digital Write.vi"("Error In"=w1713, "Output Value"=w1711, "DO Channel"="Valve 20", "LINX Resource"=w1712) -> ("Error Out"=w1648:errorcluster, "LINX Resource"=w1650:T1)  [unwired: 6 in]
    n1716 = Not(x="Circulation Loop") -> (.not. x?=w1653:bool)
    n1717 = call-poly <vilib>:"Digital Write.vi"("Error In"=w1648, "Output Value"=w1653, "DO Channel"="Circulation Loop", "LINX Resource"=w1650) -> ("Error Out"=w1647:errorcluster, "LINX Resource"=w1649:T1)  [unwired: 6 in]
  }
  n1718 = call <vilib>:"Close.vi"("Error In"=w19, "LINX Resource"=w20) -> ("Error Out"=w21:errorcluster)  [unwired: 9 in]
  n1719 = call <vilib>:"Simple Error Handler.vi"("error in (no error)"=w21) -> ()  [unwired: 4 in, 5 out]
  n1720 = control-ref of="Test"() -> (w6:refnum<vi>)
  n1721 = Unregister For Events(event registration refnum=w11, error in=w10) -> (error out=w14:errorcluster)
  n1722 = call <vilib>:"Simple Error Handler.vi"("error in (no error)"=w14) -> ()  [unwired: 4 in, 5 out]
  n1723 = register-events(w6) -> (reference out=w5:refnum<event-registration>, error out=w1:errorcluster)  [unwired: 2 in]
  n1724 = while {
    tunnel: w5 -> [w1747]
    tunnel: [w1746] -> w3
    tunnel: [w1745] -> w2
    tunnel: w1 -> [w1745]
    stop <- w1748 stop-if-true
    n1725 = event shown="[0] \"Test\": Value Change" {
      selector: w1747 -> [_]
      dyn-events: [_] -> w1746
      timeout: _ -> [_]
      event "Test": Value Change {
        n1726 = event-data() -> ()  [unwired: 1 in, 6 out]
        n1727 = flat-sequence {
          frame #0 {
            n1728 = Wait (ms)(milliseconds to wait=1000) -> ()  [unwired: 1 out]
            n1729 = local write "V8"(TRUE) -> ()
          }
          frame #1 {
            n1730 = local write "V21"(TRUE) -> ()
            n1731 = Wait (ms)(milliseconds to wait=1000) -> ()  [unwired: 1 out]
          }
          frame #2 {
            n1732 = for {
              N: 0.0 -> [_]
              n1733 = flat-sequence {
                frame #0 {
                  n1734 = while {
                    shift-right: [w1755] -> _
                    shift-left: _ -> [_]
                    stop <- w1759 stop-if-true
                    n1735 = local read "Pressure (mbar)"() -> (w1757:dbl)
                    n1736 = Wait (ms)(milliseconds to wait=100) -> ()  [unwired: 1 out]
                    n1737 = Greater?(x=w1757, y=800.0) -> (0:w1756:bool)
                    n1738 = case shown="True" w1756 {
                      selector: w1756 -> [w1760 w1761]
                      tunnel: [w1760 w1761] -> w1755
                      frame False {
                      }
                      frame True {
                        n1739 = local write "Stop Sample Pressure"(TRUE) -> ()
                        n1740 = local write "V17"(TRUE) -> ()
                      }
                    }
                    n1741 = local read "Stop Sample Pressure"() -> (w1759:bool)
                  }
                }
                frame #1 {
                  n1742 = local write "Stop Sample Pressure"(FALSE) -> ()
                  n1743 = local read "No. Slosh"() -> (w1764:dbl)
                  n1744 = Increment(x=w1764) -> (x+1=w1765:dbl)
                  n1745 = local write "No. Slosh"(w1765) -> ()
                  n1746 = Wait (ms)(milliseconds to wait=2000) -> ()  [unwired: 1 out]
                }
                frame #2 {
                  n1747 = Wait (ms)(milliseconds to wait=1000) -> ()  [unwired: 1 out]
                }
                frame #3 {
                  n1748 = local write "V17"(FALSE) -> ()
                  n1749 = Wait (ms)(milliseconds to wait=1000) -> ()  [unwired: 1 out]
                }
              }
            }
          }
          frame #3 {
            n1750 = for {
              N: 0.0 -> [_]
              n1751 = flat-sequence {
                frame #0 {
                  n1752 = while {
                    shift-right: [w1776] -> _
                    shift-left: _ -> [_]
                    stop <- w1777 stop-if-true
                    n1753 = local read "Pressure (mbar)"() -> (w1774:dbl)
                    n1754 = Wait (ms)(milliseconds to wait=100) -> ()  [unwired: 1 out]
                    n1755 = Greater?(x=w1774, y=1100.0) -> (0:w1773:bool)
                    n1756 = case shown="True" w1773 {
                      selector: w1773 -> [w1778 w1781]
                      tunnel: [w1778 w1781] -> w1776
                      frame False {
                      }
                      frame True {
                        n1757 = local write "Stop Sample Pressure"(TRUE) -> ()
                        n1758 = local write "V17"(TRUE) -> ()
                      }
                    }
                    n1759 = local read "Stop Sample Pressure"() -> (w1777:bool)
                  }
                }
                frame #1 {
                  n1760 = local write "Stop Sample Pressure"(FALSE) -> ()
                  n1761 = local read "No. Slosh"() -> (w1785:dbl)
                  n1762 = Increment(x=w1785) -> (x+1=w1784:dbl)
                  n1763 = local write "No. Slosh"(w1784) -> ()
                  n1764 = Wait (ms)(milliseconds to wait=2000) -> ()  [unwired: 1 out]
                }
                frame #2 {
                  n1765 = Wait (ms)(milliseconds to wait=1000) -> ()  [unwired: 1 out]
                }
                frame #3 {
                  n1766 = local write "V17"(FALSE) -> ()
                  n1767 = Wait (ms)(milliseconds to wait=1000) -> ()  [unwired: 1 out]
                }
              }
            }
          }
          frame #4 {
            n1768 = for {
              N: 0.0 -> [_]
              n1769 = flat-sequence {
                frame #0 {
                  n1770 = while {
                    shift-right: [w1794] -> _
                    shift-left: _ -> [_]
                    stop <- w1795 stop-if-true
                    n1771 = local read "Pressure (mbar)"() -> (w1792:dbl)
                    n1772 = Wait (ms)(milliseconds to wait=100) -> ()  [unwired: 1 out]
                    n1773 = Greater?(x=w1792, y=1300.0) -> (0:w1791:bool)
                    n1774 = case shown="True" w1791 {
                      selector: w1791 -> [w1796 w1799]
                      tunnel: [w1796 w1799] -> w1794
                      frame False {
                      }
                      frame True {
                        n1775 = local write "Stop Sample Pressure"(TRUE) -> ()
                        n1776 = local write "V17"(TRUE) -> ()
                      }
                    }
                    n1777 = local read "Stop Sample Pressure"() -> (w1795:bool)
                  }
                }
                frame #1 {
                  n1778 = local write "Stop Sample Pressure"(FALSE) -> ()
                  n1779 = local read "No. Slosh"() -> (w1802:dbl)
                  n1780 = Increment(x=w1802) -> (x+1=w1803:dbl)
                  n1781 = local write "No. Slosh"(w1803) -> ()
                  n1782 = Wait (ms)(milliseconds to wait=2000) -> ()  [unwired: 1 out]
                }
                frame #2 {
                  n1783 = Wait (ms)(milliseconds to wait=1000) -> ()  [unwired: 1 out]
                }
                frame #3 {
                  n1784 = local write "V17"(FALSE) -> ()
                  n1785 = Wait (ms)(milliseconds to wait=1000) -> ()  [unwired: 1 out]
                }
              }
            }
          }
          frame #5 {
            n1786 = for {
              N: 5.0 -> [_]
              n1787 = flat-sequence {
                frame #0 {
                  n1788 = while {
                    shift-right: [w1812] -> _
                    shift-left: _ -> [_]
                    stop <- w1813 stop-if-true
                    n1789 = local read "Pressure (mbar)"() -> (w1809:dbl)
                    n1790 = Wait (ms)(milliseconds to wait=100) -> ()  [unwired: 1 out]
                    n1791 = Greater?(x=w1809, y=1500.0) -> (0:w1811:bool)
                    n1792 = case shown="True" w1811 {
                      selector: w1811 -> [w1814 w1815]
                      tunnel: [w1814 w1815] -> w1812
                      frame False {
                      }
                      frame True {
                        n1793 = local write "Stop Sample Pressure"(TRUE) -> ()
                        n1794 = local write "V17"(TRUE) -> ()
                      }
                    }
                    n1795 = local read "Stop Sample Pressure"() -> (w1813:bool)
                  }
                }
                frame #1 {
                  n1796 = local write "Stop Sample Pressure"(FALSE) -> ()
                  n1797 = local read "No. Slosh"() -> (w1820:dbl)
                  n1798 = Increment(x=w1820) -> (x+1=w1821:dbl)
                  n1799 = local write "No. Slosh"(w1821) -> ()
                  n1800 = Wait (ms)(milliseconds to wait=2000) -> ()  [unwired: 1 out]
                }
                frame #2 {
                  n1801 = Wait (ms)(milliseconds to wait=1000) -> ()  [unwired: 1 out]
                }
                frame #3 {
                  n1802 = local write "V17"(FALSE) -> ()
                  n1803 = Wait (ms)(milliseconds to wait=1000) -> ()  [unwired: 1 out]
                }
              }
            }
          }
          frame #6 {
          }
          frame #7 {
          }
          frame #8 {
          }
          frame #9 {
            n1804 = local write "V21"(FALSE) -> ()
            n1805 = Wait (ms)(milliseconds to wait=1000) -> ()  [unwired: 1 out]
          }
          frame #10 {
            n1806 = local write "V8"(FALSE) -> ()
            n1807 = Wait (ms)(milliseconds to wait=1000) -> ()  [unwired: 1 out]
          }
        }
      }
    }
    n1808 = local read "End Program"() -> (w1748:bool)
  }
  n1809 = Unregister For Events(event registration refnum=w3, error in=w2) -> (error out=w4:errorcluster)
  n1810 = call <vilib>:"Simple Error Handler.vi"("error in (no error)"=w4) -> ()  [unwired: 4 in, 5 out]
